vi "justin arc - v1.vi"() -> ()   [LabVIEW 2019]
doc: "This is the interface, the one VI which loads all the others. Run this one first.\n\n(the line below ensures settings are saved)\n[Red Tweezers Save Settings]"
uses:
  justin arc - v1 Folder/Matt Fall 2018 files/Matt working/Red Tweezers Image Processing Final 1-19/subvis/line_trapping.ctl
  justin arc - v1 Folder/Matt Fall 2018 files/Matt working/Red Tweezers Image Processing Final 1-19/subvis/spot.ctl
  <vilib>/userDefined/High Color/IMAQdx.ctl
  justin arc - v1 Folder/Matt Fall 2018 files/Matt working/Red Tweezers Image Processing Final 1-19/subvis/selection_element.ctl
  <vilib>/Analysis/Matrix/Datatypes/RealMatrix.ctl
  justin arc - v1 Folder/Matt Fall 2018 files/Matt working/Red Tweezers Image Processing Final 1-19/subvis/mouse_info.ctl
  <vilib>/Analysis/baseanly.llb/Real A x B.vi
  justin arc - v1 Folder/Matt Fall 2018 files/Matt working/Red Tweezers Image Processing Final 1-19/subvis/red_tweezers_globals_INTERNAL_VOLATILE.vi
  justin arc - v1 Folder/Matt Fall 2018 files/Matt working/Red Tweezers Image Processing Final 1-19/subvis/red_tweezers_globals.vi
  <vilib>/Analysis/Matrix/Numeric/Multiply/Multiply - RM,R.vi
  <vilib>/Analysis/Matrix/Numeric/Multiply/Multiply - R,RM.vi
  <vilib>/Analysis/NI_AALBase.lvlib
  <vilib>/vision/driver/NI_Vision_Acquisition_Software.lvlib
  <vilib>/vision/NI_Vision_Development_Module.lvlib
  <vilib>/Analysis/Matrix/NI_Matrix.lvlib
panel:
  out "Specific Point":cluster{i32, i32}
  out "bottomrx 3":dbl
  out "toply 3":dbl
  out "bottomry 3":dbl
  out "toplx 3":dbl
  out "Circles 2":T1(array[cluster]) {"Position"."Y" format="%.2f"; "Position"."X" format="%.2f"}
  out "Spot Storage":T2[](array[typedef]) {"Amplitude Correction" step=0.1; "Line Trapping"."Phase Gradient" step=0.05; "Line Trapping"."Vector"."x" step=1e-06 format="%#_6p"; "Line Trapping"."Vector"."y" step=1e-06 format="%#_6p"; "Line Trapping"."Vector"."z" step=1e-06 format="%#_6p"; "NA Position"."r" step=1e-06; "NA Position"."y" step=1e-06; "NA Position"."x" step=1e-06; "Position"."z" step=1e-06; "Position"."y" step=1e-06; "Position"."x" step=1e-06; "Phase" step=0.7753; "Intensity" step=0.1}
  out "# selected":i16
  out "Last Pattern":T2[](array[typedef]) {"Amplitude Correction" step=0.1; "Line Trapping"."Phase Gradient" step=0.05; "Line Trapping"."Vector"."x" step=1e-06 format="%#_6p"; "Line Trapping"."Vector"."y" step=1e-06 format="%#_6p"; "Line Trapping"."Vector"."z" step=1e-06 format="%#_6p"; "NA Position"."r" step=1e-06; "NA Position"."y" step=1e-06; "NA Position"."x" step=1e-06; "Position"."z" step=1e-06; "Position"."y" step=1e-06; "Position"."x" step=1e-06; "Phase" step=0.7753; "Intensity" step=0.1}
  out "Plugins":T4(array[cluster])=[{"Name"="ASI Stage", "Folder"=path "C:/Users/Richard Bowman/Dropbox/red_tweezers_1_4_rc4/plugins/ASI Stage.llb", "vi reference"=refnum, "Needs to be run"=TRUE, "Error"={"status"=FALSE, "code"=0, "source"=""}}, {"Name"="iTweezers", "Folder"=path "C:/Users/Richard Bowman/Dropbox/red_tweezers_1_4_rc4/plugins/iTweezers.llb", "vi reference"=refnum, "Needs to be run"=TRUE, "Error"={"status"=FALSE, "code"=0, "source"=""}}, {"Name"="MightexLED", "Folder"=path "C:/Users/Richard Bowman/Dropbox/red_tweezers_1_4_rc4/plugins/MightexLED.llb", "vi reference"=refnum, "Needs to be run"=TRUE, "Error"={"status"=FALSE, "code"=0, "source"=""}}]
  in  "Tab":T5(tab)
  out "Play Pressed":bool
  out "Y":dbl
  out "X":dbl
  in  "O Button":bool
  in  "OK Button":bool
  in  "Bubble Size":dbl=50.0002
  out "Hit Indicator":bool
  in  "On":bool
  out "Induce check":bool
  out "Area+ Buffer":dbl
  in  "Area to check":dbl=0.00025
  out "Prev Current Spot":dbl
  out "spots selected 2":i32=4
  out "Spot # Check":dbl
  out "Orig Y SC":dbl
  out "Orig X SC":dbl
  out "ID num check":dbl
  out "Value Check":dbl
  out "ID":dbl[](array[numeric])
  out "Null array":dbl[](array[numeric])
  out "Potential Collisions":dbl
  out "What to Check":dbl[](array[numeric])
  out "Num":dbl
  out "Old Y":dbl
  out "Old X":dbl
  out "init":dbl
  out "Looper":bool
  in  "Output to SLM":bool
  out "Maximum":dbl
  out "Projected Distance":dbl
  out "Previous Distance":dbl
  out "Group ID #":dbl
  in  "Buffer Zone":dbl=7e-05
  out "# of Spots":dbl
  out "Distance":dbl
  out "Hit":bool
  out "Y Displacement":dbl
  out "X Displacement":dbl
  out "Current Spot #":dbl
  out "spots selected":i32=4
  in  "lock aspect ratio":bool=TRUE
  in  "Size":cluster{"x":dbl, "y":dbl, "z":dbl} {"z" step=1e-06 format="%#_4p"; "y" step=1e-06 format="%#_4p"; "x" step=1e-06 format="%#_4p"}
  in  "phase":dbl step=0.7753
  in  "Vortex Charge":i8
  in  "Intensity":dbl=1.0 step=0.1
  in  "add to selection":bool
  in  "random position":bool
  in  "new spot":bool
  in  "delete":bool
  in  "rotate":bool
  in  "Rotation Axis":u16(ring)=2 items=["Z", "X", "Y", "Custom"]
  in  "Angle (degrees)":dbl=2.0
  in  "Custom Axis":cluster{dbl, dbl, dbl}
  in  "Spot Shape":enum32{"Normal", "Line", "NA", "Mixed"}(tab)=enum."Mixed"
  in  "Line Trapping":T3 {"Phase Gradient" step=0.05; "Vector"."x" step=1e-06 format="%#_4p"; "Vector"."y" step=1e-06 format="%#_4p"; "Vector"."z" step=1e-06 format="%#_4p"}
  in  "Scale back aperture":dbl=1.1 step=0.1
  in  "Scale BA":bool
  in  "Position on back aperture":cluster{"x":dbl, "y":dbl}={"x"=-5.84327907697451e-18, "y"=0.0} {"y" step=0.1 format="%#_4p"; "x" step=0.1 format="%#_4p"}
  in  "Radius on back aperture":dbl=1.1 step=0.1
  in  "Generate":bool
  in  "Pattern":T6(tab)
  in  "Spots across centre":i32=5
  in  "Reference Array?":bool
  in  "Fraction of SLM":dbl=1.0
  in  "Spots across centre":i32=5
  in  "N":cluster{i32, i32}
  in  "spacing/m":dbl=2.0
  in  "Iterations":i32=10
  out "non-uniformity":dbl(slide)=0.031119223416512406 scale=0.0..0.2
  out "efficiency":dbl(slide)=0.8985936267644501 scale=0.0..1.0
  in  "Optimise":bool
  in  "Reset Phase/Amplitude":bool
  in  "Fall-off/m":dbl=0.00025 min=0.0 step=1e-06 format="%#_4p"
  in  "Abort Plugin":bool
  in  "Plugin:":u16(ring)=1
  in  "Save Video":bool
  in  "Global ROI (requires restart)":i32[](array[numeric])=[0, 0, 1280, 512]
  in  "Zoom":bool
  in  "Draw ROI":bool
  in  "Zoom to Fit":bool
  out "Image Information":string="640x480 1.93X 8-bit image 255    (0,0)"
  in  "Camera":T7
  in  "Time per Frame (ms)":dbl
  in  "Edit Sequence Mode":bool
  in  "Manual Edit":bool
  in  "Bubble ID to Empty":dbl
  in  "Clearance Button":bool
  in  "Manual Sequence":bool
  in  "Play Sequence":bool
  in  "Reset":bool
  out "Sequence Instances":dbl
  out "Counter":dbl
  in  "Save State":bool
  out "Sequence On?":bool
  in  "Sequence Order":dbl
  out "Selection/Group":T8[](array[typedef])
  in  "Sequence Storer":T2[][](array[typedef]) {"Amplitude Correction" step=0.1; "Line Trapping"."Phase Gradient" step=0.05; "Line Trapping"."Vector"."x" step=1e-06 format="%#_6p"; "Line Trapping"."Vector"."y" step=1e-06 format="%#_6p"; "Line Trapping"."Vector"."z" step=1e-06 format="%#_6p"; "NA Position"."r" step=1e-06; "NA Position"."y" step=1e-06; "NA Position"."x" step=1e-06; "Position"."z" step=1e-06; "Position"."y" step=1e-06; "Position"."x" step=1e-06; "Phase" step=0.7753; "Intensity" step=0.1}
  in  "Object New Y":dbl
  in  "Object New X":dbl
  in  "Input Object Location":bool
  out "Time Elapsed(ms)":i32
  out "Start":i32
  out "Stop":i32
  out "Insert End":bool
  out "NewXYRates":dbl[][](array[numeric])
  out "NewXYArraySize":dbl
  out "NewXYArray":dbl[][](array[numeric])
  in  "Rates":dbl
  out "LCS Y":dbl
  out "LCS X":dbl
  in  "LCS":dbl
  in  "Play":bool
  out "Initiate Creation 2":dbl
  in  "Max Number of Bubbles 2":dbl
  in  "Number of Planned Sequence Frames 2":dbl
  in  "Add Additional Frames":bool
  in  "Frame Location":dbl
  in  "Additional Frames Wanted":dbl
  in  "Tab Control":enum32{"Line", "Arc"}(tab)
  out "X Rate":dbl
  out "Y Rate":dbl
  out "Original Theta":dbl
  out "Original\nRadius":dbl
  out "Original\nD-Y":dbl
  out "Original\nD-X":dbl
  out "Center Y":dbl
  out "Center X":dbl
  out "Center location":dbl[][](array[numeric])
  out "Degree Rate":dbl
  out "ROI-X":dbl
  out "ROI-Y":dbl
  in  "Lock Current Spot":bool
  out "Locked Current Spot":dbl
  out "Numeric":dbl
  out "probe":dbl
  in  "Insert":bool
  in  "Start at Which Frame?":dbl
  out "Original Y":dbl
  out "Original X":dbl
  in  "Mark Original Position":bool
  in  "How Many Frames?":dbl
  out "New Y":dbl
  out "New X":dbl
  out "Spot Storage 2":T2[](array[typedef]) {"Amplitude Correction" step=0.1; "Line Trapping"."Phase Gradient" step=0.05; "Line Trapping"."Vector"."x" step=1e-06 format="%#_6p"; "Line Trapping"."Vector"."y" step=1e-06 format="%#_6p"; "Line Trapping"."Vector"."z" step=1e-06 format="%#_6p"; "NA Position"."r" step=1e-06; "NA Position"."y" step=1e-06; "NA Position"."x" step=1e-06; "Position"."z" step=1e-06; "Position"."y" step=1e-06; "Position"."x" step=1e-06; "Phase" step=0.7753; "Intensity" step=0.1}
  in  "Numeric 2":dbl
  in  "Save":bool
  in  "Load":bool
  out "Current Y":dbl
  out "Current X":dbl
  out "Calc New  Y":dbl
  out "Calc New X":dbl
  out "distance bw y and rad":dbl
  out "distance  bw x and rad":dbl
  out "Object Y":dbl
  out "Object X":dbl
  in  "Camera Capture 2":bool
  out "Object y":dbl
  out "Object x":dbl
  out "Number of Matches Returned 2":dbl
  out "bottomry 2":dbl
  out "toply 2":dbl
  out "bottomrx 2":dbl
  out "toplx 2":dbl
  in  "Send Data":bool
  out "Camera 3":T9(plugin-control)
  in  "Circle Descriptor 2":cluster{"Min Radius":dbl, "Max Radius":dbl}={"Min Radius"=3.0, "Max Radius"=500.0}
  out "Video Frame Rate":dbl(knob)=50.00000000000003 scale=0.0..100.0 scale format="%.1f"
  out "Interface Frame Rate":dbl(knob)=97.23240312927678 scale=0.0..100.0 scale format="%.1f"
  in  "stop":bool=TRUE
  out "Numeric 4":dbl
  in  "Position":cluster{"x":dbl, "y":dbl, "z":dbl}={"x"=1e-06, "y"=-6.3e-06, "z"=0.0} {"z" step=1e-06 format="%#_4p"; "y" step=1e-06 format="%#_4p"; "x" step=1e-06 format="%#_4p"}
  out "Numeric 3":dbl
  out "ROI 1":T10
  out "ROI 0":T10
  out "MOP pressed":bool
  out "MOP pressed After":bool
  out "X Pos every 10 sec":dbl
  out "Elapsed Time":dbl
  out "Position Indicator":string
  out "Spot Checker":T2[](array[typedef]) {"Amplitude Correction" step=0.1; "Line Trapping"."Phase Gradient" step=0.05; "Line Trapping"."Vector"."x" step=1e-06 format="%#_6p"; "Line Trapping"."Vector"."y" step=1e-06 format="%#_6p"; "Line Trapping"."Vector"."z" step=1e-06 format="%#_6p"; "NA Position"."r" step=1e-06; "NA Position"."y" step=1e-06; "NA Position"."x" step=1e-06; "Position"."z" step=1e-06; "Position"."y" step=1e-06; "Position"."x" step=1e-06; "Phase" step=0.7753; "Intensity" step=0.1}
  out "Image":T9(plugin-control)
  # "Notes:\n\nIf you are doing non-sequence controls,\nthe delete function can be used as intended.\nHowever, do not use the delete function after\nrunning a sequence! Using it will prevent\nthe bubbles from appearing as the\nnumber of spots will change, which is\nessential for the sequence to work (it would\nbe displaying the maximum number of\nbubbles). \n\nIf you happen to delete a bubble, it can be \nrestored by inserting a new spot. Once enough\nspots have been restored, click on manual edit\nto correct the # of spots tracker. It should \nbe restored to where it originally was."
  # "The SLM can be used to shape spots; here you can restrict the NA of a spot (so it comes only from part of the back aperture), or create a line-trap"
  # "The traps do not have any spot-shaping applied (so they should just be diffraction-limited focal spots)."
  # "This shapes the amplitude (and phase) of the beam to create extended line traps.  The \"Phase Gradient\" control allows the Poynting vector to push things along the line.  Unfortunately, some work is needed on the scaling factors so the phase gradient control will need tweaking if the line trap has a nonzero z component."
  # "By default,each spot comes from the whole back aperture.  Here, you can limit a spot to come from a specific part of the back aperture."
  # "The control below allows you to scale the whole back aperture (i.e. the position and size of all the apertures).  It's a one-time operation, i.e. only changes things when you push \"ok\"."
  # "A Combination of line-trapping and NA restriction has been applied to these traps.  You can get at the line trap or NA parameters on the other tabs, switching to the NA tab does not delete the line-trap settings."
  # "This tab generates Shack-Hartmann type holograms, which are often useful when aligning the system, and arrays of spots."
  # "The controls above only work when using the \"IMAQdx with ROI Buttons\" case in the bottom loop.  You can save video regardless of camera code though."
  # "Manual Edit allows a user to\ngo to a specific sequence frame."
  # "To clear the sequence, you must\nclear the array. Right click on sequence\nstorer to do this."
  # "Use this to \"clear\" a \nspecific bubble. If\nworking on a sequence,\nuse this as your delete\nbutton! You can update\nthe view by using manual edit."
  # "Use the reset button\nto clear counter.\nIt becomes necessary\nwhen you clear the array,\nespecially in manual mode."
  # "Use the sequence creator tab to specify the\nnumber of bubbles you want along with\nthe number of frames.\n\nTo save at a specific interval, the sequence\norder can be used to place the state. If used\nto correct something, it will replace the\nentire sequence frame.\n\n\"Sequence On?\" is only used in auto mode."
  # "Multiple bubbles can  be done with the\nline function. One bubble at a time for the arc\nfunction."
  # "Using the Load/Save function:\n\nRed Tweezers itself is unable to save long \nsequences, but a separate program is able to\naccomplish this. To do this, follow these\nsteps:\n\n1. After creating your sequence, press the save\nbutton below.\n\n2. Then, go to the subvi folder and find\nSequenceSaver.vi.\n\n3. At the control \"Sequence Storer,\" right-click\nthe dimensions part of the array and go to\ndata operations.\n\n4. Press \"Make Current Values Default\" and save\nthe sequence.\n\n5. The next time you load the program, simply\npress load to re-acquire the sequence. You\nwill need to insert the bubbles again, but after\nthe first frame can be recovered by using\nSequenceControl.vi."
types:
  T1 = cluster{"Position":cluster{"X":sgl, "Y":sgl}, "Radius":dbl, "Score":dbl}[]
  T2 = typedef "spot.ctl" = cluster{"Position":cluster{"x":dbl, "y":dbl, "z":dbl}, "Intensity":dbl, "Vortex Charge":i8, "Phase":dbl, "NA Position":cluster{"x":dbl, "y":dbl, "r":dbl}, "Line Trapping":T3, "Amplitude Correction":dbl}
  T3 = typedef "line_trapping.ctl" = cluster{"Vector":cluster{"x":dbl, "y":dbl, "z":dbl}, "Phase Gradient":dbl}
  T4 = cluster{"Name":string, "Folder":path, "vi reference":refnum<vi>, "Needs to be run":bool, "Error":errorcluster}[]
  T5 = enum32{"Current Spot", "Rotate", "Spot Shape", "Patterns", "Plugins", "Video", "Sequence", "Sequence Creator", "Spot Control", "Load/Save", "Image Process"}
  T6 = enum32{"HCP Shack-Hartmann", "Square Shack-Hartmann", "Rectangular Grid"}
  T7 = typedef "IMAQdx.ctl" = refnum<k21>
  T8 = typedef "selection_element.ctl" = cluster{"Group ID":i32, "Selected":bool}
  T9 = typedef "IMAQ Image.ctl" = refnum<image>
  T10 = typedef "NI_Matrix.lvlib/RealMatrix.ctl" = dbl[][]
  T11 = typedef "mouse_info.ctl" = cluster{"Button Down":bool, "Dragging":bool, "Position (Image Pixels)":cluster{"X":dbl, "Y":dbl}, "Previous Position (Image Pixels)":cluster{"X":dbl, "Y":dbl}, "Button":u16, "Mods":cluster{"Double Click":bool, "Menu Key":bool}, "PlatMods":cluster{"Shift":bool, "Ctrl":bool, "Alt":bool, "Cmd":bool, "Opt":bool}}
  T12 = cluster{"Desired Font (Application)":enum16{"User-specified Font", "Application Font", "System Font", "Dialog Font"}, "[User-specified Font]":cluster{"Font Name":string, "Size":i16, "Strikeout?":bool, "Italic?":bool, "Underline?":bool, "Outline?":bool, "Shadow?":bool, "Bold?":bool, "Rotation Angle":dbl}, "Horizontal Alignment":i16, "Vertical Alignment":i16}
  T13 = cluster{"Position":cluster{"x":dbl, "y":dbl, "z":dbl}, "Intensity":dbl, "Vortex Charge":i8, "Phase":dbl, "NA Position":cluster{"x":dbl, "y":dbl, "r":dbl}, "Line Trapping":T3, "Amplitude Correction":dbl}
  T14 = enum16{"Set guide visibility", "Set grid visibility", "Show front panel", "Render on image"}
  T15 = enum32{"Current Spot", "Rotate", "Spot Shape", "Patterns", "Plugins", "Video"}
  T16 = enum16{"Left Button", "Center Button", "Right Button", "Window Close"}
  T17 = typedef "Image Type" = u32
  T18 = cluster{"number: 0 to 1":dbl, "number: 0 to 1":dbl}
  T19 = typedef "overlay_element.ctl" = cluster{"Tool":enum16{"Lines", "Oval", "Rectangle", "Text"}, "Points":cluster{"X":dbl, "Y":dbl}[], "Drawing Mode":u32, "Color":u32, "String":string}
  T20 = enum32{"Current Spot", "Rotate", "Spot Shape", "Patterns", "Plugins", "Video", "Particle Tracking", "Clamping", "Blank"}[]
  T21 = typedef "LVMenuShortCut.ctl" = cluster{"include Shift key?":bool, "include Ctrl key?":bool, "shortcut key":string}
  T22 = typedef "LVPoint32TypeDef.ctl" = cluster{"Horizontal":i32, "Vertical":i32}
  T23 = cluster{"Shift":bool, "Ctrl":bool, "Alt":bool, "Cmd":bool, "Opt":bool}
  T24 = cluster{"Button Down":bool, "Dragging":bool, "Mouse Coords (image pixels)":cluster{dbl, dbl}, "Mouse Coords (image pixels)":cluster{dbl, dbl}, "Button":u16, "Mods":cluster{"Double Click":bool, "Menu Key":bool}, "PlatMods":cluster{"Shift":bool, "Ctrl":bool, "Alt":bool, "Cmd":bool, "Opt":bool}}
  T25 = cluster{"Position":cluster{"X":sgl, "Y":sgl}, "Radius":dbl, "Score":dbl}
  T26 = cluster{"Global Rectangle":i32[], "Contours":cluster{"Contour Type":u32, "ROI Type":u32, "Points":i32[]}[]}
  T27 = cluster{"Contour Type":u32, "ROI Type":u32, "Points":i32[]}[]
  T28 = cluster{"Contour Type":u32, "ROI Type":u32, "Points":i32[]}
  T29 = cluster{"[0]":dbl, "[1]":dbl, "[2]":dbl, "[3]":dbl}
  T30 = cluster{"NewXYArray[0]":dbl, "NewXYArray[1]":dbl, "NewXYArray[2]":dbl, "NewXYArray[3]":dbl, "NewXYArray[4]":dbl, "NewXYArray[5]":dbl, "NewXYArray[6]":dbl, "NewXYArray[7]":dbl, "NewXYArray[8]":dbl}
  T31 = cluster{"Average Frame Time":dbl, "millisecond timer value":u32}
  T32 = cluster{"Position":cluster{"x":dbl, "y":dbl, "z":dbl}, "Intensity":dbl, "Vortex Charge":i8, "Phase":dbl, "NA Position":cluster{"x":dbl, "y":dbl, "r":dbl}, "Line Trapping":T3, "Amplitude Correction":dbl}[]
  T33 = enum32{"Bad", "Idle", "Run top level", "Running"}
  T34 = typedef "AviRefnum.ctl" = refnum<k1>
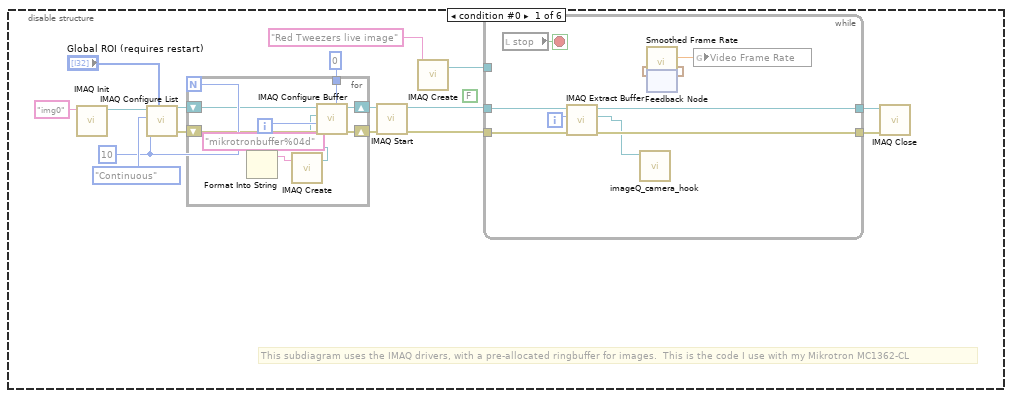
[diagram p3: hidden frame]
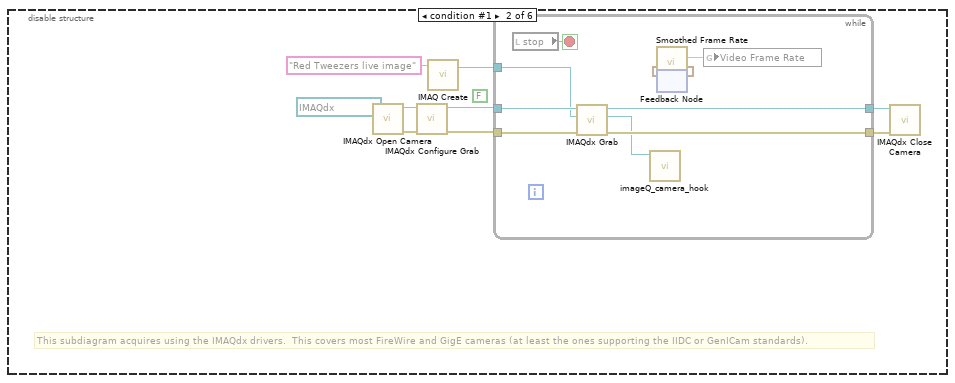
[diagram p4: hidden frame]
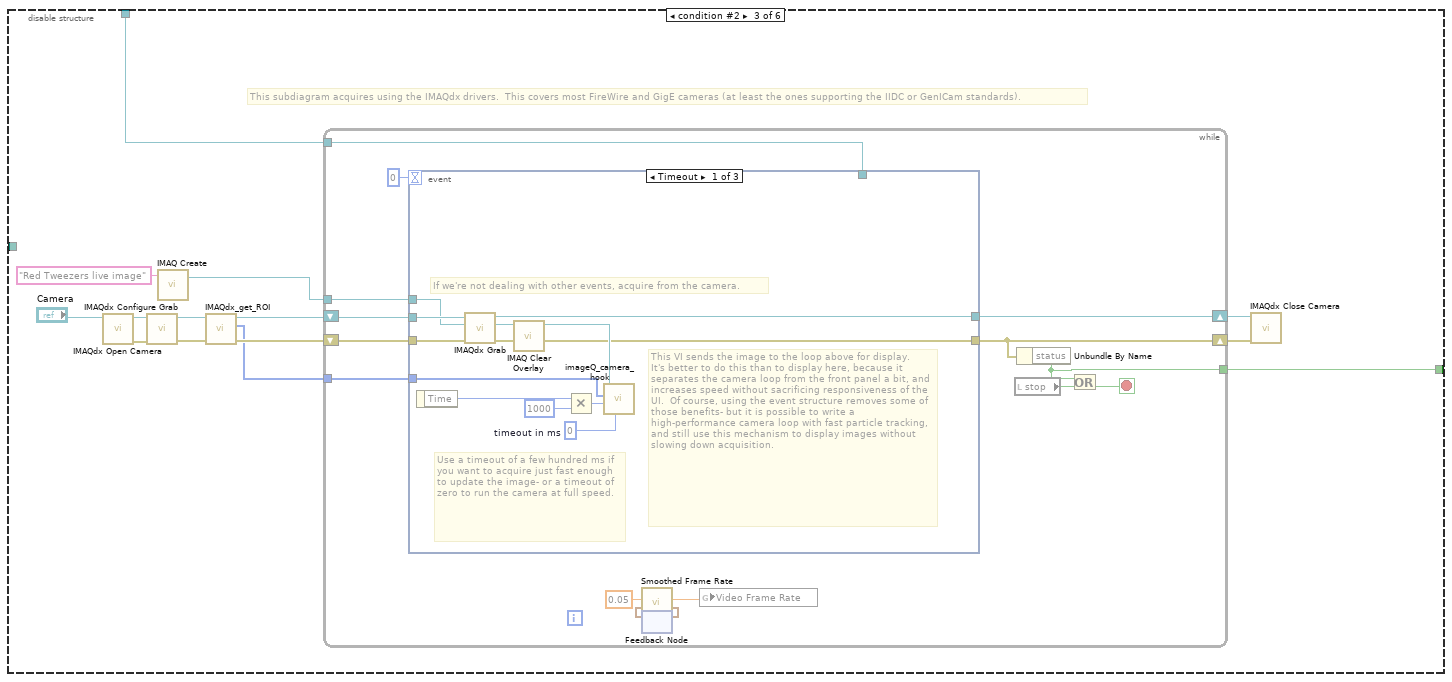
[diagram p5: hidden frame]
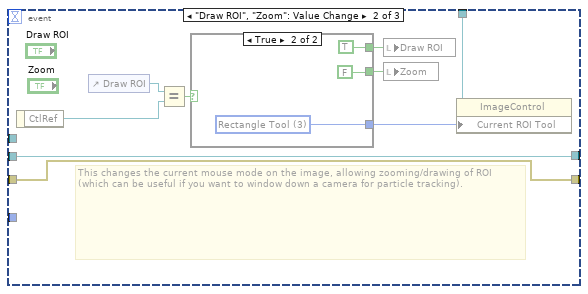
[diagram p6: hidden frame]
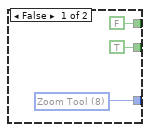
[diagram p7: hidden frame]
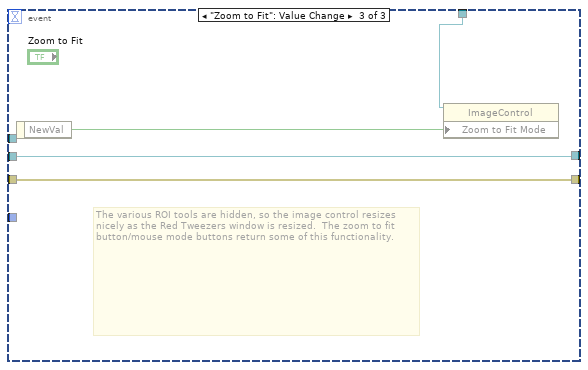
[diagram p8: hidden frame]
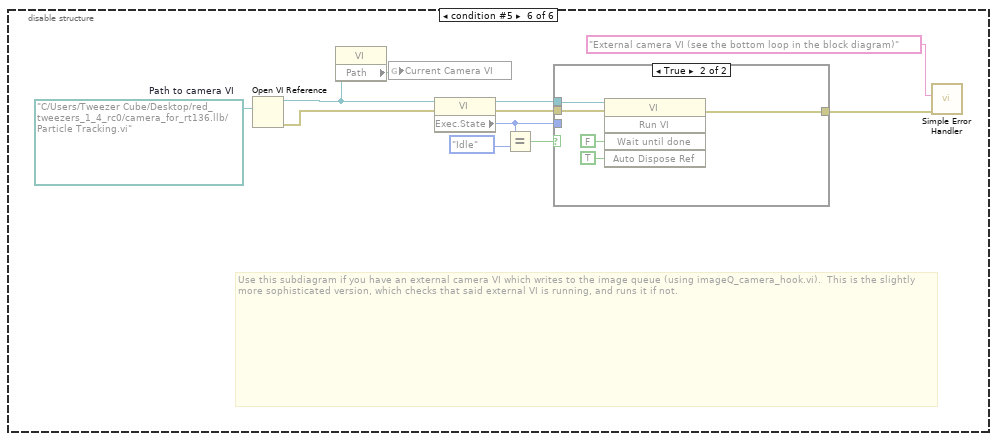
[diagram p10: hidden frame]
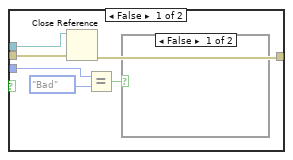
[diagram p11: hidden frame]
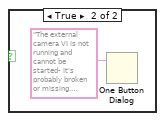
[diagram p12: hidden frame]
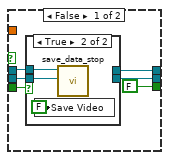
[diagram p13: hidden frame]
diagram:
  w11 = "red_tweezers_display_imageQ" ("Queue Name")
  w23 = T11 {"Button Down"=FALSE, "Dragging"=FALSE, "Position (Image Pixels)"={"X"=0.0, "Y"=0.0}, "Previous Position (Image Pixels)"={"X"=0.0, "Y"=0.0}, "Button"=0, "Mods"={"Double Click"=FALSE, "Menu Key"=FALSE}, "PlatMods"={"Shift"=FALSE, "Ctrl"=FALSE, "Alt"=FALSE, "Cmd"=FALSE, "Opt"=FALSE}}  # Mouse Information
  w24 = refnum<vi> refnum  # Image
  # "The funny looking feedback-node structure is deliberate (if odd).  We want to reload settings from the last used file (stored in the registry) only if this program has not been run since it was last loaded from file/recompiled.  That's why I use an uninitialised shift register: every time the program runs, it increments.  So, if it is zero, this is our first run (or we've been recently recompiled)."
  # "This loop handles the video that is displayed on-screen and saved to file."
  # "Initially, we only register to be told when the user clicks the image"
  # "This is the actual image control"
  # "This is a generic reference.\nIt is just a placeholder, so we can register for events later."
  # "This version of red tweezers uses two coordinate systems: \n1. Real Coordinates - corresponding to physical distances in 3D in microns\n2. Image Coordinates - position on the camera image, relative to the top left of the CURRENT ROI, measured in pixels. If the ROI changes, the relationship between \"real units\" and \"image pixels\" may change, so all values should be stored and presented to the user in REAL units unless there is a good reason to do otherwise."
  n1 = control-ref of="Plugin Pnl"() -> (w20:refnum<vi>)
  n2 = flat-sequence {
    tunnel: [w27] -> w6
    tunnel: w4 -> [_]
    frame #0 {
      n3 = vi-ref "red_tweezers_globals_INTERNAL.vi"() -> (w28:refnum<vi>)
      n4 = property class="VI"(reference=w28) -> ("Path"=w27:path)  [unwired: 1 in, 2 out]
      n5 = global write "red_tweezers_globals_INTERNAL_VOLATILE.vi" "Current Camera VI"(w27) -> ()
    }
  }
  n6 = control-ref of="Plugin:"() -> (w21:refnum<vi>)
  n7 = feedback #1() -> (w14:dbl)  [unwired: 1 in]
  n8 = Equal To 0?(x=w14) -> (x = 0?=w13:bool)
  n9 = Increment(x=w14) -> (x+1=w12:dbl)
  n10 = feedback-in #1(w12) -> ()
  n11 = call "plugins_load.vi"("Sub Panel"=w20, "Plugin Chooser"=w21) -> ("error out"=w15:errorcluster, "Plugins"=w17:T4)  [unwired: 2 in, 2 out]
  "Plugins" <- w17
  n12 = control-ref of="Image"() -> (w5:refnum<vi>)
  n13 = case shown="True" w13 {
    tunnel: w15 -> [_ w29]
    tunnel: [_ w29] -> w4
    frame False {
    }
    frame True {
      n14 = call "settings_load_default_file.vi"("error out"=w29) -> ()
    }
  }
  n15 = flat-sequence {
    tunnel: w4 -> [_]
    tunnel: w2 -> [w31]
    frame #0 {
      # "ensure we don't accidentally start saving video, and run UDP Sender to set up the hologram window."
      n16 = local write "Save Video"(FALSE ("background subtraction")) -> ()
      n17 = call "UDP Sender generic_2.vi"("Spots"=w31) -> ()  [unwired: 2 in, 1 out]
    }
  }
  n18 = global read "red_tweezers_globals.vi" "Selection/Group"() -> (w22:T8[])
  n19 = register-events(w5, w24, w24, w24) -> (reference out=w25:refnum<event-registration>)  [unwired: 2 in, 1 out]
  n20 = global read "red_tweezers_globals.vi" "Spots"() -> (w2:T2[])
  n21 = local write "stop"(FALSE ("STOP")) -> ()
  n22 = call "ensure_selection_matches_spots.vi"("Selection and Groups in"=w22, "Spots"=w2) -> ("Selection and Groups out"=w26:T8[], "Spots (duplicate)"=w1:T2[])  [unwired: 4 in]
  n23 = call "IMAQ Create"("Image Name"=w11) -> ("New Image"=w9:T9)  [unwired: 4 in, 1 out]
  n24 = call "imageQ_create_return_queue.vi"("Queue Name"=w11) -> ("queue out"=w10:refnum<queue>)
  n25 = while {
    shift-right: [w141] -> _
    shift-left: w1 -> [w161]
    shift-right: [w160] -> _
    shift-left: w26 -> [w159]
    shift-right: [w163] -> _
    shift-left: _ -> [w154]
    shift-right: [w162] -> _
    shift-left: _ -> [w153]
    tunnel: w5 -> [w158]
    shift-right: [w152] -> _
    shift-left: w23 -> [w151]
    shift-right: [w155] -> _
    shift-left: w25 -> [w156]
    border: errorcluster {"status"=FALSE, "code"=0, "source"=""} ("error out") -> [_]
    tunnel: [errorcluster {"status"=FALSE, "code"=0, "source"=""} ("error in (no error)")] -> w18
    border: w17 -> [_]
    tunnel: w1 -> [w142]
    stop <- w143 stop-if-true
    w59 = 7 items=["Red", "Green", "Blue", "Hue", "Saturation", "Luminance", "Value", "Intensity"] ("Color Plane")
    w61 = T17 0 items=["Grayscale (U8)", "Grayscale (I16)", "Grayscale (SGL)", "Complex (CSG)", "RGB (U32)", "HSL (U32)", "RGB (U64)", "Grayscale (U16)"] ("Image Type")
    # "ARRAY INICATORS ARE HIDDEN ON THE FRON PANNEL"
    # "CYCLE THROUGH THE NUMBERS ie. 0-6 \nFOR THE CASE OF 6 COORDINATES\nCURRENT CASE HAS 2 SETS OF COORDINATES"
    # "CASE STRUCTURE TO PLACE CODE INTO THE ARRAY"
    # "This is the calculation for the center of the detected circle, not sure where to put for now"
    # "This Play Function inserts bubbles from a given .mat file into the sequence storer"
    # "The function inserts the newly generated sequence for the automatic sequence generator. It also contains the code\nthe code necessary to check whether the bubbles will intersect with each other in the sequence."
    # "This calculates the size of the area including the buffer zone length.\nThe bubble diameter will also be included in the near future."
    # "The statement to the right controls the area that are being chcecked and checks\nwhich bubbles need to be checked.  There are two instances where this activates\nin this case:\n\nWhen a new bubble is selected\nWhen a bubble is deselected, reverting to the last current spot #\n\nThe other case, when the bubble moves out of the area specified, is located\ninside the while loop controlling the bubble movement with a mouse."
    # "Timer function example"
    # "These functions help with the calculations for the sequence generator."
    # "This loads the sequence from the \"saver\" VI. The save function below \"saves\" the sequence into the saver VI."
    # "The VI above is SequenceSaver.vi which contains the\ncode necessary to create a sequence."
    # "This case structure is the Save State structure. This stores\nthe current state of the bubbles (ie position)."
    # "Reset sets the counter back to zero. This is particularly useful \nwhen using the manual sequence."
    # "This case structure helps to continue the sequence.\nThis takes the true case of the Sequence On? function\nor the true case for the Manual Sequence function\nin order to go to the next sequence frame."
    # "This case structure allows for the playing of the sequence.\nThe amount of time it takes to go through the sequence\ncan be edited on the current spot menu."
    # "We only write to the image overlay when we are in one of the tabs, to prevent it disappearing when we are (for example) using the mouse."
    # "These wires control saving undo info. See the VI below's tip strips for details."
    # "Setting these wires to false means:\n(1) dragging moves the selection\n(2) clicking spots changes selection\nset them to true to stop the default mouse behaviour, don't wire them straight through!"
    n26 = event shown="[0] Timeout" {
      selector: w156 -> [w633 w1304 w1309 w1531 w1559 w1576 w1673 _]
      dyn-events: [w633 w1303 w1309 w1529 w1556 w1577 w1673 _] -> w155
      timeout: 0 -> [_ _ _ _ _ _ _ _]
      tunnel: [w641 _ w1311 w1526 w1561 w1568 w1660 _] -> w163
      tunnel: [w640 _ w1310 w1525 w1560 w1567 w1664 _] -> w162
      tunnel: [w639 _ _ _ _ _ _ _] -> w114
      tunnel: w161 -> [w638 w1299 w1316 w1521 w1554 w1573 w1668 w1991]
      tunnel: [w637 w1299 w1314 w1521 w1554 w1564 w1666 w1991] -> w149
      tunnel: [w636 w1298 w1313 w1510 w1553 w1574 w1656 w1990] -> w148
      tunnel: w159 -> [w635 w1298 w1315 w1510 w1553 w1572 w1667 w1990]
      tunnel: w158 -> [w634 w1300 w1306 w1520 w1557 w1575 w1669 _]
      tunnel: [w632 _ w1308 w1530 T11 {"Button Down"=FALSE, "Dragging"=FALSE, "Position (Image Pixels)"={"X"=0.0, "Y"=0.0}, "Previous Position (Image Pixels)"={"X"=0.0, "Y"=0.0}, "Button"=0, "Mods"={"Double Click"=FALSE, "Menu Key"=FALSE}, "PlatMods"={"Shift"=FALSE, "Ctrl"=FALSE, "Alt"=FALSE, "Cmd"=FALSE, "Opt"=FALSE}} T11 {"Button Down"=FALSE, "Dragging"=FALSE, "Position (Image Pixels)"={"X"=0.0, "Y"=0.0}, "Previous Position (Image Pixels)"={"X"=0.0, "Y"=0.0}, "Button"=0, "Mods"={"Double Click"=FALSE, "Menu Key"=FALSE}, "PlatMods"={"Shift"=FALSE, "Ctrl"=FALSE, "Alt"=FALSE, "Cmd"=FALSE, "Opt"=FALSE}} w1672 _] -> w152
      tunnel: w151 -> [w632 _ w1308 _ _ w1571 w1663 _]
      tunnel: w154 -> [_ _ w1311 w1526 w1561 w1568 w1660 _]
      tunnel: w153 -> [_ _ w1310 w1525 w1560 w1567 w1664 _]
      tunnel: [w631 _ _ _ _ _ _ _] -> w150
      tunnel: [_ _ w1307 _ _ _ TRUE _] -> w147
      tunnel: [_ _ _ TRUE TRUE TRUE FALSE _] -> w146
      tunnel: [TRUE _ _ _ _ _ _ _] -> w144
      tunnel: [_ _ _ _ _ _ _ "stop"] -> w143
      tunnel: w142 -> [_ _ _ _ _ _ w1657 _]
      event Timeout {
        n27 = event-data() -> ()  [unwired: 1 in, 1 out]
        n28 = case shown="\"Current Spot\", Default" "Tab" {
          tunnel: [w656 w924 w1071 w1173 w1254 w1292] -> w637
          tunnel: w638 -> [w653 w926 w1072 w1175 w1254 w1292]
          tunnel: w635 -> [w642 w925 w1069 w1174 w1253 w1291]
          tunnel: [w655 w923 w1070 w1172 w1253 w1291] -> w636
          tunnel: [w643 _ TRUE _ _ _] -> w641
          tunnel: [w643 _ _ _ _ _] -> w640
          tunnel: [_ _ _ FALSE _ _] -> w639
          tunnel: w634 -> [_ _ _ _ _ w1288]
          tunnel: w632 -> [_ _ w1051 _ _ _]
          tunnel: [_ _ w1053 _ _ _] -> w631
          frame "Current Spot", Default {
            w643 = FALSE
            # "The function below contains the code necessary to use the automatic sequence generator to create specific movements. It also helps translate cases where the point is entered in not dragged.\nThis prevents bubbles from intersecting if the bubble is told not to intersect."
            # "If it's out of date, update front panel"
            n29 = call "find_centroid.vi"("Selection and Groups"=w642, "Spots"=w653) -> ("Mean Values"=w651:T2, "size"=w645:cluster{"x":dbl, "y":dbl, "z":dbl}, "centroid"=w646:cluster{"x":dbl, "y":dbl, "z":dbl}, "# selected"=w644:i16)  [unwired: 2 in, 1 out]
            n30 = stacked-sequence {
              tunnel: w644 -> [_ w658]
              frame #0 {
                n31 = local read "spots selected"() -> (→"spots selected 2":i32)
              }
              frame #1 {
                "spots selected" <- w658
              }
            }
            n32 = feedback-in #2(w651) -> ()
            n33 = feedback #2() -> (w652:T2)  [unwired: 1 in]
            n34 = feedback #3() -> (w650:cluster{"x":dbl, "y":dbl, "z":dbl})  [unwired: 1 in]
            n35 = feedback-in #3(w645) -> ()
            n36 = Not Equal?(x=w652, y=w651) -> (x != y?=w649:bool)
            n37 = Not Equal?(x=w650, y=w645) -> (x != y?=w648:bool)
            n38 = Or(x=w649, y=w648) -> (x .or. y?=w647:bool)
            n39 = case shown="True" w647 {
              tunnel: w651 -> [_ w664]
              tunnel: w645 -> [_ w660]
              frame False {
              }
              frame True {
                n40 = Unbundle By Name(w664) -> ("Position"=w659:cluster{"x":dbl, "y":dbl, "z":dbl}, "Intensity"=w662:dbl, "Vortex Charge"=w661:i8, "Phase"=w663:dbl)
                n41 = local write "Size"(w660) -> ()
                n42 = local write "Vortex Charge"(w661) -> ()
                n43 = local write "Intensity"(w662) -> ()
                n44 = local write "Position"(w659) -> ()
                n45 = local write "phase"(w663) -> ()
                n46 = Unbundle By Name(w659) -> ()  [unwired: 2 out]
              }
            }
            n47 = local write "Selection/Group"(w642) -> ()
            n48 = event shown="[0] Timeout" {
              selector: _ -> [_ _ _ _ _ _ _ _]
              dyn-events: _ -> [_ _ _ _ _ _ _ _]
              timeout: 10 -> [_ _ _ _ _ _ _ _]
              tunnel: w653 -> [w666 w670 w684 w707 w811 w856 w882 w905]
              tunnel: w642 -> [w665 w669 w687 w714 w798 w853 w879 w903]
              tunnel: [w666 w668 w685 w706 w799 w854 w880 w904] -> w656
              tunnel: [w665 w667 w686 w714 w798 w853 w879 w903] -> w655
              tunnel: w646 -> [_ _ _ _ w810 _ _ _]
              event Timeout {
                n49 = event-data() -> ()  [unwired: 3 out]
              }
              event "delete": Value Change {
                n50 = event-data() -> ()  [unwired: 7 out]
                n51 = call "delete_selected_spots.vi"("Selection/Group 3"=w669, "Spots 3"=w670) -> ("Selection/Group 2"=w667:T8[], "Spots 2"=w668:T2[])  [unwired: 4 in]
              }
              event "new spot": Value Change {
                # "If we're not adding it to the selection, de-select all the other spots"
                n52 = event-data() -> ()  [unwired: 7 out]
                n53 = call "coords_ROI_currentimage.vi"() -> ("Mono ROI"=w671:i32[])
                n54 = case shown="False" "add to selection" {
                  tunnel: w687 -> [w700 w705]
                  tunnel: [w699 w705] -> w682
                  frame False {
                    n55 = for {
                      tunnel: w700 -> [w703] mode=indexing
                      tunnel: [w704] -> w699 mode=indexing
                      n56 = Unbundle(w703) -> ("Group ID"=w702:i32)  [unwired: 1 out]
                      n57 = Bundle(cluster=w703, "Group ID"=w702, "Selected"=FALSE ("Label.Visible")) -> (w704:T8)
                    }
                  }
                  frame True {
                  }
                }
                n58 = Index Array(array=w671) -> (element #1=w677:i32, element #2=w678:i32, element #3=w676:i32, element #4=w675:i32)  [unwired: 4 in]
                n59 = Bundle("Numeric"=w677, "Numeric"=w678) -> (w672:cluster{"Numeric":i32, "Numeric":i32})  [unwired: 1 in]
                n60 = Bundle("Numeric"=w676, "Numeric"=w675) -> (w674:cluster{"Numeric":i32, "Numeric":i32})  [unwired: 1 in]
                n61 = Subtract(x=w674, y=w672) -> (x-y=w673:cluster{"Numeric":i32, "Numeric":i32})
                n62 = case shown="True" "random position" {
                  tunnel: [w689 w695] -> w680
                  tunnel: w673 -> [_ w691]
                  tunnel: w672 -> [_ w690]
                  frame False {
                    n63 = call "replace_position.vi"("Position"=cluster{"x":dbl, "y":dbl, "z":dbl} {"x"=0.0, "y"=0.0, "z"=0.0}) -> ("Spot"=w689:T2)  [unwired: 1 in, 2 out]
                  }
                  frame True {
                    n64 = Random Number (0-1)() -> (number: 0 to 1=w697:dbl)
                    n65 = Random Number (0-1)() -> (number: 0 to 1=w698:dbl)
                    n66 = Bundle("number: 0 to 1"=w698, "number: 0 to 1"=w697) -> (w696:T18)  [unwired: 1 out]
                    n67 = Multiply(x=w696, y=w691) -> (x*y=w693:cluster{dbl, dbl})
                    n68 = Add(x=w693, y=w690) -> (x+y=w692:cluster{dbl, dbl})
                    n69 = call "coords_image_to_real_currentimage.vi"("Position (pixels on image)"=w692) -> ("Position (real coords)"=w694:cluster{dbl, dbl, "Z":dbl})  [unwired: 9 in]
                    n70 = call "replace_position.vi"("Position"=w694) -> ("Spot"=w695:T2)  [unwired: 1 in, 2 out]
                  }
                }
                n71 = Build Array (concatenate)(w684, w680) -> (w685:T2[])
                n72 = Build Array (concatenate)(w682, cluster{i32, "Label.Visible":bool} {0, "Label.Visible"=TRUE}) -> (w686:T8[])
              }
              event "Position": Value Change {
                # "If the position has changed, translate the spots"
                n73 = event-data() -> ("OldVal"=w712:cluster{"x":dbl, "y":dbl, "z":dbl}, "NewVal"=w713:cluster{"x":dbl, "y":dbl, "z":dbl})  [unwired: 5 out]
                n74 = flat-sequence {
                  tunnel: w714 -> [w718]
                  tunnel: w711 -> [w717]
                  tunnel: w707 -> [w716]
                  tunnel: [w715] -> w708
                  frame #0 {
                    n75 = for {
                      tunnel: w716 -> [w723] mode=indexing
                      tunnel: w718 -> [w720] mode=indexing
                      tunnel: [w722] -> w715 mode=indexing
                      tunnel: w717 -> [w721]
                      n76 = Unbundle(w720) -> ("Selected"=w719:bool)  [unwired: 1 out]
                      n77 = case shown="True" w719 {
                        tunnel: w723 -> [w724 w729]
                        tunnel: [w724 w728] -> w722
                        tunnel: w721 -> [_ w725]
                        frame False {
                        }
                        frame True {
                          n78 = call "extract_position.vi"("Spot"=w729) -> ("Position"=w726:cluster{"x":dbl, "y":dbl, "z":dbl})
                          n79 = Add(x=w726, y=w725) -> (x+y=w727:cluster{"x":dbl, "y":dbl, "z":dbl})
                          n80 = call "replace_position.vi"("Position"=w727, "Spot in"=w729) -> ("Spot"=w728:T2)  [unwired: 2 out]
                        }
                      }
                    }
                  }
                }
                n81 = Subtract(x=w713, y=w712) -> (x-y=w711:cluster{"x":dbl, "y":dbl, "z":dbl})
                n82 = local read "# of Spots"() -> (w710:dbl)
                n83 = stacked-sequence {
                  tunnel: w707 -> [_ w734 _]
                  tunnel: w708 -> [_ w733 _]
                  tunnel: w710 -> [_ w732 _]
                  tunnel: [_ _ w781] -> w709
                  tunnel: w708 -> [_ _ w780]
                  tunnel: w707 -> [_ _ w779]
                  tunnel: [_ _ w778] -> w706
                  frame #0 {
                    n84 = local write "Looper"(FALSE) -> ()
                    "init" <- 0
                  }
                  frame #1 {
                    n85 = for {
                      N: w732 -> [_]
                      tunnel: w734 -> [w739]
                      tunnel: w733 -> [w744]
                      stop <- w745 stop-if-true
                      n86 = local read "init"() -> (w738:dbl)
                      n87 = Index Array(array=w744, index=w738) -> (element=w743:T2)
                      n88 = Index Array(array=w739, index=w738) -> (element=w737:T2)
                      n89 = Unbundle By Name(w743) -> ("Position.x"=w742:dbl, "Position.y"=w741:dbl)
                      n90 = local read "# of Spots"() -> (w740:dbl)
                      n91 = Unbundle By Name(w737) -> ("Position.x"=→"Old X":dbl, "Position.y"=→"Old Y":dbl)
                      n92 = local write "New X"(w742) -> ()
                      n93 = local write "New Y"(w741) -> ()
                      n94 = stacked-sequence {
                        tunnel: w739 -> [w750 _]
                        tunnel: w742 -> [w749 _]
                        tunnel: w741 -> [w748 _]
                        tunnel: w740 -> [w747 _]
                        tunnel: w738 -> [w746 _]
                        frame #0 {
                          n95 = for {
                            N: w747 -> [_]
                            tunnel: w750 -> [w772]
                            tunnel: w749 -> [w771]
                            tunnel: w748 -> [w769]
                            tunnel: w746 -> [w754]
                            i -> [w756]
                            stop <- w755 stop-if-true
                            n96 = Index Array(array=w772, index=w756) -> (element=w773:T2)
                            n97 = Unbundle By Name(w773) -> ("Position.x"=w770:dbl, "Position.y"=w768:dbl)
                            n98 = Subtract(x=w771, y=w770) -> (x-y=w767:dbl)
                            n99 = Subtract(x=w769, y=w768) -> (x-y=w766:dbl)
                            n100 = Square(x=w767) -> (x^2=w765:dbl)
                            n101 = Square(x=w766) -> (x^2=w764:dbl)
                            n102 = local read "# of Spots"() -> (w758:dbl)
                            n103 = Add(x=w765, y=w764) -> (x+y=w763:dbl)
                            n104 = local read "Buffer Zone"() -> (w753:dbl)
                            n105 = Square Root(x=w763) -> (sqrt(x)=w762:dbl)
                            n106 = Multiply(x=2, y=w753) -> (x*y=w751:dbl)
                            n107 = Less?(x=w762, y=w751) -> (x < y?=w760:bool)
                            n108 = Not Equal?(x=w754, y=w756) -> (x != y?=w759:bool)
                            n109 = Equal?(x=w758, y=w756) -> (x = y?=w761:bool)
                            n110 = And(x=w759, y=w760) -> (x .and. y?=w757:bool)
                            "Looper" <- w757
                            n111 = Or(x=w757, y=w761) -> (x .or. y?=w755:bool)
                          }
                        }
                        frame #1 {
                          n112 = local read "Looper"() -> (w774:bool)
                          n113 = case shown="False" w774 {
                            frame False {
                              n114 = local read "init"() -> (w775:dbl)
                              n115 = Add(x=w775, y=1) -> (x+y=w777:dbl)
                              n116 = local write "init"(w777) -> ()
                            }
                            frame True {
                            }
                          }
                        }
                      }
                      n117 = local read "Looper"() -> (w745:bool)
                    }
                  }
                  frame #2 {
                    n118 = local read "Looper"() -> (w782:bool)
                    n119 = case shown="True" w782 {
                      tunnel: w780 -> [w786 _]
                      tunnel: w779 -> [_ w794]
                      tunnel: ["This is an acceptable entry." "ERROR: A bubble will intersect the buffer zone."] -> w781
                      tunnel: [w786 w794] -> w778
                      frame False {
                        n120 = local write "Looper"(FALSE) -> ()
                        n121 = local read "Current Spot #"() -> (w787:dbl)
                        n122 = Index Array(array=w786, index=w787) -> (element=w785:T2)
                        n123 = Unbundle By Name(w785) -> ("Position.x"=w784:dbl, "Position.y"=w783:dbl)
                        n124 = local write "New Y"(w783) -> ()
                        n125 = local write "New X"(w784) -> ()
                      }
                      frame True {
                        # "Restore original position"
                        n126 = local write "Looper"(FALSE) -> ()
                        n127 = local read "Old Y"() -> (w791:dbl)
                        n128 = local read "Old X"() -> (w792:dbl)
                        n129 = local read "Position"() -> (w790:cluster{"x":dbl, "y":dbl, "z":dbl})
                        n130 = Bundle By Name(cluster=w790, "x"=w792, "y"=w791) -> (w793:cluster{"x":dbl, "y":dbl, "z":dbl})
                        n131 = local write "Position"(w793) -> ()
                      }
                    }
                  }
                }
                "Position Indicator" <- w709
              }
              event "Size": Value Change {
                # "If we were constraining the aspect ratio, or preventing a divide by zero, the size control on the FP may be incorrect.  We refresh it in here to stop it displaying a wrong value."
                # "If the size has changed, scale the spots"
                n132 = event-data() -> ("OldVal"=w803:cluster{"x":dbl, "y":dbl, "z":dbl}, "NewVal"=w809:cluster{"x":dbl, "y":dbl, "z":dbl})  [unwired: 5 out]
                n133 = Not Equal?(x=w803, y=w809) -> (x != y?=w802:cluster{"x":bool, "y":bool, "z":bool})
                n134 = Divide(x=w809, y=w803) -> (x/y=w808:cluster{"x":dbl, "y":dbl, "z":dbl})
                n135 = Not Equal To 0?(x=w803) -> (x != 0?=w801:cluster{"x":bool, "y":bool, "z":bool})
                n136 = And(x=w802, y=w801) -> (x .and. y?=w800:cluster{"x":bool, "y":bool, "z":bool})
                n137 = Cluster To Array(cluster=w800) -> (array=w807:bool[])
                n138 = Cluster To Array(cluster=w808) -> (array=w806:dbl[])
                n139 = case shown="True" "lock aspect ratio" {
                  tunnel: w807 -> [w815 w832]
                  tunnel: w806 -> [w814 w830]
                  tunnel: [w812 w822] -> w805
                  frame False {
                    # "We are not constraining the aspect ratio here, so just check we're not introducing NAs"
                    n140 = for {
                      tunnel: w815 -> [w821] mode=indexing
                      tunnel: w814 -> [w817] mode=indexing
                      tunnel: [w819] -> w813 mode=indexing
                      n141 = Not A Number/Path/Refnum?(number/path/refnum=w817) -> (NaN/Path/Refnum?=w818:bool)
                      n142 = Compound Arithmetic op=AND(w821, invert w818) -> (w820:bool)
                      n143 = Select(t=w817, s=w820, f=1.0) -> (s? t:f=w819:dbl)
                    }
                    n144 = Array To Cluster(array=w813) -> (cluster=w812:cluster{"[0]":dbl, "[1]":dbl, "[2]":dbl})
                  }
                  frame True {
                    # "Pick the first element that changed and use it.  Also need to make sure (1) an element did change and (2) everything's valid (no divide by zeros)"
                    n145 = Search 1D Array(1D array=w832, element=TRUE) -> (index of element=w829:i32)  [unwired: 1 in]
                    n146 = Index Array(array=w830, index=w829) -> (element=w825:dbl)
                    n147 = Not A Number/Path/Refnum?(number/path/refnum=w825) -> (NaN/Path/Refnum?=w828:bool)
                    n148 = Less Than 0?(x=w829) -> (x < 0?=w827:bool)
                    n149 = Or(x=w828, y=w827) -> (x .or. y?=w826:bool)
                    n150 = Select(t=1.0, s=w826, f=w825) -> (s? t:f=w823:dbl)
                    n151 = Bundle("x"=w823, "x"=w823, "x"=w823) -> (w822:cluster{"x":dbl, "x":dbl, "x":dbl})  [unwired: 1 in]
                  }
                }
                n152 = for {
                  tunnel: w811 -> [w838] mode=indexing
                  tunnel: w798 -> [w835] mode=indexing
                  tunnel: [w837] -> w799 mode=indexing
                  tunnel: w805 -> [w836]
                  tunnel: w810 -> [w833]
                  n153 = Unbundle(w835) -> ("Selected"=w834:bool)  [unwired: 1 out]
                  n154 = case shown="True" w834 {
                    tunnel: w838 -> [w839 w847]
                    tunnel: [w839 w846] -> w837
                    tunnel: w836 -> [_ w845]
                    tunnel: w833 -> [_ w841]
                    frame False {
                    }
                    frame True {
                      n155 = call "extract_position.vi"("Spot"=w847) -> ("Position"=w843:cluster{"x":dbl, "y":dbl, "z":dbl})
                      n156 = Subtract(x=w843, y=w841) -> (x-y=w844:cluster{"x":dbl, "y":dbl, "z":dbl})
                      n157 = Multiply(x=w844, y=w845) -> (x*y=w842:cluster{"x":dbl, dbl, dbl})
                      n158 = Add(x=w841, y=w842) -> (x+y=w840:cluster{"x":dbl, dbl, dbl})
                      n159 = call "replace_position.vi"("Position"=w840, "Spot in"=w847) -> ("Spot"=w846:T2)  [unwired: 2 out]
                    }
                  }
                }
                n160 = call "find_centroid.vi"("Selection and Groups"=w798, "Spots"=w799) -> ("size"=w797:cluster{"x":dbl, "y":dbl, "z":dbl})  [unwired: 2 in, 4 out]
                n161 = local write "Size"(w797) -> ()
              }
              event "Intensity": Value Change {
                # "When  the user changes intensity, scale all the spots selected so the new mean is correct but keep the ratio between the selected spots.\n\nThe exception to this is when the mean intensity is zero, in which case multiplying makes no sense- in that case we just replace with the new value."
                n162 = event-data() -> ("NewVal"=w848:dbl, "OldVal"=w855:dbl)  [unwired: 5 out]
                n163 = Equal To 0?(x=w855) -> (x = 0?=w851:bool)
                n164 = Not A Number/Path/Refnum?(number/path/refnum=w855) -> (NaN/Path/Refnum?=w850:bool)
                n165 = Or(x=w851, y=w850) -> (x .or. y?=w849:bool)
                n166 = Divide(x=w848, y=w855) -> (x/y=w852:dbl)
                n167 = for {
                  tunnel: w856 -> [w861] mode=indexing
                  tunnel: w853 -> [w863] mode=indexing
                  tunnel: [w860] -> w854 mode=indexing
                  tunnel: w852 -> [w859]
                  tunnel: w849 -> [w858]
                  tunnel: w848 -> [w857]
                  n168 = Unbundle(w863) -> ("Selected"=w862:bool)  [unwired: 1 out]
                  n169 = case shown="True" w862 {
                    tunnel: w861 -> [w864 w871]
                    tunnel: [w864 w868] -> w860
                    tunnel: w859 -> [_ w867]
                    tunnel: w858 -> [_ w866]
                    tunnel: w857 -> [_ w865]
                    frame False {
                    }
                    frame True {
                      n170 = Unbundle By Name(w871) -> ("Intensity"=w869:dbl)
                      n171 = case shown="True" w866 {
                        tunnel: [w874 w875] -> w870
                        tunnel: w869 -> [w873 _]
                        tunnel: w867 -> [w872 _]
                        tunnel: w865 -> [_ w875]
                        frame False {
                          n172 = Multiply(x=w873, y=w872) -> (x*y=w874:dbl)
                        }
                        frame True {
                        }
                      }
                      n173 = Bundle By Name(cluster=w871, "Intensity"=w870) -> (w868:T2)
                    }
                  }
                }
              }
              event "phase": Value Change {
                # "When  the user changes phase, translate the phase of all spots selectedd"
                n174 = event-data() -> ("NewVal"=w877:dbl, "OldVal"=w881:dbl)  [unwired: 5 out]
                n175 = Not A Number/Path/Refnum?(number/path/refnum=w881) -> (NaN/Path/Refnum?=w876:bool)
                n176 = Subtract(x=w877, y=w881) -> (x-y=w878:dbl)
                n177 = for {
                  tunnel: w882 -> [w887] mode=indexing
                  tunnel: w879 -> [w889] mode=indexing
                  tunnel: [w886] -> w880 mode=indexing
                  tunnel: w878 -> [w885]
                  tunnel: w876 -> [w884]
                  tunnel: w877 -> [w883]
                  n178 = Unbundle(w889) -> ("Selected"=w888:bool)  [unwired: 1 out]
                  n179 = case shown="False" w888 {
                    tunnel: w887 -> [w890 w897]
                    tunnel: [w890 w894] -> w886
                    tunnel: w885 -> [_ w893]
                    tunnel: w884 -> [_ w892]
                    tunnel: w883 -> [_ w891]
                    frame False {
                    }
                    frame True {
                      n180 = Unbundle By Name(w897) -> ("Phase"=w895:dbl)
                      n181 = case shown="False" w892 {
                        tunnel: [w900 w901] -> w896
                        tunnel: w895 -> [w899 _]
                        tunnel: w893 -> [w898 _]
                        tunnel: w891 -> [_ w901]
                        frame False {
                          n182 = Add(x=w899, y=w898) -> (x+y=w900:dbl)
                        }
                        frame True {
                        }
                      }
                      n183 = Bundle By Name(cluster=w897, "Phase"=w896) -> (w894:T2)
                    }
                  }
                }
              }
              event "Vortex Charge": Value Change {
                # "When  the user changes l, just set all selected spots to have that value of l."
                n184 = event-data() -> ("NewVal"=w902:i8)  [unwired: 6 out]
                n185 = for {
                  tunnel: w905 -> [w908] mode=indexing
                  tunnel: w903 -> [w910] mode=indexing
                  tunnel: [w907] -> w904 mode=indexing
                  tunnel: w902 -> [w906]
                  n186 = Unbundle(w910) -> ("Selected"=w909:bool)  [unwired: 1 out]
                  n187 = case shown="True" w909 {
                    tunnel: w908 -> [w911 w914]
                    tunnel: [w911 w913] -> w907
                    tunnel: w906 -> [_ w912]
                    frame False {
                    }
                    frame True {
                      n188 = Bundle By Name(cluster=w914, "Vortex Charge"=w912) -> (w913:T2)
                    }
                  }
                }
              }
            }
          }
          frame "Spot Shape" {
            # "We update the spot shape tab only when spots have changed OUTSIDE this tab.  This avoids unnecessary jumping about of the tab control."
            n189 = call "find_centroid.vi"("Selection and Groups"=w925, "Spots"=w926) -> ("Mean Values"=w921:T2)  [unwired: 2 in, 4 out]
            n190 = Wait (ms)(milliseconds to wait=u32 10) -> ()  [unwired: 1 out]
            n191 = call "spots_shape.vi"("Selection and Groups"=w925, "Spots"=w926) -> ("Spot Shape"=w928:enum32{"Normal", "Line", "NA", "Mixed"})  [unwired: 7 in]
            n192 = feedback-in #4(w921) -> ()
            n193 = feedback #4() -> (w922:T2)  [unwired: 1 in]
            n194 = Not Equal?(x=w922, y=w921) -> (x != y?=w927:bool)
            n195 = feedback #5() -> (w917:enum32{"Normal", "Line", "NA", "Mixed"})  [unwired: 1 in]
            n196 = feedback #6() -> (w919:T2)  [unwired: 1 in]
            n197 = Not Equal?(x=w919, y=w921) -> (x != y?=w918:bool)
            n198 = case shown="False" w918 {
              tunnel: w928 -> [_ w1047]
              tunnel: ["Spot Shape" w1047] -> w916
              frame False {
              }
              frame True {
                n199 = local write "Spot Shape"(w1047) -> ()
              }
            }
            n200 = feedback-in #5(w916) -> ()
            n201 = Not Equal?(x=w916, y=w917) -> (x != y?=w915:bool)
            n202 = case shown="\"Normal\", Default" w916 {
              tunnel: w926 -> [w932 w949 w975 w1045]
              tunnel: w925 -> [w931 w948 w974 w1044]
              tunnel: [w931 w947 w972 w1044] -> w923
              tunnel: [w930 w946 w973 w1045] -> w924
              tunnel: w921 -> [_ w945 w971 _]
              tunnel: w927 -> [_ w944 w970 _]
              tunnel: w915 -> [_ w942 w968 _]
              frame "Normal", Default {
                # "If \"normal\" is selected, don't allow any NA or line-trapping stuff"
                n203 = for {
                  tunnel: w932 -> [w935] mode=indexing
                  tunnel: w931 -> [w934] mode=indexing
                  tunnel: [w936] -> w930 mode=indexing
                  n204 = Unbundle(w934) -> ("Selected"=w933:bool)  [unwired: 1 out]
                  n205 = case shown="True" w933 {
                    tunnel: [w937 w941] -> w936
                    tunnel: w935 -> [w937 w940]
                    frame False {
                    }
                    frame True {
                      n206 = Bundle By Name(cluster=w940, "NA Position"=cluster{"x":dbl, "y":dbl, "r":dbl} {"x"=0.0, "y"=0.0, "r"=1.0} ("x"), "Line Trapping"=T3 {"Vector"={"x"=0.0, "y"=0.0, "z"=0.0}, "Phase Gradient"=0.0}) -> (w941:T2)
                    }
                  }
                }
              }
              frame "Line" {
                # "If it's out of date, update front panel"
                n207 = Or(x=w944, y=w942) -> (x .or. y?=w943:bool)
                n208 = case shown="True" w943 {
                  tunnel: w945 -> [_ w952]
                  frame False {
                  }
                  frame True {
                    n209 = Unbundle By Name(w952) -> ("Line Trapping"=w951:T3)
                    n210 = local write "Line Trapping"(w951) -> ()
                  }
                }
                n211 = event shown="[1] \"Line Trapping\": Value Change" {
                  selector: _ -> [_ _]
                  dyn-events: _ -> [_ _]
                  timeout: 10 -> [_ _]
                  tunnel: w949 -> [w954 w958]
                  tunnel: w948 -> [w953 w956]
                  tunnel: [w954 w957] -> w946
                  tunnel: [w953 w956] -> w947
                  event Timeout {
                    n212 = event-data() -> ()  [unwired: 3 out]
                  }
                  event Value Change {
                    # "If the line vector has changed, update it"
                    n213 = event-data() -> ("NewVal"=w955:T3)  [unwired: 6 out]
                    n214 = for {
                      tunnel: w958 -> [w963] mode=indexing
                      tunnel: w956 -> [w960] mode=indexing
                      tunnel: [w962] -> w957 mode=indexing
                      tunnel: w955 -> [w961]
                      n215 = Unbundle(w960) -> ("Selected"=w959:bool)  [unwired: 1 out]
                      n216 = case shown="True" w959 {
                        tunnel: w963 -> [w964 w966]
                        tunnel: [w964 w967] -> w962
                        tunnel: w961 -> [_ w965]
                        frame False {
                        }
                        frame True {
                          n217 = Bundle By Name(cluster=w966, "Line Trapping"=w965) -> (w967:T2)
                        }
                      }
                    }
                  }
                }
              }
              frame "NA" {
                n218 = Or(x=w968, y=w970) -> (x .or. y?=w969:bool)
                n219 = case shown="True" w969 {
                  tunnel: w971 -> [_ w980]
                  frame False {
                  }
                  frame True {
                    n220 = Unbundle By Name(w980) -> ("NA Position"=w979:cluster{"x":dbl, "y":dbl, "r":dbl})
                    n221 = call "xyz_to_xy.vi"("Position"=w979) -> ("Position (2D)"=w978:cluster{"x":dbl, "y":dbl}, "z"=w977:dbl)  [unwired: 6 out]
                    n222 = local write "Position on back aperture"(w978) -> ()
                    n223 = local write "Radius on back aperture"(w977) -> ()
                  }
                }
                n224 = event shown="[3] \"Scale BA\": Value Change" {
                  selector: _ -> [_ _ _ _]
                  dyn-events: _ -> [_ _ _ _]
                  timeout: 10 -> [_ _ _ _]
                  tunnel: w975 -> [w982 w988 w1009 w1031]
                  tunnel: w974 -> [w981 w986 w1006 w1032]
                  tunnel: [w982 w987 w1007 w1029] -> w973
                  tunnel: [w981 w986 w1006 w1032] -> w972
                  event Timeout {
                    n225 = event-data() -> ()  [unwired: 3 out]
                  }
                  event "Position on back aperture": Value Change {
                    # "If the position has changed, translate the spots"
                    n226 = event-data() -> ("OldVal"=w984:cluster{"x":dbl, "y":dbl}, "NewVal"=w985:cluster{"x":dbl, "y":dbl})  [unwired: 5 out]
                    n227 = Subtract(x=w985, y=w984) -> (x-y=w983:cluster{"x":dbl, "y":dbl})
                    n228 = for {
                      tunnel: w988 -> [w993] mode=indexing
                      tunnel: w986 -> [w990] mode=indexing
                      tunnel: [w992] -> w987 mode=indexing
                      tunnel: w983 -> [w991]
                      n229 = Unbundle(w990) -> ("Selected"=w989:bool)  [unwired: 1 out]
                      n230 = case shown="True" w989 {
                        tunnel: w993 -> [w994 w996]
                        tunnel: [w994 w997] -> w992
                        tunnel: w991 -> [_ w998]
                        frame False {
                        }
                        frame True {
                          n231 = Unbundle By Name(w996) -> ("NA Position"=w1000:cluster{"x":dbl, "y":dbl, "r":dbl})
                          n232 = call "xy_to_xyz.vi"("Position (2D)"=w998) -> ("Position (3D)"=w999:cluster{dbl, dbl, dbl})  [unwired: 1 in, 2 out]
                          n233 = Add(x=w1000, y=w999) -> (x+y=w995:cluster{dbl, dbl, dbl})
                          n234 = Bundle By Name(cluster=w996, "NA Position"=w995) -> (w997:T2)
                        }
                      }
                    }
                  }
                  event "Radius on back aperture": Value Change {
                    # "When  the user changes intensity, scale all the spots selected so the new mean is correct but keep the ratio between the selected spots.\n\nThe exception to this is when the mean intensity is zero, in which case multiplying makes no sense- in that case we just replace with the new value."
                    n235 = event-data() -> ("NewVal"=w1001:dbl, "OldVal"=w1008:dbl)  [unwired: 5 out]
                    n236 = Equal To 0?(x=w1008) -> (x = 0?=w1004:bool)
                    n237 = Not A Number/Path/Refnum?(number/path/refnum=w1008) -> (NaN/Path/Refnum?=w1003:bool)
                    n238 = Or(x=w1004, y=w1003) -> (x .or. y?=w1002:bool)
                    n239 = Divide(x=w1001, y=w1008) -> (x/y=w1005:dbl)
                    n240 = for {
                      tunnel: w1009 -> [w1014] mode=indexing
                      tunnel: w1006 -> [w1016] mode=indexing
                      tunnel: [w1013] -> w1007 mode=indexing
                      tunnel: w1005 -> [w1012]
                      tunnel: w1002 -> [w1011]
                      tunnel: w1001 -> [w1010]
                      n241 = Unbundle(w1016) -> ("Selected"=w1015:bool)  [unwired: 1 out]
                      n242 = case shown="True" w1015 {
                        tunnel: w1014 -> [w1017 w1024]
                        tunnel: [w1017 w1021] -> w1013
                        tunnel: w1012 -> [_ w1020]
                        tunnel: w1011 -> [_ w1019]
                        tunnel: w1010 -> [_ w1018]
                        frame False {
                        }
                        frame True {
                          n243 = Unbundle By Name(w1024) -> ("NA Position.r"=w1022:dbl)
                          n244 = case shown="False" w1019 {
                            tunnel: [w1027 w1028] -> w1023
                            tunnel: w1022 -> [w1026 _]
                            tunnel: w1020 -> [w1025 _]
                            tunnel: w1018 -> [_ w1028]
                            frame False {
                              n245 = Multiply(x=w1026, y=w1025) -> (x*y=w1027:dbl)
                            }
                            frame True {
                            }
                          }
                          n246 = Bundle By Name(cluster=w1024, "NA Position.r"=w1023) -> (w1021:T2)
                        }
                      }
                    }
                  }
                  event "Scale BA": Value Change {
                    n247 = event-data() -> ()  [unwired: 7 out]
                    n248 = for {
                      tunnel: w1032 -> [w1037] mode=indexing
                      tunnel: w1031 -> [w1035] mode=indexing
                      tunnel: "Scale back aperture" -> [w1034]
                      tunnel: [w1033] -> w1029 mode=indexing
                      n249 = Unbundle(w1037) -> ("Selected"=w1036:bool)  [unwired: 1 out]
                      n250 = case shown="True" w1036 {
                        tunnel: w1035 -> [w1038 w1039]
                        tunnel: w1034 -> [_ w1042]
                        tunnel: [w1038 w1040] -> w1033
                        frame False {
                        }
                        frame True {
                          n251 = Unbundle By Name(w1039) -> ("NA Position"=w1043:cluster{"x":dbl, "y":dbl, "r":dbl})
                          n252 = Multiply(x=w1042, y=w1043) -> (x*y=w1041:cluster{"x":dbl, "y":dbl, "r":dbl})
                          n253 = Bundle By Name(cluster=w1039, "NA Position"=w1041) -> (w1040:T2)
                        }
                      }
                    }
                  }
                }
              }
              frame "Mixed" {
              }
            }
            n254 = call "find_centroid.vi"("Selection and Groups"=w923, "Spots"=w924) -> ("Mean Values"=w920:T2)  [unwired: 2 in, 4 out]
            n255 = feedback-in #6(w920) -> ()
          }
          frame "Rotate" {
            w1058 = u32 0 items=["Frame", "Fill", "Highlight"] ("Drawing Mode")
            w1057 = u32 0 ("Color")
            w1054 = i16 100 ("radius")
            # "It's necessary to check this has changed to stop us unintentionally \"spinning\" the spots..."
            # "Draw the centroid as a spot, then a large circle+cross"
            # "It's important that this loop doesn't go too fast- it hogs the CPU.  However, each tab can have a different loop speed."
            n256 = Unbundle By Name(w1051) -> ("Position (Image Pixels)"=w1067:cluster{"X":dbl, "Y":dbl}, "Previous Position (Image Pixels)"=w1066:cluster{"X":dbl, "Y":dbl}, "Dragging"=w1068:bool)
            n257 = feedback-in #7(w1051) -> ()
            n258 = feedback #7() -> (w1052:T11)  [unwired: 1 in]
            n259 = call "find_centroid.vi"("Selection and Groups"=w1069, "Spots"=w1072) -> ("centroid"=w1065:cluster{"x":dbl, "y":dbl, "z":dbl})  [unwired: 2 in, 4 out]
            n260 = Not Equal?(x=w1051, y=w1052) -> (x != y?=w1049:bool)
            n261 = Wait (ms)(milliseconds to wait=u32 10) -> ()  [unwired: 1 out]
            n262 = And(x=w1049, y=w1068) -> (x .and. y?=w1050:bool)
            n263 = call "coords_real_to_image_currentview.vi"("Position (real coords)"=w1065) -> ("Position (pixels, relative to the top left of the image)"=w1048:cluster{dbl, dbl})  [unwired: 7 in, 1 out]
            n264 = case shown="True" w1050 {
              tunnel: w1072 -> [w1081 w1125]
              tunnel: [w1083 w1124] -> w1071
              tunnel: w1069 -> [w1082 w1126]
              tunnel: [w1082 w1126] -> w1070
              tunnel: w1065 -> [w1080 w1117]
              tunnel: w1067 -> [_ w1116]
              tunnel: w1066 -> [_ w1115]
              tunnel: w1048 -> [_ w1114]
              frame False {
                n265 = event shown="[1] Timeout" {
                  selector: _ -> [_ _]
                  dyn-events: _ -> [_ _]
                  timeout: 10 -> [_ _]
                  tunnel: [w1096 w1113] -> w1083
                  tunnel: w1082 -> [w1095 _]
                  tunnel: w1081 -> [w1094 w1113]
                  tunnel: w1080 -> [w1090 _]
                  event "rotate": Value Change {
                    n266 = event-data() -> ()  [unwired: 6 out]
                    n267 = case shown="3" "Rotation Axis" {
                      tunnel: [cluster{dbl, dbl, dbl} {0.0, 0.0, 1.0} ("Custom Axis") cluster{dbl, dbl, dbl} {1.0, 0.0, 0.0} ("Custom Axis") cluster{dbl, dbl, dbl} {0.0, 1.0, 0.0} ("Custom Axis") "Custom Axis"] -> w1091
                      frame 0, Default {
                        # "Z"
                      }
                      frame 1 {
                        # "X"
                      }
                      frame 2 {
                        # "Y"
                      }
                      frame 3 {
                      }
                    }
                    n268 = call "normalise_3d_vector.vi"("Vector"=w1091) -> ("Unit Vector"=w1093:cluster{dbl, dbl, dbl})  [unwired: 3 out]
                    n269 = Divide(x=6.283185307179586, y=360.0) -> (x/y=w1088:dbl)
                    n270 = Multiply(x="Angle (degrees)", y=w1088) -> (x*y=w1085:dbl)
                    n271 = call "arb_rotation_matrix.vi"("Unit Vector"=w1093, "theta"=w1085) -> ("Real Matrix"=w1097:T10)
                    n272 = for {
                      tunnel: w1095 -> [w1107] mode=indexing
                      tunnel: w1094 -> [w1102] mode=indexing
                      tunnel: [w1103] -> w1096 mode=indexing
                      tunnel: w1090 -> [w1105]
                      tunnel: w1097 -> [w1104]
                      n273 = Unbundle(w1107) -> ("Selected"=w1106:bool)  [unwired: 1 out]
                      n274 = case shown="True" w1106 {
                        tunnel: w1105 -> [_ w1112]
                        tunnel: [w1108 w1111] -> w1103
                        tunnel: w1102 -> [w1108 w1110]
                        tunnel: w1104 -> [_ w1109]
                        frame False {
                        }
                        frame True {
                          n275 = call "apply_matrix_transformation_to_spots.vi"("Transform centre (i.e. transform about this point)"=w1112, "Transformation Matrix (3x3)"=w1109, "Spot In"=w1110) -> ("Spot Out"=w1111:T2)  [unwired: 5 out]
                        }
                      }
                    }
                  }
                  event Timeout {
                    n276 = event-data() -> ()  [unwired: 4 out]
                  }
                }
              }
              frame True {
                # "if the mouse has not moved, stuff will be NaN, so let's make like a leopard and not change our spots"
                # "the magnitude of the change in our direction vector gives the rotation angle in radians"
                # "If it's within 100px of the centroid, pretend the mouse is on the surface of a sphere, and synthesize Z accordingly (z^2=100^2-x^2-y^2).  This allows rotation in 3d :)  The output should always be a unit vector."
                n277 = Build Array(w1116, w1115) -> (w1131:cluster{"X":dbl, "Y":dbl}[])
                n278 = for {
                  tunnel: w1114 -> [w1164]
                  tunnel: w1131 -> [w1160] mode=indexing
                  tunnel: [w1150] -> w1130 mode=indexing
                  n279 = Subtract(x=w1160, y=w1164) -> (x-y=w1155:cluster{dbl, dbl})
                  n280 = Divide(x=w1155, y=100.0 ("x")) -> (x/y=w1156:cluster{dbl, dbl})
                  n281 = Square(x=w1156) -> (x^2=w1163:cluster{dbl, dbl})
                  n282 = Unbundle(w1163) -> (w1161:dbl, w1162:dbl)
                  n283 = Add(x=w1161, y=w1162) -> (x+y=w1152:dbl)
                  n284 = Subtract(x=1.0, y=w1152) -> (x-y=w1158:dbl)
                  n285 = Square Root(x=w1152) -> (sqrt(x)=w1153:dbl)
                  n286 = Greater Than 0?(x=w1158) -> (x > 0?=w1159:bool)
                  n287 = case shown="False" w1159 {
                    tunnel: w1158 -> [_ w1171]
                    tunnel: [0.0 w1170] -> w1149
                    tunnel: w1156 -> [w1168 w1169]
                    tunnel: w1153 -> [w1167 _]
                    tunnel: [w1166 w1169] -> w1151
                    frame False {
                      n288 = Divide(x=w1168, y=w1167) -> (x/y=w1166:cluster{dbl, dbl})
                    }
                    frame True {
                      n289 = Square Root(x=w1171) -> (sqrt(x)=w1170:dbl)
                    }
                  }
                  n290 = call "xy_to_xyz.vi"("z"=w1149, "Position (2D)"=w1151) -> ("Position (3D)"=w1150:cluster{dbl, dbl, dbl})  [unwired: 2 out]
                }
                n291 = Index Array(array=w1130) -> (element #1=w1129:cluster{dbl, dbl, dbl}, element #2=w1120:cluster{dbl, dbl, dbl})  [unwired: 2 in]
                n292 = Add(x=w1129, y=w1120) -> (x+y=w1119:cluster{dbl, dbl, dbl})
                n293 = Subtract(x=w1129, y=w1120) -> (x-y=w1118:cluster{dbl, dbl, dbl})
                n294 = call "cross_product.vi"("b"=w1119, "a"=w1118) -> ("a cross b"=w1128:cluster{dbl, dbl, dbl})
                n295 = call "normalise_3d_vector.vi"("Vector"=w1128) -> ("Unit Vector"=w1127:cluster{dbl, dbl, dbl})  [unwired: 3 out]
                n296 = call "normalise_3d_vector.vi"("Vector"=w1118) -> ("magnitude"=w1122:dbl)  [unwired: 3 out]
                n297 = Not Equal To 0?(x=w1122) -> (x != 0?=w1121:bool)
                n298 = call "arb_rotation_matrix.vi"("Unit Vector"=w1127, "theta"=w1122) -> ("Real Matrix"=w1123:T10)
                n299 = case shown="True" w1121 {
                  tunnel: w1126 -> [_ w1137]
                  tunnel: w1125 -> [w1132 w1136]
                  tunnel: [w1132 w1135] -> w1124
                  tunnel: w1123 -> [_ w1134]
                  tunnel: w1117 -> [_ w1133]
                  frame False {
                  }
                  frame True {
                    n300 = for {
                      tunnel: w1137 -> [w1143] mode=indexing
                      tunnel: w1136 -> [w1140] mode=indexing
                      tunnel: [w1139] -> w1135 mode=indexing
                      tunnel: w1134 -> [w1141]
                      tunnel: w1133 -> [w1138]
                      n301 = Unbundle(w1143) -> ("Selected"=w1142:bool)  [unwired: 1 out]
                      n302 = case shown="True" w1142 {
                        tunnel: [w1144 w1147] -> w1139
                        tunnel: w1140 -> [w1144 w1148]
                        tunnel: w1141 -> [_ w1145]
                        tunnel: w1138 -> [_ w1146]
                        frame False {
                        }
                        frame True {
                          n303 = call "apply_matrix_transformation_to_spots.vi"("Transform centre (i.e. transform about this point)"=w1146, "Transformation Matrix (3x3)"=w1145, "Spot In"=w1148) -> ("Spot Out"=w1147:T2)  [unwired: 5 out]
                        }
                      }
                    }
                  }
                }
              }
            }
            n304 = call "coords_real_to_image_currentview.vi"("Position (real coords)"=w1065) -> ("Position (pixels, relative to the top left of the image)"=w1060:cluster{dbl, dbl}, "z (real coords)"=w1064:dbl)  [unwired: 7 in]
            n305 = expression code="z*1e7+20"(w1064) -> (w1076:dbl)
            n306 = In Range and Coerce(upper limit=100.0, x=w1076, lower limit=2.0) -> (coerced(x)=w1063:dbl)  [unwired: 1 out]
            n307 = Bundle("upper limit"=w1063, "upper limit"=w1063) -> (w1056:cluster{"upper limit":dbl, "upper limit":dbl})  [unwired: 1 in]
            n308 = call "myoverlay_oval.vi"("Color"=w1057, "Drawing Mode"=w1058, "Size"=w1056, "Centre Position (pixels on image)"=w1060) -> ("Overlay Elements Out"=w1062:T19[])  [unwired: 5 in]
            n309 = Bundle("radius"=w1054, "radius"=w1054) -> (w1055:cluster{"radius":i16, "radius":i16})  [unwired: 1 in]
            n310 = call "myoverlay_oval.vi"("Color"=w1057, "Drawing Mode"=w1058, "Size"=w1055, "Centre Position (pixels on image)"=w1060, "Overlay Elements In"=w1062) -> ("Overlay Elements Out"=w1061:T19[])  [unwired: 4 in]
            n311 = Multiply(x=w1054, y=cluster{dbl, dbl}[] [{0.0, 0.0}, {1.0, 0.0}, {0.0, 0.0}, {0.0, 1.0}, {0.0, 0.0}, {-1.0, 0.0}, {0.0, 0.0}, {0.0, -1.0}, {0.0, 0.0}]) -> (x*y=w1073:cluster{dbl, dbl}[])
            n312 = Add(x=w1060, y=w1073) -> (x+y=w1059:cluster{dbl, dbl}[])
            n313 = call "myoverlay_lines.vi"("Color"=w1057, "Drawing Mode"=w1058, "Line Endpoints"=w1059, "Overlay Elements In"=w1061) -> ("Overlay Elements Out"=w1053:T19[])  [unwired: 5 in]
          }
          frame "Patterns" {
            n314 = event shown="[3] \"Optimise\": Value Change" {
              selector: _ -> [_ _ _ _ _]
              dyn-events: _ -> [_ _ _ _ _]
              timeout: u32 10 ("milliseconds to wait") -> [_ _ _ _ _]
              tunnel: [w1190 w1220 w1224 w1227 w1238] -> w1173
              tunnel: [w1189 w1221 w1223 w1230 w1239] -> w1172
              tunnel: w1175 -> [w1188 w1220 w1224 w1228 w1237]
              tunnel: w1174 -> [w1187 w1221 w1223 w1230 w1239]
              event "Generate": Value Change {
                # "If there were previous spots, centre the pattern on the spots"
                n315 = event-data() -> ()  [unwired: 1 in, 1 out]
                n316 = call "find_centroid.vi"("Selection and Groups"=w1187, "Spots"=w1188) -> ("size"=w1183:cluster{"x":dbl, "y":dbl, "z":dbl}, "centroid"=w1179:cluster{"x":dbl, "y":dbl, "z":dbl}, "# selected"=w1185:i16)  [unwired: 2 in, 2 out]
                n317 = Greater?(x=w1185, y=i16 1) -> (0:w1180:bool)
                n318 = case shown="False" w1180 {
                  tunnel: w1183 -> [_ w1206]
                  tunnel: [cluster{"x":dbl, "y":dbl, "z":dbl} {"x"=2e-05, "y"=2e-05, "z"=2e-05} ("size") w1206] -> w1182
                  frame False {
                  }
                  frame True {
                  }
                }
                n319 = case shown="\"HCP Shack-Hartmann\"" "Pattern" {
                  tunnel: [w1208 w1211 w1217] -> w1181
                  tunnel: w1182 -> [_ w1210 _]
                  frame "Square Shack-Hartmann" {
                    n320 = call "patterns_square_shack_hartmann.vi"("N"="Spots across centre") -> ("Spots"=w1208:T2[])
                  }
                  frame "HCP Shack-Hartmann" {
                    n321 = Unbundle By Name(w1210) -> ("x"=w1209:dbl)
                    n322 = call "pattern_hcp_shack_hartmann.vi"("Width"=w1209, "Reference Array?"="Reference Array?", "Fraction of SLM"="Fraction of SLM", "N"="Spots across centre") -> ("Shack-Hartmann Spots"=w1211:T2[])  [unwired: 7 in]
                  }
                  frame "Rectangular Grid" {
                    n323 = call "patterns_rectangular_grid.vi"("spacing/m"="spacing/m", "N"="N") -> ("Spots"=w1217:T2[])
                  }
                }
                n324 = local write "Generate"(FALSE ("Generate")) -> ()
                n325 = case shown="True" w1180 {
                  tunnel: w1181 -> [w1193 w1197]
                  tunnel: w1179 -> [_ w1199]
                  tunnel: [w1193 w1195] -> w1191
                  frame False {
                  }
                  frame True {
                    n326 = call "find_centroid.vi"("Spots"=w1197) -> ("centroid"=w1198:cluster{"x":dbl, "y":dbl, "z":dbl}, "# selected"=→"# selected":i16)  [unwired: 3 in, 3 out]
                    n327 = Subtract(x=w1199, y=w1198) -> (x-y=w1196:cluster{"x":dbl, "y":dbl, "z":dbl})
                    n328 = for {
                      tunnel: w1197 -> [w1202] mode=indexing
                      tunnel: w1196 -> [w1201]
                      tunnel: [w1200] -> w1195 mode=indexing
                      n329 = call "extract_position.vi"("Spot"=w1202) -> ("Position"=w1203:cluster{"x":dbl, "y":dbl, "z":dbl})
                      n330 = Add(x=w1203, y=w1201) -> (x+y=w1204:cluster{"x":dbl, "y":dbl, "z":dbl})
                      n331 = call "replace_position.vi"("Position"=w1204, "Spot in"=w1202) -> ("Spot"=w1200:T2)  [unwired: 2 out]
                    }
                  }
                }
                "Last Pattern" <- w1191
                n332 = call "ensure_selection_matches_spots.vi"("Select All (default: no)"=TRUE ("Select All (default: true)"), "Spots"=w1191) -> ("Selection and Groups out"=w1189:T8[], "Spots (duplicate)"=w1190:T2[])  [unwired: 4 in]
              }
              event "Spots across centre", "Fraction of SLM", "Reference Array?", "N", "spacing/m", "Spots across centre": Value Change {
                n333 = event-data() -> ()  [unwired: 1 in, 1 out]
                n334 = local read "Last Pattern"() -> (w1219:T2[])
                n335 = Equal?(x=w1220, y=w1219) -> (x = y?=w1218:bool)
                n336 = case shown="True" w1218 {
                  selector: w1218 -> [_ w1222]
                  frame False {
                  }
                  frame True {
                    n337 = property on="Generate" class="Bool (strict)"("Val(Sgnl)"=w1222) -> ()  [unwired: 2 in, 2 out]
                  }
                }
              }
              event Timeout {
                n338 = event-data() -> ()  [unwired: 1 in, 1 out]
              }
              event "Optimise": Value Change {
                n339 = event-data() -> ()  [unwired: 1 in, 1 out]
                n340 = for {
                  N: "Iterations" -> [_]
                  tunnel: 203 ("Optimisation Resolution") -> [w1234]
                  shift-right: [w1235] -> w1227
                  shift-left: w1228 -> [w1236]
                  tunnel: "Fall-off/m" -> [w1231]
                  n341 = call "do_gsw_step.vi"("Optimisation Resolution"=w1234, "Sinc Zero"=w1231, "Spots In"=w1236) -> ("non-uniformity"=→"non-uniformity":dbl, "efficiency"=→"efficiency":dbl, "Spots Out"=w1235:T2[])  [unwired: 6 in]
                }
              }
              event "Reset Phase/Amplitude": Value Change {
                n342 = event-data() -> ()  [unwired: 1 in, 1 out]
                n343 = for {
                  tunnel: [w1242] -> w1238 mode=indexing
                  tunnel: w1237 -> [w1243] mode=indexing
                  n344 = Bundle By Name(cluster=w1243, "Phase"=0.0, "Amplitude Correction"=0.0) -> (w1242:T2)
                }
              }
            }
          }
          frame "Plugins" {
            # "The local variable ensures the references are  correct when they make it through to the \"close plugins\" block."
            # "This is the error from loading/unloading VIs on the front panel"
            n345 = control-ref of="Plugin Pnl"() -> (w1247:refnum<vi>)
            n346 = Wait (ms)(milliseconds to wait=u32 10) -> ()  [unwired: 1 out]
            n347 = feedback #8() -> (w1246:T4)
            n348 = feedback #9() -> (w1248:errorcluster)
            n349 = event shown="[1] \"Plugin:\": Value Change" {
              selector: _ -> [_ _ _]
              dyn-events: _ -> [_ _ _]
              timeout: 10 -> [_ _ _]
              tunnel: "Abort Plugin" -> [w1255 _ _]
              tunnel: "Plugin:" -> [w1260 _ w1276]
              tunnel: w1248 -> [w1259 w1274 w1278]
              tunnel: [w1258 w1269 w1277] -> w1249
              tunnel: [w1257 w1270 w1280] -> w1245
              tunnel: w1246 -> [w1261 w1271 w1279]
              tunnel: w1247 -> [_ w1272 _]
              event Timeout {
                n350 = event-data() -> ()  [unwired: 1 in, 2 out]
                n351 = Not(x=w1255) -> (.not. x?=w1256:bool)
                n352 = case shown="True" w1256 {
                  tunnel: w1261 -> [w1263 w1268]
                  tunnel: w1260 -> [_ w1267]
                  tunnel: w1259 -> [w1262 w1266]
                  tunnel: [w1262 w1265] -> w1258
                  tunnel: [w1263 w1264] -> w1257
                  frame False {
                  }
                  frame True {
                    n353 = call "plugins_run.vi"("Error In"=w1266, "Plugin Index"=w1267, "Plugins In"=w1268) -> ("Error Out"=w1265:errorcluster, "Plugins"=w1264:T4)  [unwired: 7 in]
                  }
                }
              }
              event "Plugin:": Value Change {
                n354 = event-data() -> ("NewVal"=w1273:u16)  [unwired: 1 in]
                n355 = call "plugins_switch.vi"("error in"=w1274, "Plugin Pnl"=w1272, "Plugin Index"=w1273, "Plugins In"=w1271) -> ("error out"=w1269:errorcluster, "Plugins Out"=w1270:T4)  [unwired: 4 in]
              }
              event "Abort Plugin": Value Change {
                n356 = event-data() -> ("NewVal"=w1275:bool)  [unwired: 1 in]
                n357 = case shown="True" w1275 {
                  tunnel: [w1282 w1287] -> w1280
                  tunnel: w1279 -> [w1282 w1286]
                  tunnel: w1278 -> [w1281 w1285]
                  tunnel: [w1281 w1284] -> w1277
                  tunnel: w1276 -> [_ w1283]
                  frame False {
                  }
                  frame True {
                    n358 = call "plugins_abort.vi"("Error In"=w1285, "Plugin Index"=w1283, "Plugins In"=w1286) -> ("Error Out"=w1284:errorcluster, "Plugins Out"=w1287:T4)  [unwired: 7 in]
                  }
                }
              }
            }
            n359 = feedback-in #8(w1245) -> ()
            n360 = feedback-in #9(w1249) -> ()
            n361 = local write "Plugins"(w1245) -> ()
          }
          frame "Video" {
            # "All the controls on this tab are in the bottom (camera) loop."
            n362 = Wait (ms)(milliseconds to wait=u32 10) -> ()  [unwired: 1 out]
            n363 = property on="Property Node" class="ImageControl"(reference=w1288) -> ("Image Information String"=→"Image Information":string)  [unwired: 1 in, 2 out]
          }
        }
      }
      event "Tab": Value Change {
        w1296 = T20 [enum."Video", enum."Particle Tracking"] items=["Current Spot", "Rotate", "Spot Shape", "Patterns", "Plugins", "Video", "Particle Tracking", "Clamping", "Blank"]
        w1301 = refnum<vi> refnum  # Image
        # "This allows us to disable custom mouse-handling for certain tabs.  It can also be done from within the \"mouse down\" event case."
        n364 = event-data() -> ("NewVal"=w1297:T5)  [unwired: 1 in, 3 out]
        n365 = Equal?(x=w1296, y=w1297) -> (x = y?=w1295:bool[])
        n366 = Or Array Elements(Boolean array=w1295) -> (logical OR=w1294:bool)
        n367 = Not(x=w1294) -> (.not. x?=w1293:bool)
        n368 = Select(t=w1300, s=w1293, f=w1301) -> (s? t:f=w1302:refnum<vi>)
        n369 = register-events(reference=w1304, w1302, w1301, w1301, w1301) -> (reference out=w1303:refnum<event-registration>)  [unwired: 1 in, 1 out]
      }
      event Menu Selection (User) {
        n370 = event-data() -> ("ItemTag"=w1312:string, "MenuRef"=w1305:refnum<k9>)  [unwired: 1 in]
        n371 = case shown="\"ToggleSavingData\"" w1312 {
          tunnel: w1316 -> [w1320 w1330 w1339 w1353 w1372 w1376 w1379 w1386 w1393 w1395 w1398 w1427 w1453 w1474 w1485 w1496 w1499 w1501 w1506 w1509]
          tunnel: w1315 -> [w1319 w1329 w1338 w1362 w1371 w1375 w1377 w1384 w1392 w1394 w1397 w1426 w1452 w1473 w1484 w1495 w1498 w1502 w1507 w1508]
          tunnel: [w1320 w1330 w1339 w1353 w1370 w1373 w1379 w1386 w1393 w1395 w1398 w1427 w1453 w1474 w1485 w1496 w1499 w1501 w1506 w1509] -> w1314
          tunnel: [w1319 w1329 w1338 w1362 w1369 w1374 w1378 w1385 w1391 w1396 w1399 w1426 w1452 w1473 w1484 w1495 w1498 w1502 w1507 w1508] -> w1313
          tunnel: [_ _ _ _ TRUE _ _ _ _ _ _ _ _ _ _ _ _ _ _ _] -> w1307
          tunnel: w1306 -> [_ _ _ _ _ _ _ _ _ _ _ w1425 w1451 w1465 _ _ _ _ _ _]
          tunnel: w1305 -> [_ _ _ _ _ _ _ _ _ _ _ w1416 w1445 w1468 w1479 w1490 _ _ _ _]
          frame "ToggleSavingData" {
            # "Data is saved from the middle loop: look there for an explanation."
            n372 = local read "Save Video"() -> (w1318:bool)
            n373 = Not(x=w1318) -> (.not. x?=w1317:bool)
            n374 = local write "Save Video"(w1317) -> ()
          }
          frame "SaveStateToFile" {
            # "Save the current settings (i.e. the values of all the controls in VIs that have [Red Tweezers Save Settings] in their documentation string) to a file."
            n375 = call "File Dialog"("prompt"="Please select a location to save the settings", "button label"="Save", "default name"="red_tweezers_settings.xml", "pattern (all files)"="*.xml" ("pattern label"), "pattern label"="XML Settings Files") -> ("selected path"=w1328:path, "cancelled"=w1321:bool)  [unwired: 7 in, 2 out]
            n376 = Not(x=w1321) -> (.not. x?=w1322:bool)
            n377 = case shown="True" w1322 {
              tunnel: w1328 -> [_ w1332]
              frame False {
              }
              frame True {
                n378 = Path To String(path=w1332) -> (string=w1331:string)
                n379 = call "settings_save_to_file.vi"("XML File Path"=w1332) -> ()  [unwired: 11 in]
                n380 = call "settings_filename_to_registry.vi"("Last Used Settings File"=w1331) -> ()  [unwired: 11 in]
              }
            }
          }
          frame "SaveStateToCurrentFile" {
            # "As SaveStateToFile, but using the current file (i.e. Save not Save As...)."
            n381 = global read "red_tweezers_globals_INTERNAL_VOLATILE.vi" "Current Settings File"() -> (w1337:path)
            n382 = call <vilib>:"Check if File or Folder Exists.vi"("path"=w1337) -> ("file or folder exists?"=w1336:bool, "dup path"=w1335:path)  [unwired: 8 in, 1 out]
            n383 = case shown="True" w1336 {
              selector: w1336 -> [_ w1350]
              tunnel: w1335 -> [_ w1351]
              tunnel: [w1342 w1351] -> w1334
              tunnel: [w1343 w1350] -> w1333
              frame False {
                n384 = call "File Dialog3"("prompt"="Please select a location to save the settings", "button label"="Save", "default name"="red_tweezers_settings.xml", "pattern (all files)"="*.xml" ("pattern label"), "pattern label"="XML Settings Files") -> ("selected path"=w1342:path, "cancelled"=w1349:bool)  [unwired: 7 in, 2 out]
                n385 = Not(x=w1349) -> (.not. x?=w1343:bool)
              }
              frame True {
              }
            }
            n386 = case shown="True" w1333 {
              tunnel: w1334 -> [_ w1341]
              frame False {
              }
              frame True {
                n387 = Path To String(path=w1341) -> (string=w1340:string)
                n388 = call "settings_save_to_file.vi"("XML File Path"=w1341) -> ()  [unwired: 11 in]
                n389 = call "settings_filename_to_registry.vi"("Last Used Settings File"=w1340) -> ()  [unwired: 11 in]
              }
            }
          }
          frame "LoadStateFromFile" {
            # "Load a file, and use it to reset the values of all the front panel controls."
            # "We need to re-run the initialisation stuff in UDP sender after changing settings\n(for example, this synchronises the settings like camera pixel size with the\nrelevant global variable)"
            n390 = call "File Dialog2"("prompt"="Please select a settings file", "button label"="Open", "default name"="red_tweezers_settings.xml", "pattern (all files)"="*.xml" ("pattern label"), "pattern label"="XML Settings Files") -> ("selected path"=w1354:path, "cancelled"=w1361:bool)  [unwired: 7 in, 2 out]
            n391 = Not(x=w1361) -> (.not. x?=w1360:bool)
            n392 = case shown="False" w1360 {
              selector: w1360 -> [w1363 w1364]
              tunnel: w1354 -> [_ w1365]
              tunnel: [w1363 w1364] -> w1352
              frame False {
              }
              frame True {
                n393 = call "settings_load_from_file.vi"("XML File Path"=w1365) -> ()  [unwired: 9 in, 2 out]
                n394 = Path To String(path=w1365) -> (string=w1366:string)
                n395 = call "settings_filename_to_registry.vi"("Last Used Settings File"=w1366) -> ()  [unwired: 11 in]
              }
            }
            n396 = call "UDP Sender generic_2.vi"("re-initialise"=w1352, "Spots"=w1353) -> ()  [unwired: 1 in, 1 out]
          }
          frame "Undo" {
            # "This should get the last undo vector and replace the spots with it :)"
            n397 = call "red_tweezers_UNDO.vi"("Selection/Group"=w1371, "Undo/Store (store, False)"=TRUE, "Spots"=w1372) -> ("Selection/Group Out (Undo only)"=w1369:T8[], "Spots Out (Undo only)"=w1370:T2[])  [unwired: 7 in]
          }
          frame "Delete" {
            n398 = call "delete_selected_spots.vi"("Selection/Group 3"=w1375, "Spots 3"=w1376) -> ("Selection/Group 2"=w1374:T8[], "Spots 2"=w1373:T2[])  [unwired: 4 in]
          }
          frame "SelectAllSpots" {
            n399 = for {
              tunnel: w1377 -> [w1382] mode=indexing
              tunnel: [w1383] -> w1378 mode=indexing
              n400 = Unbundle(w1382) -> ("Group ID"=w1381:i32)  [unwired: 1 out]
              n401 = Bundle(cluster=w1382, "Group ID"=w1381, "Selected"=TRUE ("Label.Visible")) -> (w1383:T8)
            }
          }
          frame "SelectNoSpots" {
            n402 = for {
              tunnel: w1384 -> [w1389] mode=indexing
              tunnel: [w1390] -> w1385 mode=indexing
              n403 = Unbundle(w1389) -> ("Group ID"=w1388:i32)  [unwired: 1 out]
              n404 = Bundle(cluster=w1389, "Group ID"=w1388, "Selected"=FALSE ("Label.Visible")) -> (w1390:T8)
            }
          }
          frame "SelectSpecificSpots" {
            n405 = call "select_by_id.vi"("Selection/Group"=w1392, "Spots"=w1393) -> ("Selection/Group Out"=w1391:T8[])  [unwired: 9 in]
          }
          frame "Group" {
            # "Group the currently selected spots"
            n406 = call "group_selected_spots.vi"("Selection/Group 2"=w1394) -> ("Array"=w1396:T8[])
          }
          frame "Ungroup" {
            # "Ungroup the currently selected spots"
            n407 = for {
              tunnel: [w1403] -> w1399 mode=indexing
              tunnel: w1397 -> [w1402] mode=indexing
              tunnel: 0 -> [w1401]
              n408 = Unbundle(w1402) -> ("Selected"=w1404:bool)  [unwired: 1 out]
              n409 = case shown="False" w1404 {
                tunnel: [w1405 w1408] -> w1403
                tunnel: w1402 -> [w1405 w1407]
                tunnel: w1401 -> [_ w1406]
                frame False {
                }
                frame True {
                  n410 = Unbundle(w1407) -> ("Selected"=w1409:bool)  [unwired: 1 out]
                  n411 = Bundle(cluster=w1407, "Group ID"=w1406, "Selected"=w1409) -> (w1408:T8)
                }
              }
            }
          }
          frame "ZoomIn" {
            w1410 = "ZoomToFit" ("item tag")
            # "turn off \"zoom to fit\""
            n412 = property class="ImageControl"(reference=w1425) -> (reference out=w1419:refnum<vi>, "ZoomSingle"=w1424:cluster{"X":sgl, "Y":sgl}, "Image Center Position"=w1417:cluster{"X":u32, "Y":u32})  [unwired: 1 in, 1 out]
            n413 = Unbundle(w1424) -> ("X"=w1422:sgl)  [unwired: 1 out]
            n414 = Round To Nearest(number=w1422) -> (nearest integer value=w1418:sgl)
            n415 = Greater Than 0?(x=w1418) -> (x > 0?=w1423:bool)
            n416 = case shown="True" w1423 {
              tunnel: w1422 -> [w1432 w1435]
              tunnel: [w1431 w1433] -> w1421
              frame False {
                n417 = Reciprocal(x=w1432) -> (1/x=w1429:sgl)
                n418 = Round Toward +Infinity(x=w1429) -> (ceil(x): smallest int >= x=w1430:sgl)
                n419 = Decrement(x=w1430) -> (x-1=w1428:sgl)
                n420 = Reciprocal(x=w1428) -> (1/x=w1431:sgl)
              }
              frame True {
                n421 = Round Toward -Infinity(1:w1435) -> (0:w1434:sgl)
                n422 = Increment(x=w1434) -> (x+1=w1433:sgl)
              }
            }
            n423 = Bundle(w1421, w1421) -> (w1420:cluster{sgl, sgl})  [unwired: 1 in]
            n424 = property class="ImageControl"(reference=w1419, "ZoomSingle"=w1420, "Image Center Position"=w1417) -> ()  [unwired: 1 in, 2 out]
            n425 = Get Menu Item Info(7:w1410, 11:w1416) -> (1:w1413:bool, 2:w1414:string, 3:w1415:refnum<k9>, 6:w1412:T21)  [unwired: 1 in, 3 out]
            n426 = Set Menu Item Info(4:w1412, 6:FALSE ("checked"), 7:w1410, 9:w1413, 10:w1414, 11:w1415) -> ()  [unwired: 1 in, 2 out]
          }
          frame "ZoomOut" {
            w1439 = "ZoomToFit" ("item tag")
            # "turn off \"zoom to fit\""
            n427 = property class="ImageControl"(reference=w1451) -> (reference out=w1447:refnum<vi>, "ZoomSingle"=w1450:cluster{"X":sgl, "Y":sgl}, "Image Center Position"=w1446:cluster{"X":u32, "Y":u32})  [unwired: 1 in, 1 out]
            n428 = Unbundle(w1450) -> ("X"=w1436:sgl)  [unwired: 1 out]
            n429 = Greater?(x=w1436, y=1.0) -> (0:w1438:bool)
            n430 = case shown="False" w1438 {
              tunnel: w1436 -> [w1460 w1463]
              tunnel: [w1459 w1461] -> w1449
              frame False {
                n431 = Reciprocal(x=w1460) -> (1/x=w1457:sgl)
                n432 = Add(x=w1457, y=sgl 0.01 ("x")) -> (x+y=w1455:sgl)
                n433 = Round Toward -Infinity(1:w1455) -> (0:w1458:sgl)
                n434 = Increment(x=w1458) -> (x+1=w1456:sgl)
                n435 = Reciprocal(x=w1456) -> (1/x=w1459:sgl)
              }
              frame True {
                n436 = Round Toward +Infinity(x=w1463) -> (ceil(x): smallest int >= x=w1462:sgl)
                n437 = Decrement(x=w1462) -> (x-1=w1461:sgl)
              }
            }
            n438 = Bundle(w1449, w1449) -> (w1448:cluster{sgl, sgl})  [unwired: 1 in]
            n439 = property class="ImageControl"(reference=w1447, "ZoomSingle"=w1448, "Image Center Position"=w1446) -> ()  [unwired: 1 in, 2 out]
            n440 = Get Menu Item Info(7:w1439, 11:w1445) -> (1:w1442:bool, 2:w1443:string, 3:w1444:refnum<k9>, 6:w1441:T21)  [unwired: 1 in, 3 out]
            n441 = Set Menu Item Info(4:w1441, 6:FALSE ("checked"), 7:w1439, 9:w1442, 10:w1443, 11:w1444) -> ()  [unwired: 1 in, 2 out]
          }
          frame "ZoomToFit" {
            w1469 = "ZoomToFit" ("item tag")
            # "and make sure the image obeys the result"
            # "Toggle menu checkmark"
            n442 = Get Menu Item Info(7:w1469, 11:w1468) -> (1:w1467:bool, 2:w1471:string, 3:w1472:refnum<k9>, 4:w1466:bool, 6:w1470:T21)  [unwired: 1 in, 2 out]
            n443 = Not(x=w1466) -> (.not. x?=w1464:bool)
            n444 = Set Menu Item Info(4:w1470, 6:w1464, 7:w1469, 9:w1467, 10:w1471, 11:w1472) -> ()  [unwired: 1 in, 2 out]
            n445 = property class="ImageControl"(reference=w1465, "Zoom to Fit Mode"=w1464) -> ()  [unwired: 1 in, 2 out]
          }
          frame "ShowGrid" {
            w1480 = "ShowGrid" ("item tag")
            # "Toggle menu checkmark"
            n446 = Get Menu Item Info(7:w1480, 11:w1479) -> (1:w1478:bool, 2:w1482:string, 3:w1483:refnum<k9>, 4:w1477:bool, 6:w1481:T21)  [unwired: 1 in, 2 out]
            n447 = Not(x=w1477) -> (.not. x?=w1476:bool)
            n448 = Set Menu Item Info(4:w1481, 6:w1476, 7:w1480, 9:w1478, 10:w1482, 11:w1483) -> ()  [unwired: 1 in, 2 out]
            n449 = call "grid_and_guides.vi"("Boolean"=w1476, "Operation"=T14."Set grid visibility") -> ()  [unwired: 9 in, 1 out]
          }
          frame "ShowGuides" {
            w1491 = "ShowGuides" ("item tag")
            # "Toggle menu checkmark"
            n450 = Get Menu Item Info(7:w1491, 11:w1490) -> (1:w1489:bool, 2:w1493:string, 3:w1494:refnum<k9>, 4:w1488:bool, 6:w1492:T21)  [unwired: 1 in, 2 out]
            n451 = Not(x=w1488) -> (.not. x?=w1487:bool)
            n452 = Set Menu Item Info(4:w1492, 6:w1487, 7:w1491, 9:w1489, 10:w1493, 11:w1494) -> ()  [unwired: 1 in, 2 out]
            n453 = call "grid_and_guides.vi"("Boolean"=w1487, "Operation"=T14."Set guide visibility") -> ()  [unwired: 9 in, 1 out]
          }
          frame "ConfigureGridAndGuides" {
            n454 = call "grid_and_guides.vi"("Operation"=T14."Show front panel") -> ()  [unwired: 10 in, 1 out]
          }
          frame "ShowSettings" {
            n455 = call "UDP Sender generic_2.vi"("Show panel"=TRUE, "Spots"=w1501) -> ()  [unwired: 1 in, 1 out]
          }
          frame "CameraSettings" {
            n456 = global read "red_tweezers_globals_INTERNAL_VOLATILE.vi" "Current Camera VI"() -> (w1504:path)
            n457 = Open VI Reference(vi path=w1504) -> (vi reference=w1503:refnum<vi>)  [unwired: 5 in, 1 out]
            n458 = property class="VI"(reference=w1503, "Front Panel.Open"=TRUE ("Front Panel Window:Open")) -> ()  [unwired: 1 in, 2 out]
          }
          frame Default {
          }
        }
      }
      event Mouse Down? {
        # "We don't process clicks when the user is on the video tab, so that we can set ROIs."
        # "When the mouse button goes down over the image, we save where it went down, etc. and wait to see what happens next.  We also register to be told when the mouse leaves the control, goes up, or moves.  \"click\" or \"drag\" are only detected once the mouse moves or goes up."
        n459 = event-data() -> ("Coords"=w1524:T22, "Button"=w1519:u16, "Mods"=w1528:cluster{"Double Click":bool, "Menu Key":bool}, "PlatMods"=w1527:T23)  [unwired: 1 in]
        n460 = call "mouse_to_image_coords.vi"("Mouse Coords (screen/pane units)"=w1524, "Image Control"=w1520) -> ("Cursor is on Display Area"=w1518:bool, "Mouse Coords (image pixels)"=w1523:cluster{dbl, dbl})  [unwired: 4 in]
        n461 = disable-structure shown="Enabled" {
          disable-tunnel: w1519 -> [w1536 _]
          disable-tunnel: w1518 -> [w1534 w1537]
          disable-tunnel: [w1533 w1537] -> w1514
          frame Enabled {
            n462 = Equal?(x=u16 1, y=w1536) -> (x = y?=w1535:bool)
            n463 = And(x=w1534, y=w1535) -> (x .and. y?=w1533:bool)
          }
          frame Disabled {
            # "use other pane to allow right-clicking on image"
          }
        }
        n464 = local read "Tab"() -> (w1515:T5)
        n465 = Not Equal?(x=w1515, y=T15."Video" ("Tab")) -> (x != y?=w1513:bool)
        n466 = And(x=w1514, y=w1513) -> (x .and. y?=w1512:bool)
        n467 = case shown="False" w1512 {
          tunnel: w1531 -> [w1540 w1551]
          tunnel: [T11 {"Button Down"=FALSE, "Dragging"=FALSE, "Position (Image Pixels)"={"X"=0.0, "Y"=0.0}, "Previous Position (Image Pixels)"={"X"=0.0, "Y"=0.0}, "Button"=0, "Mods"={"Double Click"=FALSE, "Menu Key"=FALSE}, "PlatMods"={"Shift"=FALSE, "Ctrl"=FALSE, "Alt"=FALSE, "Cmd"=FALSE, "Opt"=FALSE}} w1550] -> w1530
          tunnel: [w1540 w1547] -> w1529
          tunnel: w1519 -> [_ w1546]
          tunnel: w1528 -> [_ w1545]
          tunnel: w1527 -> [_ w1544]
          tunnel: w1523 -> [_ w1543]
          tunnel: [FALSE TRUE] -> w1522
          tunnel: w1520 -> [_ w1541]
          frame False {
            # "If the user clicked on a scrollbar, ignore it and let LabVIEW handle it. (this keeps the scrollbars working)"
          }
          frame True {
            w1549 = FALSE  # Dragging
            w1548 = TRUE  # Button Down
            n468 = register-events(reference=w1551, w1541, w1541, w1541, w1541) -> (reference out=w1547:refnum<event-registration>)  [unwired: 1 in, 1 out]
            n469 = Bundle("Button Down"=w1548, "Dragging"=w1549, "Mouse Coords (image pixels)"=w1543, "Mouse Coords (image pixels)"=w1543, "Button"=w1546, "Mods"=w1545, "PlatMods"=w1544) -> (w1550:T24)  [unwired: 1 in]
          }
        }
        n470 = Array Size(array=w1510) -> (size(s)=w1511:i32)
        n471 = local write "# of Spots"(w1511) -> ()
        n472 = local write "Selection/Group"(w1510) -> ()
        n473 = event-data("Discard?"=w1522) -> ()  [unwired: 4 in, 1 out]
      }
      event Mouse Leave {
        w1558 = refnum<vi> refnum  # Dummy
        # "When the mouse leaves, we reset things."
        n474 = event-data() -> ()  [unwired: 1 in, 2 out]
        n475 = register-events(reference=w1559, w1557, w1558, w1558, w1558) -> (reference out=w1556:refnum<event-registration>)  [unwired: 1 in, 1 out]
      }
      event Mouse Up {
        w1578 = refnum<vi> refnum  # Dummy
        # "Double clicking adds a spot at the mouse position."
        # "deregister"
        # "If we get here the mouse has gone down and up again.  If we've not moved in between, we have a Click.\nEither way we're no longer interested in mouse leave/move/up events."
        n476 = event-data() -> ("Mods"=w1565:cluster{"Double Click":bool, "Menu Key":bool})  [unwired: 1 in, 5 out]
        n477 = Unbundle By Name(w1571) -> ("Dragging"=w1580:bool)
        n478 = Unbundle By Name(w1565) -> ("Double Click"=w1562:bool)
        n479 = Not(x=w1580) -> (.not. x?=w1579:bool)
        n480 = Not(x=w1567) -> (.not. x?=w1569:bool)
        n481 = And(x=w1579, y=w1569) -> (x .and. y?=w1563:bool)
        n482 = case shown="True" w1563 {
          tunnel: w1571 -> [_ w1586]
          tunnel: w1573 -> [w1581 w1585]
          tunnel: w1572 -> [w1582 w1588]
          tunnel: [w1582 w1587] -> w1574
          tunnel: w1562 -> [_ w1583]
          tunnel: [w1581 w1584] -> w1564
          frame False {
          }
          frame True {
            n483 = case shown="True" w1583 {
              tunnel: w1588 -> [w1595 w1645]
              tunnel: [w1593 w1651] -> w1587
              tunnel: w1585 -> [w1589 w1652]
              tunnel: w1586 -> [w1592 w1647]
              tunnel: [w1589 w1643] -> w1584
              frame False {
                w1599 = 400.0  # 20^2 px
                # "If the user clicked, determine which spots should be selected: if we've clicked a spot/group then select it.  Shift-clicking toggles selection for that spot, and leaves the rest of the selection unchanged."
                # "check we're close enough"
                # "find closest"
                n484 = Unbundle By Name(w1592) -> ("Position (Image Pixels)"=w1591:cluster{"X":dbl, "Y":dbl}, "PlatMods.Shift"=w1590:bool)
                n485 = for {
                  tunnel: [w1635] -> w1597 mode=indexing
                  tunnel: w1591 -> [w1634]
                  tunnel: w1589 -> [w1633] mode=indexing
                  # "calculate distances between mouse position and spot positions"
                  n486 = call "extract_position.vi"("Spot"=w1633) -> ("Position"=w1632:cluster{"x":dbl, "y":dbl, "z":dbl})
                  n487 = call "coords_real_to_image_currentview.vi"("Position (real coords)"=w1632) -> ("Position (pixels, relative to the top left of the image)"=w1631:cluster{dbl, dbl})  [unwired: 7 in, 1 out]
                  n488 = Subtract(x=w1631, y=w1634) -> (x-y=w1638:cluster{dbl, dbl})
                  n489 = Multiply(x=w1638, y=w1638) -> (x*y=w1637:cluster{dbl, dbl})
                  n490 = Cluster To Array(cluster=w1637) -> (array=w1636:dbl[])
                  n491 = Add Array Elements(numeric array=w1636) -> (sum=w1635:dbl)
                }
                n492 = Array Max & Min(array=w1597) -> (min value=w1598:dbl, min index (indices)=w1594:i32)  [unwired: 2 out]
                n493 = Less Or Equal?(x=w1598, y=w1599) -> (x <= y?=w1596:bool)
                n494 = case shown="True" w1596 {
                  tunnel: w1595 -> [w1600 w1607]
                  tunnel: w1594 -> [_ w1601]
                  tunnel: w1590 -> [_ w1603]
                  tunnel: [w1600 w1602] -> w1593
                  frame False {
                    # "If we didn't click a spot, do nothing."
                  }
                  frame True {
                    # "If the spot is in a group, act on all spots in that group, not just the spot we clicked."
                    # "This case statement toggles the selection of the spot/group we clicked, and leaves other spots unchanged if we're holding shift.  Otherwise, we select the spot/group that was clicked and deselect everything else."
                    n495 = stacked-sequence {
                      tunnel: w1601 -> [_ w1609]
                      frame #0 {
                        n496 = local read "Current Spot #"() -> (→"Prev Current Spot":dbl)
                      }
                      frame #1 {
                        "Current Spot #" <- w1609
                      }
                    }
                    n497 = Index Array(array=w1607, index=w1601) -> (element=w1606:T8)
                    n498 = Unbundle(w1606) -> ("Group ID"=w1604:i32)  [unwired: 1 out]
                    n499 = Greater Than 0?(x=w1604) -> (x > 0?=w1605:bool)
                    n500 = for {
                      tunnel: w1607 -> [w1620] mode=indexing
                      tunnel: w1605 -> [w1617]
                      tunnel: w1604 -> [w1616]
                      tunnel: w1601 -> [w1615]
                      tunnel: w1603 -> [w1613]
                      tunnel: [w1611] -> w1602 mode=indexing
                      i -> [w1614]
                      n501 = Unbundle(w1620) -> ("Group ID"=w1610:i32, "Selected"=w1618:bool)
                      n502 = case shown="True" w1617 {
                        tunnel: w1610 -> [_ w1624]
                        tunnel: [w1622 w1626] -> w1612
                        tunnel: w1616 -> [_ w1625]
                        tunnel: w1615 -> [w1623 _]
                        tunnel: w1614 -> [w1621 _]
                        frame False {
                          n503 = Equal?(x=w1621, y=w1623) -> (x = y?=w1622:bool)
                        }
                        frame True {
                          n504 = Equal?(x=w1624, y=w1625) -> (x = y?=w1626:bool)
                        }
                      }
                      n505 = case shown="True" w1613 {
                        tunnel: [w1627 w1628] -> w1619
                        tunnel: w1618 -> [_ w1629]
                        tunnel: w1612 -> [w1627 w1630]
                        frame False {
                        }
                        frame True {
                          n506 = Exclusive Or(1:w1630, 2:w1629) -> (0:w1628:bool)
                        }
                      }
                      n507 = Bundle("Group ID"=w1610, w1619) -> (w1611:cluster{"Group ID":i32, bool})  [unwired: 1 out]
                    }
                  }
                }
              }
              frame True {
                # "convert mouse position to real coords, and add a spot there."
                # "Double-click detected"
                n508 = Unbundle By Name(w1647) -> ("Position (Image Pixels)"=w1646:cluster{"X":dbl, "Y":dbl})
                n509 = for {
                  tunnel: w1645 -> [w1655] mode=indexing
                  tunnel: [w1654] -> w1644 mode=indexing
                  n510 = Bundle(cluster=w1655, "Selected"=FALSE) -> (w1654:T8)  [unwired: 1 in]
                }
                n511 = call "coords_image_to_real_currentimage.vi"("Position (pixels on image)"=w1646) -> ("Position (real coords)"=w1648:cluster{dbl, dbl, "Z":dbl})  [unwired: 9 in]
                n512 = call "replace_position.vi"("Position"=w1648) -> ("Spot"=w1650:T2)  [unwired: 3 in]
                n513 = Build Array (concatenate)(w1652, w1650) -> (w1643:T2[])
                n514 = Build Array (concatenate)(w1644, T8 {"Group ID"=0, "Selected"=TRUE} ("selection_element")) -> (w1651:T8[])
                n515 = Array Size(array=w1643) -> (size(s)=w1642:i32)
                n516 = local write "Induce check"(TRUE) -> ()
                n517 = Subtract(x=w1642, y=1) -> (x-y=w1641:i32)
                n518 = local write "Current Spot #"(w1641) -> ()
              }
            }
          }
        }
        n519 = register-events(reference=w1576, w1575, w1578, w1578, w1578) -> (reference out=w1577:refnum<event-registration>)  [unwired: 1 in, 1 out]
      }
      event Mouse Move {
        n520 = event-data() -> ("Coords"=w1670:T22)  [unwired: 1 in, 2 out]
        n521 = call "mouse_to_image_coords.vi"("Mouse Coords (screen/pane units)"=w1670, "Image Control"=w1669) -> ("Mouse Coords (image pixels)"=w1661:cluster{dbl, dbl})  [unwired: 4 in, 1 out]
        n522 = Not(x=w1660) -> (.not. x?=w1665:bool)
        n523 = case shown="True" w1665 {
          tunnel: w1663 -> [_ w1683]
          tunnel: w1668 -> [w1675 w1685]
          tunnel: w1667 -> [w1674 w1684]
          tunnel: [w1674 w1684] -> w1656
          tunnel: [w1675 w1686] -> w1666
          tunnel: w1661 -> [_ w1677]
          tunnel: w1657 -> [_ w1676]
          frame False {
          }
          frame True {
            # "this is the displacement of the mouse, since the last iteration, in \"real\" coordinates (NB the conversions go before subtracting, as it may involve adding a constant as well as multiplying, which would confuse things as we're only interested in displacements here."
            # "The \"position\" local variable is there just in case we're on the \"current spot\" tab, so that the position updates nicely"
            # "If the user is dragging, translate the spots.\nHolding down shift causes the mouse's motion to be transformed into scaling about the centroid of the spots and rotation about the same point"
            n524 = Unbundle By Name(w1683) -> ("Position (Image Pixels)"=w1678:cluster{"X":dbl, "Y":dbl})
            n525 = call "find_centroid.vi"("Selection and Groups"=w1684, "Spots"=w1685) -> ("centroid"=w1679:cluster{"x":dbl, "y":dbl, "z":dbl})  [unwired: 2 in, 4 out]
            n526 = Unbundle By Name(w1683) -> ("PlatMods.Shift"=w1682:bool)
            n527 = disable-structure shown="Disabled" {
              disable-tunnel: w1679 -> [w1687 _]
              frame Disabled {
                n528 = local write "Position"(w1687) -> ()
              }
              frame Enabled {
              }
            }
            n529 = call "coords_image_to_real_currentimage.vi"("Position (pixels on image)"=w1677) -> ("Position (real coords)"=w1680:cluster{dbl, dbl, "Z":dbl})  [unwired: 9 in]
            n530 = call "coords_image_to_real_currentimage.vi"("Position (pixels on image)"=w1678) -> ("Position (real coords)"=w1681:cluster{dbl, dbl, "Z":dbl})  [unwired: 9 in]
            n531 = case shown="False" w1682 {
              tunnel: [w1692 w1966] -> w1686
              tunnel: w1685 -> [w1698 w1967]
              tunnel: w1684 -> [w1697 w1965]
              tunnel: w1681 -> [w1696 w1952]
              tunnel: w1679 -> [_ w1962]
              tunnel: w1680 -> [w1693 w1953]
              tunnel: w1676 -> [_ _]
              frame False {
                # "Spot Checker passes on information for the bubble collision,system so proper calculations can be made."
                n532 = while {
                  tunnel: w1696 -> [w1737]
                  tunnel: [w1727] -> w1694
                  tunnel: w1693 -> [w1726]
                  i -> [w1720]
                  stop <- w1722 stop-if-true
                  w1712 = 0
                  # "This while loop statement makes sure\nthat every spot gets checked before \nallowing any spot to move."
                  # "Buffer zone controls the amount of space between the\ncenter of a spot compared to the center of another spot.\nThis is used to prevent bubbles from colliding with each other."
                  # "Projected distance calculates the distance between two spots- this is used for when a \"hit\" occurs. If the projected distance becomes larger than the previous distance, the program will assume that the spot is being pulled from the buffer zone and as a result will allow the bubble to exit."
                  # "This subVI leads to the distance function, which outputs the distance between a spot being checked compared to the current spot number."
                  n533 = control-ref of="Value Check"() -> (w1717:refnum<vi>)
                  n534 = control-ref of="ID num check"() -> (w1716:refnum<vi>)
                  n535 = control-ref of="Spot Checker"() -> (w1733:refnum<vi>)
                  n536 = Subtract(x=w1726, y=w1737) -> (x-y=w1727:cluster{dbl, dbl, "Z":dbl})
                  n537 = call "DistanceFunction.vi"("Condition Driver"=FALSE, "Position (real coords)"=w1737, "Current Spot Number"=w1716, "Spot Checker"=w1733, "Spot Number Being Checked"=w1717) -> ("Distance"=w1701:dbl)  [unwired: 6 in]
                  n538 = stacked-sequence {
                    tunnel: w1701 -> [_ w1742]
                    frame #0 {
                      n539 = local read "Distance"() -> (→"Previous Distance":dbl)
                    }
                    frame #1 {
                      "Distance" <- w1742
                    }
                  }
                  n540 = Unbundle(w1727) -> (→"X Displacement":dbl, →"Y Displacement":dbl)  [unwired: 1 out]
                  n541 = control-ref of="ID num check"() -> (w1718:refnum<vi>)
                  n542 = control-ref of="Spot Checker"() -> (w1731:refnum<vi>)
                  n543 = control-ref of="Y Displacement"() -> (w1729:refnum<vi>)
                  n544 = control-ref of="Value Check"() -> (w1719:refnum<vi>)
                  n545 = control-ref of="X Displacement"() -> (w1730:refnum<vi>)
                  n546 = call "ProjectedDistance.vi"("X Displacement"=w1730, "Spot Number Check"=w1719, "Current Spot #"=w1718, "Spot Checker"=w1731, "Y Displacement"=w1729) -> ("Numeric"=→"Projected Distance":dbl)  [unwired: 6 in]
                  n547 = Multiply(x="Buffer Zone", y=2) -> (x*y=w1736:dbl)
                  n548 = local read "ID num check"() -> (w1713:dbl)
                  n549 = local read "Value Check"() -> (w1714:dbl)
                  n550 = local read "Projected Distance"() -> (w1705:dbl)
                  n551 = Equal?(x=w1701, y=0) -> (x = y?=w1702:bool)
                  n552 = case shown="False" w1702 {
                    frame False {
                      n553 = local read "Hit"() -> (w1739:bool)
                      n554 = local write "Hit Indicator"(w1739) -> ()
                    }
                    frame True {
                      "Hit Indicator" <- FALSE
                    }
                  }
                  n555 = Not Equal?(x=w1705, y=0) -> (x != y?=w1703:bool)
                  n556 = Less Or Equal?(x=w1701, y=w1736) -> (x <= y?=w1706:bool)
                  n557 = Equal?(x=w1713, y=w1712) -> (x = y?=w1711:bool)
                  n558 = And(x=w1706, y=w1703) -> (x .and. y?=w1699:bool)
                  "Hit" <- w1699
                  n559 = Equal?(x=w1712, y=w1714) -> (x = y?=w1710:bool)
                  n560 = Not(x=w1699) -> ()  [unwired: 1 out]
                  n561 = And(x=w1711, y=w1710) -> (x .and. y?=w1709:bool)
                  n562 = Or(x=w1699, y=w1709) -> (x .or. y?=w1715:bool)
                  n563 = case shown="False" w1715 {
                    frame False {
                      n564 = stacked-sequence {
                        frame #0 {
                          n565 = local read "Potential Collisions"() -> (w1745:dbl)
                          n566 = local read "Spot # Check"() -> (w1747:dbl)
                          n567 = Subtract(x=w1745, y=1) -> (x-y=w1743:dbl)
                          n568 = Less Or Equal?(x=w1747, y=w1743) -> (x <= y?=w1746:bool)
                          n569 = case shown="True" w1746 {
                            frame False {
                              # "Spot # Check resets if the the number of potential collisons is more than Spot # Check."
                              n570 = local write "Spot # Check"(0) -> ()
                            }
                            frame True {
                              n571 = stacked-sequence {
                                frame #0 {
                                # "Spot # Check increments by 1 every time it is greater than the # of potential collisions."
                                n572 = local read "Spot # Check"() -> (w1751:dbl)
                                n573 = Add(x=w1751, y=1) -> (x+y=→"Spot # Check":dbl)
                                }
                                frame #1 {
                                # "Spot # Check resets if the Spot # Check is eqaul to the # of potential collisions."
                                n574 = local read "Potential Collisions"() -> (w1752:dbl)
                                n575 = local read "Spot # Check"() -> (w1753:dbl)
                                n576 = Equal?(x=w1753, y=w1752) -> (x = y?=w1754:bool)
                                n577 = case shown="True" w1754 {
                                frame False {
                                }
                                frame True {
                                n578 = local write "Spot # Check"(0) -> ()
                                }
                                }
                                }
                                frame #2 {
                                n579 = local read "Spot Checker"() -> (w1769:T2[])
                                n580 = local read "Current Spot #"() -> (w1770:dbl)
                                n581 = local read "Area to check"() -> (w1756:dbl)
                                n582 = Index Array(array=w1769, index=w1770) -> (element=w1768:T2)
                                n583 = local read "Orig Y SC"() -> (w1765:dbl)
                                n584 = Unbundle By Name(w1768) -> ("Position.x"=w1766:dbl, "Position.y"=w1764:dbl)
                                n585 = local read "Orig X SC"() -> (w1767:dbl)
                                n586 = Subtract(x=w1764, y=w1765) -> (x-y=w1757:dbl)
                                n587 = Absolute Value(x=w1757) -> (abs(x)=w1758:dbl)
                                n588 = Subtract(x=w1766, y=w1767) -> (x-y=w1760:dbl)
                                n589 = Greater?(x=w1758, y=w1756) -> (0:w1762:bool)
                                n590 = Absolute Value(x=w1760) -> (abs(x)=w1759:dbl)
                                n591 = Greater?(x=w1759, y=w1756) -> (0:w1761:bool)
                                n592 = Or(x=w1761, y=w1762) -> (x .or. y?=w1763:bool)
                                n593 = case shown="True" w1763 {
                                frame False {
                                }
                                frame True {
                                n594 = stacked-sequence {
                                frame #0 {
                                n595 = local read "Null array"() -> (w1775:dbl[])
                                n596 = local write "What to Check"(w1775) -> ()
                                n597 = local write "ID"(w1775) -> ()
                                n598 = local read "Current Spot #"() -> (w1777:dbl)
                                n599 = local write "Potential Collisions"(0) -> ()
                                n600 = local read "Spot Checker"() -> (w1776:T2[])
                                n601 = Index Array(array=w1776, index=w1777) -> (element=w1778:T2)
                                n602 = Wait (ms)(milliseconds to wait=100) -> ()  [unwired: 1 out]
                                n603 = Unbundle By Name(w1778) -> ("Position.x"=w1772:dbl, "Position.y"=w1773:dbl)
                                n604 = local write "Orig Y SC"(w1773) -> ()
                                n605 = local write "Orig X SC"(w1772) -> ()
                                }
                                frame #1 {
                                # "All this is a  statement checking whether the microrobot is within the area being checked using absolute value statements. The number of potential collisions gets added by 1 every time a bubble is detected within the area."
                                n606 = local read "# of Spots"() -> (w1779:dbl)
                                n607 = for {
                                N: w1779 -> [_]
                                tunnel: w1779 -> [w1784]
                                i -> [w1780]
                                n608 = local read "Selection/Group"() -> (w1783:T8[])
                                n609 = Index Array(array=w1783, index=w1780) -> (element=w1782:T8)
                                n610 = Unbundle By Name(w1782) -> ("Selected"=w1781:bool)
                                n611 = case shown="True" w1781 {
                                tunnel: w1784 -> [_ w1786]
                                tunnel: w1780 -> [_ w1785]
                                frame False {
                                }
                                frame True {
                                n612 = for {
                                N: w1786 -> [_]
                                tunnel: w1785 -> [w1787]
                                i -> [w1788]
                                n613 = local read "Selection/Group"() -> (w1792:T8[])
                                n614 = Index Array(array=w1792, index=w1788) -> (element=w1791:T8)
                                n615 = Unbundle By Name(w1791) -> ("Selected"=w1789:bool)
                                n616 = Not(x=w1789) -> (.not. x?=w1790:bool)
                                n617 = case shown="True" w1790 {
                                tunnel: w1788 -> [_ w1796]
                                tunnel: w1787 -> [_ w1795]
                                tunnel: w1787 -> [_ w1794]
                                frame False {
                                }
                                frame True {
                                n618 = local read "Spot Checker"() -> (w1813:T2[])
                                n619 = Index Array(array=w1813, index=w1796) -> (element=w1814:T2)
                                n620 = Index Array(array=w1813, index=w1795) -> (element=w1812:T2)
                                n621 = Unbundle By Name(w1812) -> ("Position.x"=w1809:dbl, "Position.y"=w1805:dbl)
                                n622 = Unbundle By Name(w1814) -> ("Position.x"=w1806:dbl, "Position.y"=w1802:dbl)
                                n623 = local read "Area+ Buffer"() -> (w1793:dbl)
                                n624 = Subtract(x=w1809, y=w1793) -> (x-y=w1810:dbl)
                                n625 = Greater Or Equal?(x=w1806, y=w1810) -> (x >= y?=w1811:bool)
                                n626 = Add(x=w1805, y=w1793) -> (x+y=w1804:dbl)
                                n627 = Subtract(x=w1805, y=w1793) -> (x-y=w1803:dbl)
                                n628 = Add(x=w1809, y=w1793) -> (x+y=w1807:dbl)
                                n629 = Less Or Equal?(x=w1802, y=w1804) -> (x <= y?=w1801:bool)
                                n630 = Greater Or Equal?(x=w1802, y=w1803) -> (x >= y?=w1800:bool)
                                n631 = Less Or Equal?(x=w1806, y=w1807) -> (x <= y?=w1808:bool)
                                n632 = And(x=w1811, y=w1808) -> (x .and. y?=w1798:bool)
                                n633 = And(x=w1801, y=w1800) -> (x .and. y?=w1799:bool)
                                n634 = And(x=w1798, y=w1799) -> (x .and. y?=w1797:bool)
                                n635 = case shown="True" w1797 {
                                tunnel: w1796 -> [_ _]
                                tunnel: w1796 -> [_ w1816]
                                tunnel: w1794 -> [_ w1815]
                                frame False {
                                }
                                frame True {
                                n636 = stacked-sequence {
                                tunnel: w1816 -> [w1817 _]
                                tunnel: w1815 -> [w1818 _]
                                frame #0 {
                                n637 = local read "Potential Collisions"() -> (w1821:dbl)
                                n638 = local read "What to Check"() -> (w1822:dbl[])
                                n639 = Insert Into Array(array=w1822, index=w1821, new element=w1817) -> (w1823:dbl[])
                                n640 = local read "ID"() -> (w1820:dbl[])
                                n641 = local write "What to Check"(w1823) -> ()
                                n642 = Insert Into Array(array=w1820, index=w1821, new element=w1818) -> (w1819:dbl[])
                                n643 = local write "ID"(w1819) -> ()
                                }
                                frame #1 {
                                n644 = local read "Potential Collisions"() -> (w1826:dbl)
                                n645 = Add(x=w1826, y=1) -> (x+y=w1824:dbl)
                                n646 = local write "Potential Collisions"(w1824) -> ()
                                }
                                }
                                }
                                }
                                }
                                }
                                }
                                }
                                }
                                }
                                }
                                frame #2 {
                                n647 = local read "Current Spot #"() -> (w1827:dbl)
                                n648 = local write "Prev Current Spot"(w1827) -> ()
                                }
                                }
                                }
                                }
                                }
                              }
                            }
                          }
                        }
                        frame #1 {
                          # "This updates the ID and Value being checked at the beginning of IDs and values being checked."
                          n649 = local read "Spot # Check"() -> (w1830:dbl)
                          n650 = local read "What to Check"() -> (w1831:dbl[])
                          n651 = local read "ID"() -> (w1832:dbl[])
                          n652 = Index Array(array=w1832, index=w1830) -> (element=w1829:dbl)
                          n653 = Index Array(array=w1831, index=w1830) -> (element=w1828:dbl)
                          n654 = local write "Value Check"(w1828) -> ()
                          n655 = local write "ID num check"(w1829) -> ()
                        }
                      }
                    }
                    frame True {
                      n656 = stacked-sequence {
                        frame #0 {
                          # "This section activate a case statement which allows us to change the area being checked. Orig X/Y SC holds the position of the area to check and changes after the bubble exits the area beig checked."
                          # "This statement controls the areas selected and finds which bubbles needs to be checked. This activates when the bubble\nmoves out of the area specified."
                          n657 = local read "# of Spots"() -> (w1852:dbl)
                          n658 = local read "Current Spot #"() -> (w1851:dbl)
                          n659 = Subtract(x=w1852, y=1) -> (x-y=w1853:dbl)
                          n660 = Equal?(x=w1851, y=w1853) -> (x = y?=w1849:bool)
                          n661 = case shown="True" w1849 {
                            tunnel: [w1912 w1915] -> w1850
                            frame True {
                              n662 = local read "# of Spots"() -> (w1913:dbl)
                              n663 = Subtract(x=w1913, y=2) -> (x-y=w1912:dbl)
                            }
                            frame False {
                              n664 = local read "# of Spots"() -> (w1914:dbl)
                              n665 = Subtract(x=w1914, y=1) -> (x-y=w1915:dbl)
                            }
                          }
                          "Maximum" <- w1850
                          n666 = local read "Spot Checker"() -> (w1848:T2[])
                          n667 = local read "Current Spot #"() -> (w1847:dbl)
                          n668 = Index Array(array=w1848, index=w1847) -> (element=w1846:T2)
                          n669 = Unbundle By Name(w1846) -> ("Position.x"=w1845:dbl, "Position.y"=w1844:dbl)
                          n670 = local read "Orig Y SC"() -> (w1842:dbl)
                          n671 = local read "Orig X SC"() -> (w1843:dbl)
                          n672 = Subtract(x=w1844, y=w1842) -> (x-y=w1839:dbl)
                          n673 = Subtract(x=w1845, y=w1843) -> (x-y=w1841:dbl)
                          n674 = Absolute Value(x=w1839) -> (abs(x)=w1838:dbl)
                          n675 = Absolute Value(x=w1841) -> (abs(x)=w1840:dbl)
                          n676 = local read "Area to check"() -> (w1834:dbl)
                          n677 = local read "Area to check"() -> (w1833:dbl)
                          n678 = Greater?(x=w1840, y=w1834) -> (0:w1837:bool)
                          n679 = Greater?(x=w1838, y=w1833) -> (0:w1836:bool)
                          n680 = Or(x=w1837, y=w1836) -> (x .or. y?=w1835:bool)
                          n681 = case shown="True" w1835 {
                            frame False {
                            }
                            frame True {
                              n682 = stacked-sequence {
                                frame #0 {
                                # "A small time delay of 100 ms is provided to allow the data to pass throguh properly."
                                n683 = Wait (ms)(milliseconds to wait=100) -> ()  [unwired: 1 out]
                                n684 = local read "Null array"() -> (→"What to Check" →"ID":dbl[])
                                n685 = local read "Spot Checker"() -> (w1860:T2[])
                                n686 = local read "Current Spot #"() -> (w1859:dbl)
                                n687 = Index Array(array=w1860, index=w1859) -> (element=w1858:T2)
                                n688 = Unbundle By Name(w1858) -> ("Position.x"=→"Orig X SC":dbl, "Position.y"=→"Orig Y SC":dbl)
                                "Potential Collisions" <- 0
                                }
                                frame #1 {
                                n689 = local read "# of Spots"() -> (w1863:dbl)
                                n690 = for {
                                N: w1863 -> [_]
                                tunnel: w1863 -> [w1868]
                                i -> [w1864]
                                n691 = local read "Selection/Group"() -> (w1867:T8[])
                                n692 = Index Array(array=w1867, index=w1864) -> (element=w1866:T8)
                                n693 = Unbundle By Name(w1866) -> ("Selected"=w1865:bool)
                                n694 = case shown="True" w1865 {
                                tunnel: w1868 -> [_ w1870]
                                tunnel: w1864 -> [_ w1869]
                                frame False {
                                }
                                frame True {
                                n695 = for {
                                N: w1870 -> [_]
                                tunnel: w1869 -> [w1871]
                                i -> [w1872]
                                n696 = local read "Selection/Group"() -> (w1876:T8[])
                                n697 = Index Array(array=w1876, index=w1872) -> (element=w1875:T8)
                                n698 = Unbundle By Name(w1875) -> ("Selected"=w1873:bool)
                                n699 = Not(x=w1873) -> (.not. x?=w1874:bool)
                                n700 = case shown="True" w1874 {
                                tunnel: w1872 -> [_ w1880]
                                tunnel: w1871 -> [_ w1879]
                                tunnel: w1871 -> [_ w1878]
                                frame False {
                                }
                                frame True {
                                n701 = local read "Spot Checker"() -> (w1897:T2[])
                                n702 = Index Array(array=w1897, index=w1880) -> (element=w1898:T2)
                                n703 = Index Array(array=w1897, index=w1879) -> (element=w1896:T2)
                                n704 = Unbundle By Name(w1896) -> ("Position.x"=w1893:dbl, "Position.y"=w1889:dbl)
                                n705 = Unbundle By Name(w1898) -> ("Position.x"=w1890:dbl, "Position.y"=w1886:dbl)
                                n706 = local read "Area+ Buffer"() -> (w1877:dbl)
                                n707 = Subtract(x=w1893, y=w1877) -> (x-y=w1894:dbl)
                                n708 = Greater Or Equal?(x=w1890, y=w1894) -> (x >= y?=w1895:bool)
                                n709 = Add(x=w1889, y=w1877) -> (x+y=w1888:dbl)
                                n710 = Subtract(x=w1889, y=w1877) -> (x-y=w1887:dbl)
                                n711 = Add(x=w1893, y=w1877) -> (x+y=w1891:dbl)
                                n712 = Less Or Equal?(x=w1886, y=w1888) -> (x <= y?=w1885:bool)
                                n713 = Greater Or Equal?(x=w1886, y=w1887) -> (x >= y?=w1884:bool)
                                n714 = Less Or Equal?(x=w1890, y=w1891) -> (x <= y?=w1892:bool)
                                n715 = And(x=w1895, y=w1892) -> (x .and. y?=w1882:bool)
                                n716 = And(x=w1885, y=w1884) -> (x .and. y?=w1883:bool)
                                n717 = And(x=w1882, y=w1883) -> (x .and. y?=w1881:bool)
                                n718 = case shown="True" w1881 {
                                tunnel: w1880 -> [_ _]
                                tunnel: w1880 -> [_ w1900]
                                tunnel: w1878 -> [_ w1899]
                                frame False {
                                }
                                frame True {
                                n719 = stacked-sequence {
                                tunnel: w1900 -> [w1901 _]
                                tunnel: w1899 -> [w1902 _]
                                frame #0 {
                                n720 = local read "Potential Collisions"() -> (w1905:dbl)
                                n721 = local read "What to Check"() -> (w1906:dbl[])
                                n722 = Insert Into Array(array=w1906, index=w1905, new element=w1901) -> (w1907:dbl[])
                                n723 = local read "ID"() -> (w1904:dbl[])
                                n724 = Insert Into Array(array=w1904, index=w1905, new element=w1902) -> (w1903:dbl[])
                                n725 = local write "What to Check"(w1907) -> ()
                                n726 = local write "ID"(w1903) -> ()
                                }
                                frame #1 {
                                n727 = local read "Potential Collisions"() -> (w1910:dbl)
                                n728 = Add(x=w1910, y=1) -> (x+y=w1908:dbl)
                                n729 = local write "Potential Collisions"(w1908) -> ()
                                }
                                }
                                }
                                }
                                }
                                }
                                }
                                }
                                }
                                }
                                }
                              }
                            }
                          }
                        }
                        frame #1 {
                          n730 = local read "# of Spots"() -> (w1919:dbl)
                          n731 = Not Equal?(x=w1919, y=1) -> (x != y?=w1917:bool)
                          n732 = case shown="True" w1917 {
                            frame False {
                            }
                            frame True {
                              n733 = stacked-sequence {
                                frame #0 {
                                n734 = local read "Potential Collisions"() -> (w1922:dbl)
                                n735 = local read "Spot # Check"() -> (w1924:dbl)
                                n736 = Subtract(x=w1922, y=1) -> (x-y=w1920:dbl)
                                n737 = Less Or Equal?(x=w1924, y=w1920) -> (x <= y?=w1923:bool)
                                n738 = case shown="False" w1923 {
                                frame False {
                                n739 = local write "Spot # Check"(0) -> ()
                                }
                                frame True {
                                }
                                }
                                }
                                frame #1 {
                                n740 = local read "What to Check"() -> (w1930:dbl[])
                                n741 = local read "ID"() -> (w1928:dbl[])
                                n742 = local read "Spot # Check"() -> (w1926:dbl)
                                n743 = Index Array(array=w1930, index=w1926) -> (element=→"Value Check":dbl)
                                n744 = Index Array(array=w1928, index=w1926) -> (element=→"ID num check":dbl)
                                }
                              }
                            }
                          }
                        }
                      }
                    }
                  }
                  n745 = local read "Potential Collisions"() -> (w1707:dbl)
                  n746 = Subtract(x=w1707, y=1) -> (x-y=w1708:dbl)
                  n747 = local read "Hit"() -> (w1725:bool)
                  n748 = Equal?(x=w1720, y=w1708) -> (x = y?=w1724:bool)
                  n749 = Or(x=w1725, y=w1724) -> (x .or. y?=w1722:bool)
                }
                n750 = for {
                  tunnel: w1697 -> [w1944] mode=indexing
                  tunnel: w1698 -> [w1941] mode=indexing
                  tunnel: [w1943] -> w1692 mode=indexing
                  tunnel: w1694 -> [w1942]
                  # "If the projected distance is greater than the\nprevious distance, then the selected spots will move. \nThis situation only occurs if the bubble is about to/crossing \nthe buffer zone of another bubble. \n\nThe selected spots will also move if none of the bubbles\nare near/crossing the buffer zone of another bubble."
                  n751 = local read "Hit"() -> (w1934:bool)
                  n752 = Unbundle By Name(w1941) -> ()  [unwired: 1 out]
                  n753 = local read "Projected Distance"() -> (w1933:dbl)
                  n754 = Unbundle(w1944) -> ("Group ID"=→"Group ID #":i32, "Selected"=w1938:bool)
                  n755 = local read "Previous Distance"() -> (w1936:dbl)
                  n756 = Not(x=w1934) -> (.not. x?=w1932:bool)
                  n757 = Greater?(x=w1933, y=w1936) -> (0:w1935:bool)
                  n758 = And(x=w1934, y=w1935) -> (x .and. y?=w1931:bool)
                  n759 = Or(x=w1932, y=w1931) -> (x .or. y?=w1937:bool)
                  n760 = And(x=w1938, y=w1937) -> (x .and. y?=w1939:bool)
                  n761 = case shown="True" w1939 {
                    tunnel: w1941 -> [w1945 w1949]
                    tunnel: [w1945 w1948] -> w1943
                    tunnel: w1942 -> [_ w1950]
                    frame False {
                      # "otherwise, leave it alone!"
                    }
                    frame True {
                      # "If the spot is selected, move it by the same amount as the mouse"
                      n762 = call "extract_position.vi"("Spot"=w1949) -> ("Position"=w1947:cluster{"x":dbl, "y":dbl, "z":dbl})
                      n763 = Add(x=w1947, y=w1950) -> (x+y=w1946:cluster{dbl, dbl, dbl})
                      n764 = call "replace_position.vi"("Position"=w1946, "Spot in"=w1949) -> ("Spot"=w1948:T2)  [unwired: 2 out]
                    }
                  }
                }
                "Spot Checker" <- w1692
                n765 = local read "Locked Current Spot"() -> (w1688:dbl)
                n766 = Index Array(array=w1692, index=w1688) -> (element=w1691:T2)
                n767 = Unbundle By Name(w1691) -> ("Position.x"=→"New X":dbl, "Position.y"=→"New Y":dbl)  [unwired: 1 out]
                n768 = Array Size(array=w1692) -> (size(s)=→"# of Spots":i32)
              }
              frame True {
                # "coordinate conversion to find the rotation and scaling done by the mouse, about the centroid of the spots"
                n769 = Subtract(x=w1952, y=w1962) -> (x-y=w1971:cluster{dbl, dbl, dbl})
                n770 = Subtract(x=w1953, y=w1962) -> (x-y=w1970:cluster{dbl, dbl, dbl})
                n771 = Unbundle(w1970) -> (w1956:dbl, w1957:dbl)  [unwired: 1 out]
                n772 = Unbundle(w1971) -> (w1961:dbl, w1960:dbl)  [unwired: 1 out]
                n773 = Re/Im To Polar(2:w1957, 3:w1956) -> (0:w1954:dbl, 1:w1955:dbl)
                n774 = Re/Im To Polar(2:w1960, 3:w1961) -> (0:w1958:dbl, 1:w1959:dbl)
                n775 = Divide(x=w1955, y=w1959) -> (x/y=w1951:dbl)
                n776 = Subtract(x=w1954, y=w1958) -> (x-y=w1963:dbl)
                n777 = Bundle(w1951, w1951, w1951) -> (w1973:cluster{dbl, dbl, dbl})  [unwired: 1 out]
                n778 = call "scale_matrix.vi"("Scale Factors"=w1973) -> ("Scale Matrix"=w1969:T10)
                n779 = call "arb_rotation_matrix.vi"("Unit Vector"=cluster{dbl, dbl, dbl} {0.0, 0.0, 1.0}, "theta"=w1963) -> ("Real Matrix"=w1968:T10)
                n780 = call-poly <vilib>:"A x B.vi"("B"=w1968, "A"=w1969) -> ("A x B"=w1964:T10)  [unwired: 1 out]
                n781 = for {
                  tunnel: w1967 -> [w1979] mode=indexing
                  tunnel: [w1978] -> w1966 mode=indexing
                  tunnel: w1965 -> [w1977] mode=indexing
                  tunnel: w1962 -> [w1975]
                  tunnel: w1964 -> [w1974]
                  n782 = Unbundle(w1977) -> ("Selected"=w1976:bool)  [unwired: 1 out]
                  n783 = case shown="True" w1976 {
                    tunnel: w1979 -> [w1980 w1984]
                    tunnel: [w1980 w1983] -> w1978
                    tunnel: w1975 -> [_ w1982]
                    tunnel: w1974 -> [_ w1981]
                    frame False {
                    }
                    frame True {
                      n784 = call "apply_matrix_transformation_to_spots.vi"("Transform centre (i.e. transform about this point)"=w1982, "Transformation Matrix (3x3)"=w1981, "Spot In"=w1984) -> ("Spot Out"=w1983:T2)  [unwired: 5 out]
                    }
                  }
                }
              }
            }
          }
        }
        "Selection/Group" <- w1656
        n785 = Unbundle By Name(w1663) -> ("Position (Image Pixels)"=w1662:cluster{"X":dbl, "Y":dbl})
        n786 = Bundle By Name(cluster=w1663, "Dragging"=TRUE, "Previous Position (Image Pixels)"=w1662, "Position (Image Pixels)"=w1661) -> (w1672:T11)
      }
      event "stop": Value Change {
        n787 = event-data() -> ()  [unwired: 1 in, 4 out]
        n788 = global read "red_tweezers_globals_INTERNAL_VOLATILE.vi" "Current Settings File"() -> (w1988:path)
        n789 = call <vilib>:"Check if File or Folder Exists.vi"("path"=w1988) -> ("file or folder exists?"=w1987:bool)  [unwired: 8 in, 2 out]
        n790 = case shown="False" w1987 {
          tunnel: [w1995 w1999] -> w1989
          frame False {
            n791 = Two Button Dialog(message="Save current settings?", 1:"Don't Save" ("F button name (\"Cancel\")"), 2:"Save As..." ("T button name (\"OK\")")) -> (T button?=w1992:bool)
            n792 = Select(t=T16."Center Button" ("Which Button?"), s=w1992, f=T16."Right Button" ("Which Button?")) -> (s? t:f=w1995:T16)
          }
          frame True {
            n793 = call <vilib>:"Three Button Dialog.vi"("Allow user to close window? (TRUE)"=TRUE, "Window Title (\"\")"="Save Settings?" ("Window Title (\"\")"), "Right Button Text (\"Cancel\")"="No" ("Right Button Text (\"Cancel\")"), "Center Button Text (\"No\")"="Save As..." ("Center Button Text (\"No\")"), "Left Button Text (\"Yes\")"="Save" ("Left Button Text (\"Yes\")"), "message"="Would you like to save the current settings? You can choose to use the current settings file or save to a new location.") -> ("Which Button?"=w1999:T16)  [unwired: 5 in]
          }
        }
        n794 = case shown="\"Center Button\"" w1989 {
          tunnel: [TRUE TRUE FALSE FALSE] -> w1986
          frame "Left Button", Default {
          }
          frame "Center Button" {
            n795 = call "File Dialog5"("prompt"="Please select a location to save the settings", "button label"="Save", "default name"="red_tweezers_settings.xml", "pattern (all files)"="*.xml" ("pattern label"), "pattern label"="XML Settings Files") -> ("selected path"=w2007:path)  [unwired: 7 in, 3 out]
            n796 = global write "red_tweezers_globals_INTERNAL_VOLATILE.vi" "Current Settings File"(w2007) -> ()
          }
          frame "Right Button" {
          }
          frame "Window Close" {
          }
        }
        n797 = global write "red_tweezers_globals_INTERNAL_VOLATILE.vi" "Save Settings On Exit"(w1986) -> ()
      }
    }
    n798 = call "Vision Acquisition"() -> ("Image Out"=w32:T9)  [unwired: 24 in, 3 out]
    n799 = call "IMAQ Create"("Image Name"="untitled", "Image Type"=w61) -> ("New Image"=w60:T9)  [unwired: 3 in, 1 out]
    n800 = local read "Number of Matches Returned 2"() -> (w54:dbl)
    n801 = Add(x=w54, y=1.0 ("x+y")) -> (x+y=w58:dbl)
    n802 = for {
      N: w58 -> [_]
      tunnel: w32 -> [w191]
      i -> [w219]
      # "ROI CODE TO SELECT SPECIFIC POINTS"
      n803 = local read "Circles 2"() -> (w206:T1)
      n804 = Number To Decimal String(number=w219) -> (decimal integer string=w218:string)  [unwired: 1 in]
      n805 = Index Array(array=w206) -> (element=w223:T25)  [unwired: 1 in]
      n806 = Unbundle(w223) -> ("Position"=w217:cluster{"X":sgl, "Y":sgl}, "Radius"=w205:dbl)  [unwired: 1 out]
      n807 = property on="Camera 3" class="ImageControl"() -> ("ROI"=w201:T26)  [unwired: 2 in, 2 out]
      n808 = Unbundle(w217) -> ("X"=w221:sgl, "Y"=w220:sgl)
      n809 = Unbundle By Name(w201) -> ("Contours"=w192:T27)
      n810 = Subtract(x=w221, y=w205) -> (x-y=→"toplx 2":dbl)
      n811 = Add(x=w221, y=w205) -> (x+y=→"bottomrx 2":dbl)
      n812 = Add(x=w220, y=w205) -> (x+y=→"bottomry 2":dbl)
      n813 = Subtract(x=w220, y=w205) -> (x-y=→"toply 2":dbl)
      n814 = Index Array(array=w192) -> (element=w193:T28)  [unwired: 1 in]
      n815 = Unbundle By Name(w193) -> ("Points"=w194:i32[])
      n816 = Index Array(array=w194, index #1=0 ("index"), index #2=1 ("index")) -> (element #1=w202:i32, element #2=w203:i32)
      "ROI-X" <- w202
      "ROI-Y" <- w203
      n817 = local read "toply 2"() -> (w209:dbl)
      n818 = local read "bottomrx 2"() -> (w208:dbl)
      n819 = Bundle(w202, w203) -> (w197:cluster{i32, i32})  [unwired: 1 in]
      "Specific Point" <- w197
      n820 = local read "toplx 2"() -> (w210:dbl)
      n821 = local read "bottomry 2"() -> (w207:dbl)
      n822 = Build Array(w210, w209, w208, w207) -> (w215:dbl[])
      n823 = call "IMAQ Overlay Text"("Text Color (black)"=u32 1703680, "Font, Size & Style"=T12 {"Desired Font (Application)"=enum."Application Font", "[User-specified Font]"={"Font Name"="", "Size"=40, "Strikeout?"=FALSE, "Italic?"=FALSE, "Underline?"=FALSE, "Outline?"=FALSE, "Shadow?"=FALSE, "Bold?"=FALSE, "Rotation Angle"=0.0}, "Horizontal Alignment"=0, "Vertical Alignment"=0}, "String"="ROI", "Origin"=w197, "Image"=w191) -> ()  [unwired: 5 in, 2 out]
      n824 = Array To Cluster(array=w215) -> (cluster=w222:T29)
      n825 = call "IMAQ Overlay Oval"("Bounding Rectangle"=w222, "Image"=w191) -> ("Image Out"=w216:T9)  [unwired: 8 in, 1 out]
      n826 = call "IMAQ Overlay Text"("String"=w218, "Origin"=w217, "Image"=w216) -> ("Image Out"=→"Camera 3":T9)  [unwired: 7 in, 1 out]
    }
    n827 = call "IMAQ ExtractSingleColorPlane"("Color Plane"=w59, "Image Dst"=w60, "Image Src"=w32) -> ()  [unwired: 7 in, 2 out]
    n828 = call-poly "IMAQ Detect Shapes"("Circle Descriptor"="Circle Descriptor 2", "Image"=w32) -> ("Number of Matches Returned"=→"Number of Matches Returned 2":i32, "Circles"=→"Circles 2":T1)  [unwired: 7 in, 1 out]
    n829 = case shown="True" "Camera Capture 2" {
      frame False {
      }
      frame True {
        n830 = local read "Circles 2"() -> (w179:T1)
        n831 = Index Array(array=w179) -> (element=w180:T25)  [unwired: 1 in]
        n832 = Index Array(array=w179) -> (element=w190:T25)  [unwired: 1 in]
        n833 = Unbundle(w180) -> ("Position"=w188:cluster{"X":sgl, "Y":sgl}, "Radius"=w181:dbl)  [unwired: 1 out]
        n834 = Unbundle(w190) -> ("Position"=w189:cluster{"X":sgl, "Y":sgl})  [unwired: 2 out]
        n835 = Unbundle(w188) -> ("X"=w186:sgl, "Y"=w187:sgl)
        n836 = Unbundle(w189) -> ("X"=→"Object x":sgl, "Y"=→"Object y":sgl)
        n837 = Subtract(x=w186, y=w181) -> (x-y=→"toplx 3":dbl)
        n838 = Add(x=w186, y=w181) -> (x+y=→"bottomrx 3":dbl)
        n839 = Add(x=w187, y=w181) -> (x+y=→"bottomry 3":dbl)
        n840 = Subtract(x=w187, y=w181) -> (x-y=→"toply 3":dbl)
      }
    }
    n841 = case shown="1" "Numeric 2" {
      frame 0, Default {
        n842 = local read "ROI-X"() -> (w171:dbl)
        n843 = local read "ROI-Y"() -> (w170:dbl)
        n844 = Build Array(w171, w170) -> (w168:T10)
        n845 = call-poly <vilib>:"Multiply.vi"("Real Scalar c"=1e-07 ("y"), "Real Matrix A"=w168) -> ("A * c"=→"ROI 0":T10)
      }
      frame 1 {
        n846 = local read "ROI-X"() -> (w176:dbl)
        n847 = local read "ROI-Y"() -> (w175:dbl)
        n848 = Build Array(w176, w175) -> (w173:T10)
        n849 = call-poly <vilib>:"Multiply.vi"("Real Matrix A"=w173, "Real Scalar c"=1e-07 ("y")) -> ("c * A"=→"ROI 1":T10)
      }
    }
    n850 = local read "Stop"() -> (w64:i32)
    n851 = local read "Start"() -> (w63:i32)
    n852 = Subtract(x=w64, y=w63) -> (x-y=→"Time Elapsed(ms)":i32)
    n853 = case shown="True" "Play" {
      frame False {
      }
      frame True {
        n854 = stacked-sequence {
          frame #0 {
            n855 = Tick Count (ms)() -> (millisecond timer value=→"Start":u32)
          }
          frame #1 {
            n856 = case shown="False" "Input Object Location" {
              frame False {
                # "If Play is pressed, but user input is not, will surround object \n(a circle right now)"
                n857 = local read "Object X"() -> (w415:dbl)
                n858 = local read "bottomry 2"() -> (w417:dbl)
                n859 = local read "toply 2"() -> (w412:dbl)
                n860 = local read "toplx 2"() -> (w425:dbl)
                n861 = local read "Object Y"() -> (w424:dbl)
                n862 = local read "Object X"() -> (w408:dbl)
                n863 = local read "bottomrx 2"() -> (w430:dbl)
                n864 = local read "Object Y"() -> (w429:dbl)
                n865 = Multiply(x=w425, y=1e-07) -> (x*y=w426:dbl)
                n866 = Multiply(x=w415, y=1e-07) -> (x*y=w418:dbl)
                n867 = Multiply(x=w424, y=1e-07) -> (x*y=w427:dbl)
                n868 = Multiply(x=w429, y=1e-07) -> (x*y=w428:dbl)
                n869 = Multiply(x=w417, y=1e-07) -> (x*y=w419:dbl)
                n870 = Multiply(x=w412, y=1e-07) -> (x*y=w413:dbl)
                n871 = Multiply(x=w430, y=1e-07) -> (x*y=w431:dbl)
                n872 = Multiply(x=w408, y=1e-07) -> (x*y=w410:dbl)
                n873 = Build Array(w410, w413) -> (w404:T10)
                n874 = Build Array(w418, w419) -> (w405:T10)
                n875 = Build Array(w431, w428) -> (w406:T10)
                n876 = Build Array(w426, w427) -> (w407:T10)
                n877 = Build Array (concatenate)(w404, w405, w406, w407) -> (w403:T10)
                n878 = local write "NewXYArray"(w403) -> ()
              }
              frame True {
                n879 = local read "distance  bw x and rad"() -> (w433:dbl)
                n880 = local read "distance  bw x and rad"() -> (w436:dbl)
                n881 = local read "Object New Y"() -> (w443:dbl)
                n882 = local read "Object New Y"() -> (w440:dbl)
                n883 = local read "Object New X"() -> (w437:dbl)
                n884 = local read "distance bw y and rad"() -> (w442:dbl)
                n885 = local read "Object New X"() -> (w434:dbl)
                n886 = local read "distance bw y and rad"() -> (w439:dbl)
                n887 = local read "Object New X"() -> (w458:dbl)
                n888 = local read "Object New X"() -> (w468:dbl)
                n889 = Subtract(x=w434, y=w433) -> (x-y=w432:dbl)
                n890 = local read "Object New Y"() -> (w446:dbl)
                n891 = Add(x=w437, y=w436) -> (x+y=w435:dbl)
                n892 = Subtract(x=w443, y=w442) -> (x-y=w441:dbl)
                n893 = Add(x=w440, y=w439) -> (x+y=w438:dbl)
                n894 = local read "Object New Y"() -> (w451:dbl)
                n895 = Multiply(x=w432, y=1e-07) -> (x*y=w448:dbl)
                n896 = Multiply(x=w441, y=1e-07) -> (x*y=w464:dbl)
                n897 = Multiply(x=w468, y=1e-07) -> (x*y=w465:dbl)
                n898 = Multiply(x=w438, y=1e-07) -> (x*y=w455:dbl)
                n899 = Multiply(x=w458, y=1e-07) -> (x*y=w459:dbl)
                n900 = Multiply(x=w435, y=1e-07) -> (x*y=w454:dbl)
                n901 = Multiply(x=w451, y=1e-07) -> (x*y=w450:dbl)
                n902 = Multiply(x=w446, y=1e-07) -> (x*y=w445:dbl)
                n903 = Build Array(w465, w464) -> (w463:T10)
                n904 = Build Array(w459, w455) -> (w462:T10)
                n905 = Build Array(w454, w450) -> (w461:T10)
                n906 = Build Array(w448, w445) -> (w460:T10)
                n907 = Build Array (concatenate)(w463, w462, w461, w460) -> (w444:T10)
                n908 = local write "NewXYArray"(w444) -> ()
              }
            }
            n909 = local write "Max Number of Bubbles 2"("Max Number of Bubbles 2") -> ()
            n910 = local write "LCS"("LCS") -> ()
            n911 = local write "Rates"("Rates") -> ()
            n912 = local write "How Many Frames?"("Number of Planned Sequence Frames 2") -> ()
            "Initiate Creation 2" <- 1.0
          }
          frame #2 {
            n913 = local read "NewXYArray"() -> (w472:dbl[][])
            n914 = Array Size(array=w472) -> (size(s)=w471:i32[])
            n915 = Index Array(array=w471, index=0) -> (element=w469:i32)
            "NewXYArraySize" <- w469
            n916 = for {
              N: w469 -> [w474]
              i -> [w475]
              stop <- w473 stop-if-true
              n917 = stacked-sequence {
                tunnel: w475 -> [w477 _]
                tunnel: w474 -> [w476 _]
                tunnel: [_ w480] -> w473
                frame #0 {
                  n918 = local write "Locked Current Spot"(w477) -> ()
                  n919 = local write "# of Spots"(w476) -> ()
                  n920 = local write "Rates"(1) -> ()
                  n921 = local write "LCS"(0) -> ()
                }
                frame #1 {
                  n922 = local read "Insert"() -> (w480:bool)
                  n923 = local write "Insert"(TRUE) -> ()
                }
              }
            }
          }
        }
      }
    }
    n924 = local read "toplx 2"() -> (w45:dbl)
    n925 = local read "bottomrx 2"() -> (w46:dbl)
    n926 = Subtract(x=w45, y=w46) -> (x-y=w48:dbl)
    n927 = local read "toplx 2"() -> (w50:dbl)
    n928 = Absolute Value(x=w48) -> (abs(x)=w49:dbl)
    n929 = Divide(x=w49, y=2.0) -> (x/y=w37:dbl)
    "distance  bw x and rad" <- w37
    n930 = Add(x=w37, y=w50) -> (x+y=→"Object X":dbl)
    n931 = local write "Object New X"("Object New X") -> ()
    n932 = local write "Object New Y"("Object New Y") -> ()
    n933 = local read "bottomry 2"() -> (w44:dbl)
    n934 = local read "toply 2"() -> (w43:dbl)
    n935 = Subtract(x=w44, y=w43) -> (x-y=w42:dbl)
    n936 = local read "toply 2"() -> (w39:dbl)
    n937 = Absolute Value(x=w42) -> (abs(x)=w41:dbl)
    n938 = Divide(x=w41, y=2.0) -> (x/y=w36:dbl)
    "distance bw y and rad" <- w36
    n939 = Add(x=w36, y=w39) -> (x+y=→"Object Y":dbl)
    n940 = case shown="True" "Lock Current Spot" {
      frame False {
      }
      frame True {
        n941 = global read "red_tweezers_globals.vi" "Spots"() -> (w559:T2[])
        n942 = local read "Current Spot #"() -> (w560:dbl)
        "Locked Current Spot" <- w560
        n943 = Index Array(array=w559, index=w560) -> (element=w561:T2)
        n944 = Unbundle By Name(w561) -> ("Position.x"=→"LCS X":dbl, "Position.y"=→"LCS Y":dbl)
        n945 = local write "LCS"(0) -> ()
      }
    }
    n946 = local read "Rates"() -> (w69:dbl)
    n947 = Equal?(x=w69, y=1.0) -> (x = y?=w67:bool)
    n948 = case shown="True" w67 {
      frame False {
      }
      frame True {
        n949 = stacked-sequence {
          frame #0 {
            n950 = local read "Number of Planned Sequence Frames 2"() -> (w305:dbl)
            n951 = local read "Tab Control"() -> (w306:enum32{"Line", "Arc"})
            n952 = case shown="\"Arc\"" w306 {
              tunnel: w305 -> [w312 w366]
              frame "Arc" {
                w319 = 1e-07 ("x")
                w340 = 2
                n953 = local read "Current Y"() -> (w329:dbl)
                n954 = local read "Current X"() -> (w331:dbl)
                n955 = local read "Center Y"() -> (w330:dbl)
                n956 = local read "Center X"() -> (w332:dbl)
                n957 = Subtract(x=w312, y=1.0) -> (x-y=w311:dbl)
                n958 = expression code="(x/180.0)*pi" "degrees to radians"(180.0) -> (w335:dbl)
                n959 = Subtract(x=w330, y=w329) -> (x-y=→"Original\nD-Y":dbl)
                n960 = Subtract(x=w332, y=w331) -> (x-y=→"Original\nD-X":dbl)
                n961 = local read "Current X"() -> (w309:dbl)
                n962 = Divide(x=w335, y=w311) -> (x/y=→"Degree Rate":dbl)
                n963 = local read "Current Y"() -> (w307:dbl)
                n964 = Less Than 0?(x=w309) -> (x < 0?=w310:bool)
                n965 = case shown="False" w310 {
                  tunnel: w309 -> [_ w363]
                  tunnel: w307 -> [w346 w362]
                  tunnel: w309 -> [_ _]
                  tunnel: w309 -> [w345 _]
                  frame False {
                    n966 = Less Than 0?(x=w346) -> (x < 0?=w344:bool)
                    n967 = case shown="True" w344 {
                      tunnel: w346 -> [w349 w353]
                      tunnel: w345 -> [w348 w352]
                      frame False {
                        n968 = Divide(x=w349, y=w348) -> (x/y=w350:dbl)
                        n969 = Inverse Tangent(1:w350) -> (0:w347:dbl)
                        n970 = local write "Original Theta"(w347) -> ()
                      }
                      frame True {
                        w354 = 2.0  # x
                        n971 = Divide(x=w353, y=w352) -> (x/y=w358:dbl)
                        n972 = Inverse Tangent(1:w358) -> (0:w357:dbl)
                        n973 = Multiply(x=w354, y=3.141592653589793) -> (x*y=w356:dbl)
                        n974 = Add(x=w357, y=w356) -> (x+y=w351:dbl)
                        n975 = local write "Original Theta"(w351) -> ()
                      }
                    }
                  }
                  frame True {
                    n976 = Divide(x=w362, y=w363) -> (x/y=w364:dbl)
                    n977 = Inverse Tangent(1:w364) -> (0:w361:dbl)
                    n978 = Add(x=w361, y=3.141592653589793) -> (x+y=w359:dbl)
                    n979 = local write "Original Theta"(w359) -> ()
                  }
                }
                n980 = local read "ROI-Y"() -> (w317:dbl)
                n981 = local read "ROI-X"() -> (w318:dbl)
                n982 = local read "Current Y"() -> (w342:dbl)
                n983 = local read "Current X"() -> (w338:dbl)
                n984 = Multiply(x=w319, y=w317) -> (x*y=w316:dbl)
                n985 = Multiply(x=w319, y=w318) -> (x*y=w315:dbl)
                n986 = Add(x=w316, y=w342) -> (x+y=w341:dbl)
                n987 = Add(x=w315, y=w338) -> (x+y=w339:dbl)
                n988 = Divide(x=w341, y=w340) -> (x/y=w333:dbl)
                "Center Y" <- w333
                n989 = Divide(x=w339, y=w340) -> (x/y=w334:dbl)
                "Center X" <- w334
                n990 = Build Array(w334, w333) -> (→"Center location":T10)
                n991 = local read "Original\nD-X"() -> (w328:dbl)
                n992 = local read "Original\nD-Y"() -> (w327:dbl)
                n993 = local read "Position"() -> (w322:cluster{"x":dbl, "y":dbl, "z":dbl})
                n994 = Square(x=w328) -> (x^2=w326:dbl)
                n995 = Square(x=w327) -> (x^2=w325:dbl)
                n996 = Unbundle(w322) -> ("x"=→"Current X":dbl, "y"=→"Current Y":dbl)  [unwired: 1 out]
                n997 = Add(x=w326, y=w325) -> (x+y=w324:dbl)
                n998 = Square Root(x=w324) -> (sqrt(x)=→"Original\nRadius":dbl)
              }
              frame "Line" {
                n999 = local read "Max Number of Bubbles 2"() -> (w365:dbl)
                n1000 = for {
                  N: w365 -> [_]
                  tunnel: w366 -> [w368]
                  i -> [w367]
                  n1001 = stacked-sequence {
                    tunnel: w368 -> [_ w386]
                    tunnel: w367 -> [w372 w383]
                    frame #0 {
                      n1002 = local read "NewXYArray"() -> (w378:dbl[][])
                      n1003 = Index Array(array=w378, index (row)=w372) -> (element=w377:dbl[])  [unwired: 1 in]
                      n1004 = Array To Cluster(array=w377) -> (cluster=w376:T30)
                      n1005 = global read "red_tweezers_globals.vi" "Spots"() -> (w373:T2[])
                      n1006 = Unbundle By Name(w376) -> ("NewXYArray[0]"=w375:dbl, "NewXYArray[1]"=w374:dbl)
                      n1007 = Index Array(array=w373, index=w372) -> (element=w371:T2)
                      n1008 = local write "New Y"(w374) -> ()
                      n1009 = local write "New X"(w375) -> ()
                      n1010 = Unbundle By Name(w371) -> ("Position.x"=w370:dbl, "Position.y"=w369:dbl)
                      n1011 = local write "Original X"(w370) -> ()
                      n1012 = local write "Original Y"(w369) -> ()
                    }
                    frame #1 {
                      n1013 = local read "Original X"() -> (w387:dbl)
                      n1014 = local read "Original Y"() -> (w389:dbl)
                      n1015 = Subtract(x=w386, y=1) -> (x-y=w393:dbl)
                      n1016 = local read "New Y"() -> (w390:dbl)
                      n1017 = local read "New X"() -> (w388:dbl)
                      n1018 = Subtract(x=w389, y=w390) -> (x-y=w392:dbl)
                      n1019 = Subtract(x=w387, y=w388) -> (x-y=w391:dbl)
                      n1020 = Divide(x=w392, y=w393) -> (x/y=w381:dbl)
                      "Y Rate" <- w381
                      n1021 = Divide(x=w391, y=w393) -> (x/y=w382:dbl)
                      "X Rate" <- w382
                      n1022 = Bundle(w382, w381) -> (w380:cluster{dbl, dbl})  [unwired: 1 in]
                      n1023 = local read "NewXYRates"() -> (w384:dbl[][])
                      n1024 = Cluster To Array(cluster=w380) -> (array=w379:dbl[])
                      n1025 = Insert Into Array(array=w384, index (row)=w383, new element=w379) -> (w385:dbl[][])  [unwired: 1 in]
                      n1026 = local write "NewXYRates"(w385) -> ()
                    }
                  }
                }
              }
            }
          }
          frame #1 {
            n1027 = local write "Rates"(0) -> ()
          }
        }
      }
    }
    n1028 = case shown="True" "Mark Original Position" {
      frame False {
      }
      frame True {
        w562 = TRUE
        n1029 = local write "Mark Original Position"(FALSE) -> ()
        n1030 = local read "New X"() -> (→"Original X":dbl)
        n1031 = local read "New Y"() -> (→"Original Y":dbl)
        "MOP pressed After" <- w562
        "MOP pressed" <- w562
      }
    }
    n1032 = local read "Sequence Instances"() -> (w125:dbl)
    n1033 = case shown="True" w144 {
      tunnel: w150 -> [_ w628]
      frame False {
      }
      frame True {
        n1034 = global write "red_tweezers_globals_INTERNAL.vi" "Image Overlay (extras from control loop)"(w628) -> ()
      }
    }
    n1035 = local read "Counter"() -> (w124:dbl)
    n1036 = call "red_tweezers_UNDO.vi"("Force Save"=w146, "This change is inconsequential (don't save it)"=w147, "Selection/Group"=w148, "Spots"=w149) -> ()  [unwired: 6 in, 2 out]
    n1037 = call "sync_with_globals.vi"("Selection/Group"=w148, "Spots"=w149) -> ("Selection/Group 2"=w160:T8[], "Spots 2"=w111:T2[])  [unwired: 4 in]
    n1038 = local read "Sequence Storer"() -> (w120:T2[][])
    n1039 = local read "Sequence On?"() -> (w123:bool)
    n1040 = local read "Sequence On?"() -> (w138:bool)
    n1041 = call "SequenceControl.vi"("Sequence On? 2"=w123, "Counter 2"=w124, "Sequence Instances 2"=w125, "Sequence Storer"=w120) -> ("Time per Frame (ms) 2"=w118:dbl, "Sequence Order 2"=w121:dbl, "Reset 2"=w122:bool, "Sequence Storer 2"=w133:T2[][], "Clearance Button 2"=w132:bool, "Manual Edit 2"=w131:bool, "Save State 2"=w130:bool, "Play Sequence 2"=w127:bool, "Bubble ID to Empty 2"=w126:dbl, "Manual Sequence 2"=w128:bool, "Edit Sequence Mode 2"=w129:bool)  [unwired: 1 in]
    n1042 = local write "Play Sequence"(w127) -> ()
    n1043 = local write "Bubble ID to Empty"(w126) -> ()
    n1044 = local write "Manual Sequence"(w128) -> ()
    n1045 = local write "Reset"(w122) -> ()
    n1046 = local write "Edit Sequence Mode"(w129) -> ()
    n1047 = local write "Clearance Button"(w132) -> ()
    n1048 = local write "Sequence Storer"(w133) -> ()
    n1049 = local write "Save State"(w130) -> ()
    n1050 = local write "Manual Edit"(w131) -> ()
    n1051 = Or(x=w138, y="Manual Sequence") -> (x .or. y?=w137:bool)
    n1052 = local write "Time per Frame (ms)"(w118) -> ()
    n1053 = feedback #10() -> (w165:T31)  [unwired: 1 out]
    n1054 = call "Smoothed Frame Rate.vi"("Feedback In"=w165) -> ("Feedback Out"=w164:T31, "Frame Rate"=→"Interface Frame Rate":dbl)  [unwired: 1 in, 4 out]
    n1055 = feedback-in #10(w164) -> ()
    n1056 = local write "Sequence Order"(w121) -> ()
    n1057 = Not(x=w114) -> (.not. x?=w115:bool)
    n1058 = Not(x="Output to SLM") -> (.not. x?=w116:bool)
    n1059 = case shown="True" w137 {
      tunnel: [w598 w603] -> w141
      tunnel: w111 -> [w597 _]
      frame False {
        n1060 = Or(x="Manual Edit", y="Edit Sequence Mode") -> (x .or. y?=w596:bool)
        n1061 = case shown="False" w596 {
          tunnel: w597 -> [w599 _]
          tunnel: [w599 w600] -> w598
          frame False {
          }
          frame True {
            n1062 = local read "Sequence Order"() -> (w601:dbl)
            n1063 = local read "Sequence Storer"() -> (w602:T2[][])
            n1064 = Index Array(array=w602, index (row)=w601) -> (element=w600:T2[])  [unwired: 1 in]
          }
        }
      }
      frame True {
        n1065 = stacked-sequence {
          tunnel: [w605 _] -> w603
          frame #0 {
            n1066 = local read "Counter"() -> (w606:dbl)
            n1067 = local read "Sequence Storer"() -> (w607:T2[][])
            n1068 = Index Array(array=w607, index (row)=w606) -> (element=w605:T2[])  [unwired: 1 in]
            n1069 = Wait (ms)(milliseconds to wait="Time per Frame (ms)") -> ()  [unwired: 1 out]
          }
          frame #1 {
            n1070 = local read "Sequence Instances"() -> (w609:dbl)
            n1071 = local read "Counter"() -> (w612:dbl)
            n1072 = Subtract(x=w609, y=1) -> (x-y=w610:dbl)
            n1073 = Equal?(x=w612, y=w610) -> (x = y?=w611:bool)
            n1074 = case shown="True" w611 {
              frame False {
                n1075 = local read "Counter"() -> (w615:dbl)
                n1076 = Add(x=w615, y=1) -> (x+y=→"Counter":dbl)
              }
              frame True {
                w616 = FALSE
                n1077 = local write "Counter"(0) -> ()
                n1078 = local write "Play Sequence"(w616) -> ()
                n1079 = local write "Sequence On?"(w616) -> ()
              }
            }
          }
        }
      }
    }
    n1080 = case shown="True" "Save State" {
      tunnel: w111 -> [_ w619]
      frame False {
      }
      frame True {
        n1081 = local write "Save State"(FALSE) -> ()
        n1082 = stacked-sequence {
          tunnel: w619 -> [w620 _]
          frame #0 {
            "Spot Storage" <- w620
          }
          frame #1 {
            n1083 = local read "Spot Storage"() -> (w626:T2[])
            n1084 = Replace Array Subset(array="Sequence Storer", new element=w626, index (row)="Sequence Order") -> (w624:T2[][])  [unwired: 1 in]
            n1085 = Array Size(array=w624) -> (size(s)=w623:i32[])
            n1086 = local write "Sequence Storer"(w624) -> ()
            n1087 = Index Array(array=w623, index=0) -> (element=→"Sequence Instances":i32)
          }
        }
      }
    }
    n1088 = case shown="True" "Clearance Button" {
      frame False {
      }
      frame True {
        # "This is the Bubble ID to Empty tool- this \"deletes\" the bubble in a sequence."
        n1089 = local read "Sequence Order"() -> (w589:dbl)
        n1090 = local read "Sequence Storer"() -> (w590:T2[][])
        n1091 = Replace Array Subset(array=w590, new element=T13 {"Position"={"x"=nan, "y"=nan, "z"=nan}, "Intensity"=1.0, "Vortex Charge"=1, "Phase"=1.0, "NA Position"={"x"=0.0, "y"=0.0, "r"=1.0}, "Line Trapping"={"Vector"={"x"=0.0, "y"=0.0, "z"=0.0}, "Phase Gradient"=0.0}, "Amplitude Correction"=0.0} ("Cluster"), index (row)=w589, index (col)="Bubble ID to Empty") -> (w586:T2[][])
        n1092 = local write "Sequence Storer"(w586) -> ()
      }
    }
    n1093 = case shown="True" "Save" {
      frame False {
      }
      frame True {
        n1094 = local read "Sequence Storer"() -> (w555:T2[][])
        n1095 = call "SequenceSaver.vi"("Sequence Storer"=w555) -> ()  [unwired: 10 in, 1 out]
      }
    }
    n1096 = And(x=w116, y=w115) -> (x .and. y?=w119:bool)
    n1097 = case shown="True" "Load" {
      frame False {
      }
      frame True {
        n1098 = call "SequenceSaver.vi"() -> ("Sequence Storer 2"=w554:T2[][])  [unwired: 11 in]
        n1099 = local write "Sequence Storer"(w554) -> ()
      }
    }
    n1100 = local read "Initiate Creation 2"() -> (w72:dbl)
    n1101 = case shown="True" w119 {
      tunnel: w111 -> [w2016 _]
      frame False {
        n1102 = call "UDP Sender generic_2.vi"("Spots"=w2016) -> ()  [unwired: 2 in, 1 out]
      }
      frame True {
      }
    }
    n1103 = case shown="True" "Reset" {
      frame False {
      }
      frame True {
        n1104 = local write "Counter"(0) -> ()
      }
    }
    n1105 = case shown="True" "Add Additional Frames" {
      frame False {
      }
      frame True {
        # "This adds additional frames to the sequence."
        n1106 = for {
          N: "Additional Frames Wanted" -> [_]
          i -> [w568]
          n1107 = local read "Max Number of Bubbles 2"() -> (w572:dbl)
          n1108 = Add(x=1, y=w568) -> (x+y=w569:i32)
          n1109 = Add(x="Frame Location", y=w569) -> (x+y=w570:dbl)
          n1110 = Initialize Array(T13 {"Position"={"x"=nan, "y"=nan, "z"=nan}, "Intensity"=1.0, "Vortex Charge"=1, "Phase"=1.0, "NA Position"={"x"=0.0, "y"=0.0, "r"=1.0}, "Line Trapping"={"Vector"={"x"=0.0, "y"=0.0, "z"=0.0}, "Phase Gradient"=0.0}, "Amplitude Correction"=0.0} ("Cluster"), w572) -> (w573:T32)
          n1111 = local read "Sequence Storer"() -> (w574:T2[][])
          n1112 = Insert Into Array(array=w574, index (row)=w570, new element=w573) -> (w575:T2[][])  [unwired: 1 in]
          n1113 = local write "Sequence Storer"(w575) -> ()
        }
      }
    }
    n1114 = case shown="1" w72 {
      frame 0, Default {
      }
      frame 1 {
        # "This create the array needed for a sequential\narray."
        n1115 = local read "Number of Planned Sequence Frames 2"() -> (w579:dbl)
        n1116 = local read "Max Number of Bubbles 2"() -> (w578:dbl)
        n1117 = for {
          N: w579 -> [_]
          tunnel: w578 -> [w580]
          i -> [w583]
          n1118 = Initialize Array(T13 {"Position"={"x"=nan, "y"=nan, "z"=nan}, "Intensity"=1.0, "Vortex Charge"=1, "Phase"=1.0, "NA Position"={"x"=0.0, "y"=0.0, "r"=1.0}, "Line Trapping"={"Vector"={"x"=0.0, "y"=0.0, "z"=0.0}, "Phase Gradient"=0.0}, "Amplitude Correction"=0.0} ("Cluster"), w580) -> (w581:T32)
          n1119 = local read "Sequence Storer"() -> (w584:T2[][])
          n1120 = Insert Into Array(array=w584, index (row)=w583, new element=w581) -> (w585:T2[][])  [unwired: 1 in]
          n1121 = local write "Sequence Storer"(w585) -> ()
        }
        n1122 = local write "Initiate Creation 2"(0) -> ()
      }
    }
    n1123 = case shown="False" "Play Sequence" {
      frame False {
        n1124 = local write "Sequence On?"(FALSE) -> ()
      }
      frame True {
        "Sequence On?" <- TRUE
      }
    }
    n1125 = local read "Current Spot #"() -> (w94:dbl)
    n1126 = local read "Selection/Group"() -> (w95:T8[])
    n1127 = local read "# of Spots"() -> (w110:dbl)
    n1128 = Not Equal?(x=w94, y=-1) -> (x != y?=w96:bool)
    n1129 = local read "spots selected 2"() -> (w84:i32)
    n1130 = Index Array(array=w95, index=w94) -> (element=w93:T8)
    n1131 = Unbundle By Name(w93) -> ("Selected"=w92:bool)
    n1132 = local read "spots selected"() -> (w85:i32)
    n1133 = Not(x=w92) -> (.not. x?=w91:bool)
    n1134 = And(x=w91, y=w96) -> (x .and. y?=w86:bool)
    n1135 = Less?(x=w85, y=w84) -> (x < y?=w82:bool)
    n1136 = case shown="True" "Insert" {
      tunnel: w111 -> [_ w225]
      tunnel: w110 -> [_ w224]
      frame False {
      }
      frame True {
        n1137 = for {
          N: w224 -> [_]
          tunnel: w225 -> [w227]
          i -> [w226]
          n1138 = stacked-sequence {
            tunnel: w227 -> [w229 w234 _]
            tunnel: w226 -> [_ w230 _]
            frame #0 {
              n1139 = local read "Start at Which Frame?"() -> (→"Num":dbl)
              "Spot Storage 2" <- w229
            }
            frame #1 {
              n1140 = local read "Selection/Group"() -> (w233:T8[])
              n1141 = Index Array(array=w233, index=w230) -> (element=w232:T8)
              n1142 = Unbundle By Name(w232) -> ("Selected"=w231:bool)
              n1143 = case shown="True" w231 {
                tunnel: w234 -> [_ _]
                frame False {
                }
                frame True {
                  n1144 = stacked-sequence {
                    frame #0 {
                      n1145 = case shown="\"Arc\"" "Tab Control" {
                        frame "Arc" {
                          n1146 = local read "How Many Frames?"() -> (w238:dbl)
                          n1147 = Subtract(x=w238, y=1) -> (x-y=w236:dbl)
                          n1148 = for {
                            N: w238 -> [_]
                            tunnel: w236 -> [w240]
                            i -> [w242]
                            # "What is this ^\n\nFor # of sequence\nframes, don't worry\nabout it"
                            # "How to make position x and y?\nIt's called a cluster, inser the new position to Position.x and Position.y"
                            n1149 = Equal?(x=w240, y=w242) -> (x = y?=w241:bool)
                            n1150 = case shown="False" w241 {
                              tunnel: [w261 w273] -> w244
                              tunnel: [w260 w272] -> w243
                              tunnel: w242 -> [w263 _]
                              frame False {
                                # "calculating new position"
                                n1151 = local read "Original Theta"() -> (w269:dbl)
                                n1152 = local read "Degree Rate"() -> (w271:dbl)
                                n1153 = Add(x=w263, y=1.0) -> (x+y=w262:dbl)
                                n1154 = Multiply(x=w271, y=w262) -> (x*y=w270:dbl)
                                n1155 = Add(x=w269, y=w270) -> (x+y=w268:dbl)
                                n1156 = local read "Original\nRadius"() -> (w265:dbl)
                                n1157 = Cosine(x=w268) -> (cos(x)=w267:dbl)
                                n1158 = Sine(x=w268) -> (sin(x)=w266:dbl)
                                n1159 = Multiply(x=w266, y=w265) -> (x*y=w260:dbl)
                                n1160 = Multiply(x=w267, y=w265) -> (x*y=w261:dbl)
                              }
                              frame True {
                                n1161 = global read "red_tweezers_globals.vi" "Spots"() -> (w276:T2[])
                                n1162 = local read "Numeric"() -> (w275:dbl)
                                n1163 = Index Array(array=w276, index=w275) -> (element=w274:T2)
                                n1164 = Unbundle By Name(w274) -> ("Position.x"=w273:dbl, "Position.y"=w272:dbl)
                              }
                            }
                            n1165 = local read "Spot Storage 2"() -> (w259:T2[])
                            n1166 = local read "Numeric"() -> (w258:dbl)
                            n1167 = Index Array(array=w259, index=w258) -> (element=w246:T2)
                            n1168 = local read "Start at Which Frame?"() -> (w239:dbl)
                            "Numeric 4" <- w239
                            n1169 = Bundle By Name(cluster=w246, "Position.x"=w244, "Position.y"=w243) -> (w245:T2)
                            n1170 = local read "How Many Frames?"() -> (w247:dbl)
                            n1171 = Subtract(x=w239, y=w242) -> (x-y=w256:dbl)
                            n1172 = local read "Sequence Storer"() -> (w257:T2[][])
                            n1173 = local read "Numeric"() -> (w252:dbl)
                            n1174 = Add(x=w256, y=w247) -> (x+y=w255:dbl)
                            n1175 = Subtract(x=w255, y=1) -> (x-y=w253:dbl)
                            n1176 = Replace Array Subset(array=w257, new element=w245, index (row)=w253, index (col)=w252) -> (w251:T2[][])
                            n1177 = Array Size(array=w251) -> (size(s)=w250:i32[])
                            n1178 = local write "Sequence Storer"(w251) -> ()
                            n1179 = Index Array(array=w250, index=0) -> (element=w248:i32)
                            n1180 = local write "Sequence Instances"(w248) -> ()
                          }
                        }
                        frame "Line" {
                          # "This is the automatic sequence generator which allows for the creation of the sequence. This calculates the LAST coordinates of each bubble first\nbefore going for the first few coordinates of the sequence."
                          n1181 = local read "How Many Frames?"() -> (w277:dbl)
                          n1182 = for {
                            N: w277 -> [_]
                            i -> [w285]
                            # "For why do we multiply?"
                            n1183 = local read "Spot Storage 2"() -> (w295:T2[])
                            n1184 = local read "Numeric"() -> (w282:dbl)
                            n1185 = local read "NewXYRates"() -> (w283:dbl[][])
                            n1186 = Index Array(array=w283, index (row)=w282, index (col)=1) -> (element=w278:dbl)
                            n1187 = Index Array(array=w283, index (row)=w282, index (col)=0) -> (element=w279:dbl)
                            n1188 = Index Array(array=w295, index=w282) -> (element=w293:T2)
                            n1189 = Unbundle By Name(w293) -> ("Position.x"=w300:dbl, "Position.y"=w298:dbl)
                            n1190 = Multiply(x=w279, y=w285) -> (x*y=w299:dbl)
                            n1191 = Multiply(x=w278, y=w285) -> (x*y=w294:dbl)
                            "probe" <- w294
                            n1192 = Subtract(x=w300, y=w299) -> (x-y=w297:dbl)
                            n1193 = Subtract(x=w298, y=w294) -> (x-y=w296:dbl)
                            n1194 = Bundle By Name(cluster=w293, "Position.x"=w297, "Position.y"=w296) -> (w288:T2)
                            n1195 = local read "Sequence Storer"() -> (w301:T2[][])
                            n1196 = local read "Numeric"() -> (w287:dbl)
                            n1197 = Add(x="Start at Which Frame?", y=w285) -> (x+y=w284:dbl)
                            n1198 = Replace Array Subset(array=w301, new element=w288, index (row)=w284, index (col)=w287) -> (w292:T2[][])
                            n1199 = Array Size(array=w292) -> (size(s)=w291:i32[])
                            n1200 = local write "Sequence Storer"(w292) -> ()
                            n1201 = Index Array(array=w291, index=0) -> (element=w289:i32)
                            n1202 = local write "Sequence Instances"(w289) -> ()
                          }
                        }
                      }
                    }
                    frame #1 {
                      w303 = FALSE
                      n1203 = Tick Count (ms)() -> (millisecond timer value=→"Stop":u32)
                      n1204 = local write "Play Pressed"(w303) -> ()
                      "Insert End" <- w303
                    }
                  }
                }
              }
              "Numeric" <- w230
            }
            frame #2 {
              n1205 = local write "Insert"(FALSE) -> ()
            }
          }
        }
      }
    }
    n1206 = And(x=w82, y=w86) -> (x .and. y?=w87:bool)
    n1207 = case shown="True" w87 {
      frame False {
      }
      frame True {
        n1208 = local read "# of Spots"() -> (w489:dbl)
        n1209 = for {
          N: w489 -> [_]
          i -> [w491]
          stop <- w490 stop-if-true
          n1210 = local read "Selection/Group"() -> (w493:T8[])
          n1211 = Index Array(array=w493, index=w491) -> (element=w492:T8)
          n1212 = Unbundle By Name(w492) -> ("Selected"=w490:bool)
          n1213 = case shown="True" w490 {
            tunnel: w491 -> [_ w495]
            frame False {
            }
            frame True {
              n1214 = local write "Current Spot #"(w495) -> ()
              "Induce check" <- TRUE
            }
          }
        }
      }
    }
    n1215 = local read "spots selected"() -> (w97:i32)
    n1216 = local read "spots selected 2"() -> (w98:i32)
    n1217 = local read "Prev Current Spot"() -> (w106:dbl)
    n1218 = local read "Current Spot #"() -> (w107:dbl)
    n1219 = Not Equal?(x=w107, y=w106) -> (x != y?=w105:bool)
    n1220 = Greater?(x=w98, y=w97) -> (0:w99:bool)
    n1221 = local read "Induce check"() -> (w88:bool)
    n1222 = Or(x=w105, y=w99) -> (x .or. y?=w90:bool)
    n1223 = Or(x=w90, y=w88) -> (x .or. y?=w89:bool)
    n1224 = case shown="True" w89 {
      frame False {
      }
      frame True {
        n1225 = stacked-sequence {
          frame #0 {
            # "A small 100 ms delay is given to provide enough time for the data to be processed properly."
            n1226 = local read "Null array"() -> (w501:dbl[])
            n1227 = local write "What to Check"(w501) -> ()
            n1228 = local write "ID"(w501) -> ()
            n1229 = local read "Current Spot #"() -> (w503:dbl)
            n1230 = local write "Potential Collisions"(0) -> ()
            n1231 = local read "Spot Checker"() -> (w502:T2[])
            n1232 = Index Array(array=w502, index=w503) -> (element=w504:T2)
            n1233 = Wait (ms)(milliseconds to wait=10) -> ()  [unwired: 1 out]
            n1234 = Unbundle By Name(w504) -> ("Position.x"=w498:dbl, "Position.y"=w499:dbl)
            n1235 = local write "Orig Y SC"(w499) -> ()
            n1236 = local write "Orig X SC"(w498) -> ()
            n1237 = local write "Induce check"(FALSE) -> ()
          }
          frame #1 {
            n1238 = local read "# of Spots"() -> (w505:dbl)
            n1239 = for {
              N: w505 -> [_]
              tunnel: w505 -> [w510]
              i -> [w506]
              n1240 = local read "Selection/Group"() -> (w509:T8[])
              n1241 = Index Array(array=w509, index=w506) -> (element=w508:T8)
              n1242 = Unbundle By Name(w508) -> ("Selected"=w507:bool)
              n1243 = case shown="True" w507 {
                tunnel: w510 -> [_ w512]
                tunnel: w506 -> [_ w511]
                frame False {
                }
                frame True {
                  n1244 = for {
                    N: w512 -> [_]
                    tunnel: w511 -> [w513]
                    i -> [w514]
                    # "If the bubble is not selected, find difference of bubble to bubble\nbeing checked"
                    n1245 = local read "Selection/Group"() -> (w518:T8[])
                    n1246 = Index Array(array=w518, index=w514) -> (element=w517:T8)
                    n1247 = Unbundle By Name(w517) -> ("Selected"=w515:bool)
                    n1248 = Not(x=w515) -> (.not. x?=w516:bool)
                    n1249 = case shown="True" w516 {
                      tunnel: w514 -> [_ w522]
                      tunnel: w513 -> [_ w521]
                      tunnel: w513 -> [_ w520]
                      frame False {
                      }
                      frame True {
                        n1250 = local read "Spot Checker"() -> (w539:T2[])
                        n1251 = Index Array(array=w539, index=w522) -> (element=w540:T2)
                        n1252 = Index Array(array=w539, index=w521) -> (element=w538:T2)
                        n1253 = Unbundle By Name(w538) -> ("Position.x"=w535:dbl, "Position.y"=w531:dbl)
                        n1254 = Unbundle By Name(w540) -> ("Position.x"=w532:dbl, "Position.y"=w528:dbl)
                        n1255 = local read "Area+ Buffer"() -> (w519:dbl)
                        n1256 = Subtract(x=w535, y=w519) -> (x-y=w536:dbl)
                        n1257 = Greater Or Equal?(x=w532, y=w536) -> (x >= y?=w537:bool)
                        n1258 = Add(x=w531, y=w519) -> (x+y=w530:dbl)
                        n1259 = Subtract(x=w531, y=w519) -> (x-y=w529:dbl)
                        n1260 = Add(x=w535, y=w519) -> (x+y=w533:dbl)
                        n1261 = Less Or Equal?(x=w528, y=w530) -> (x <= y?=w527:bool)
                        n1262 = Greater Or Equal?(x=w528, y=w529) -> (x >= y?=w526:bool)
                        n1263 = Less Or Equal?(x=w532, y=w533) -> (x <= y?=w534:bool)
                        n1264 = And(x=w537, y=w534) -> (x .and. y?=w524:bool)
                        n1265 = And(x=w527, y=w526) -> (x .and. y?=w525:bool)
                        n1266 = And(x=w524, y=w525) -> (x .and. y?=w523:bool)
                        n1267 = case shown="True" w523 {
                          tunnel: w522 -> [_ _]
                          tunnel: w522 -> [_ w542]
                          tunnel: w520 -> [_ w541]
                          frame False {
                          }
                          frame True {
                            n1268 = stacked-sequence {
                              tunnel: w542 -> [w543 _]
                              tunnel: w541 -> [w544 _]
                              frame #0 {
                                n1269 = local read "Potential Collisions"() -> (w547:dbl)
                                n1270 = local read "What to Check"() -> (w548:dbl[])
                                n1271 = Insert Into Array(array=w548, index=w547, new element=w543) -> (w549:dbl[])
                                n1272 = local read "ID"() -> (w546:dbl[])
                                n1273 = local write "What to Check"(w549) -> ()
                                n1274 = Insert Into Array(array=w546, index=w547, new element=w544) -> (w545:dbl[])
                                n1275 = local write "ID"(w545) -> ()
                              }
                              frame #1 {
                                n1276 = local read "Potential Collisions"() -> (w552:dbl)
                                n1277 = Add(x=w552, y=1) -> (x+y=w550:dbl)
                                n1278 = local write "Potential Collisions"(w550) -> ()
                              }
                            }
                          }
                        }
                      }
                    }
                  }
                }
              }
            }
          }
          frame #2 {
            n1279 = local read "Current Spot #"() -> (w553:dbl)
            n1280 = local write "Prev Current Spot"(w553) -> ()
          }
        }
      }
    }
    n1281 = local read "Buffer Zone"() -> (w103:dbl)
    n1282 = Multiply(x=w103, y=2) -> (x*y=w104:dbl)
    n1283 = Add(x="Area to check", y=w104) -> (x+y=→"Area+ Buffer":dbl)
    n1284 = feedback #11() -> (w76:dbl)  [unwired: 1 in]
    n1285 = Equal?(x=w76, y=10000) -> (x = y?=w77:bool)
    n1286 = call "Elapsed Time"("Reset"=w77) -> ("Elapsed Time (s)"=w75:dbl, "Time has Elapsed"=w80:bool)  [unwired: 11 in, 6 out]
    "Elapsed Time" <- w75
    n1287 = feedback-in #11(w75) -> ()
    n1288 = And(x="On", y=w80) -> (x .and. y?=w81:bool)
    n1289 = case shown="True" w81 {
      frame False {
      }
      frame True {
        n1290 = local read "Position"() -> (w488:cluster{"x":dbl, "y":dbl, "z":dbl})
        n1291 = Unbundle By Name(w488) -> ("x"=→"X Pos every 10 sec":dbl)
      }
    }
    n1292 = case shown="True" "OK Button" {
      frame False {
      }
      frame True {
        n1293 = script code="clear all;\nclc;\n\ng = gigecam('169.254.154.83');\n\ng.PixelFormat= 'BayerGR8'\n\nimg = snapshot(g);\n\nimshow(img);"() -> ()  [unwired: 1 in, 1 out]
      }
    }
    n1294 = case shown="True" "O Button" {
      frame False {
      }
      frame True {
        n1295 = script code="%\n    rslt = Hough1_data(img);\n\n    % Frame translation\n    %- omit this as of now \n    \n    % Control method\n    increment = 10; %assuming the diamiter of the agent around 20 pic \n    \n    %- NewLoc = [x,y] whose unit is px\n    %- update new location based on current location obtained by the camera\n    NewLoc(1)= rslt(1);\n    NewLoc(2)= rslt(2);\n    \n    \n    % Update microrobot location with NewLoc\n    % the single robot would move to oblique downword\n    \n    % wait seconds"() -> ("NewLoc"=w484:dbl[])  [unwired: 1 in, 1 out]
        n1296 = Index Array(array=w484, index=1) -> (element=→"Y":dbl)
        n1297 = Index Array(array=w484, index=0) -> (element=→"X":dbl)
      }
    }
  }
  n1298 = flat-sequence {
    tunnel: w6 -> [w2019]
    tunnel: w5 -> [w2018]
    tunnel: [w2017] -> w3
    frame #0 {
      n1299 = disable-structure shown="\"White Image (stub)\"" {
        disable-tunnel: w2019 -> [_ _ _ _ _ _]
        disable-tunnel: w2018 -> [_ _ w2077 _ _ _]
        disable-tunnel: [_ _ w2076 _ _ _] -> w2017
        frame condition #0 {
          w2021 = u32 10 ("Number of buffers")
          (unwired) FALSE ("background subtraction")
          # "This subdiagram uses the IMAQ drivers, with a pre-allocated ringbuffer for images.  This is the code I use with my Mikrotron MC1362-CL"
          n1300 = call <vilib>:"IMAQ Init.vi"("Interface Name"="img0") -> ("IMAQ Session Out"=w2028:refnum<k11>)  [unwired: 9 in, 1 out]
          n1301 = call <vilib>:"IMAQ Configure List.vi"("Region of interest"="Global ROI (requires restart)", "Number of buffers"=w2021, "Continuous?"=enum16{"One-Shot", "Continuous"}."Continuous", "IMAQ Session In"=w2028) -> ("error out"=w2022:errorcluster, "IMAQ Session Out"=w2024:refnum<k11>)  [unwired: 6 in]
          n1302 = for {
            N: w2021 -> [_]
            tunnel: 0 ("Channel") -> [w2041]
            shift-right: [w2044] -> w2026
            shift-left: w2022 -> [w2040]
            shift-right: [w2043] -> w2025
            shift-left: w2024 -> [w2042]
            i -> [w2039]
            n1303 = Format Into String(format string="mikrotronbuffer%04d", w2039) -> (resulting string=w2037:string)  [unwired: 2 in, 1 out]
            n1304 = call "IMAQ Create"("Image Name"=w2037) -> ("New Image"=w2036:T9)  [unwired: 4 in, 1 out]
            n1305 = call <vilib>:"IMAQ Configure Buffer.vi"("Channel"=w2041, "error in (no error)"=w2040, "Buffer Number"=w2039, "Image In"=w2036, "IMAQ Session In"=w2042) -> ("error out"=w2044:errorcluster, "IMAQ Session Out"=w2043:refnum<k11>)  [unwired: 5 in]
          }
          n1306 = call <vilib>:"IMAQ Start.vi"("error in (no error)"=w2026, "IMAQ Session In"=w2025) -> ("error out"=w2032:errorcluster, "IMAQ Session Out"=w2033:refnum<k11>)  [unwired: 8 in]
          n1307 = call "IMAQ Create"("Image Name"="Red Tweezers live image") -> ("New Image"=w2034:T9)  [unwired: 3 in, 2 out]
          n1308 = while {
            tunnel: w2033 -> [w2052]
            tunnel: w2032 -> [w2051]
            tunnel: w2034 -> [_]
            tunnel: [w2053] -> w2030
            tunnel: [w2046] -> w2031
            i -> [w2048]
            stop <- w2054 stop-if-true
            n1309 = local read "stop"() -> (w2054:bool)
            n1310 = call <vilib>:"IMAQ Extract Buffer.vi"("error in (no error)"=w2051, "Buffer to extract"=w2048, "IMAQ Session In"=w2052) -> ("error out"=w2046:errorcluster, "Image Out"=w2045:T9, "IMAQ Session Out"=w2053:refnum<k11>)  [unwired: 3 in, 3 out]
            n1311 = call "imageQ_camera_hook.vi"("Image"=w2045) -> ()  [unwired: 11 in]
            n1312 = feedback #12() -> (w2049:T31)  [unwired: 1 in]
            n1313 = call "Smoothed Frame Rate.vi"("Feedback In"=w2049) -> ("Feedback Out"=w2050:T31, "Frame Rate"=w2047:dbl)  [unwired: 1 in, 4 out]
            n1314 = feedback-in #12(w2050) -> ()
            n1315 = global write "red_tweezers_globals_INTERNAL_VOLATILE.vi" "Video Frame Rate"(w2047) -> ()
          }
          n1316 = call <vilib>:"IMAQ Close.vi"("error in (no error)"=w2031, "IMAQ Session In"=w2030) -> ()  [unwired: 9 in, 1 out]
        }
        frame condition #1 {
          (unwired) FALSE ("background subtraction")
          # "This subdiagram acquires using the IMAQdx drivers.  This covers most FireWire and GigE cameras (at least the ones supporting the IIDC or GenICam standards)."
          n1317 = call <vilib>:"IMAQdx Open Camera.vi"("Session In"=T7 "dalsaGenie") -> ("error out"=w2057:errorcluster, "Session Out"=w2056:T7)  [unwired: 9 in]
          n1318 = call <vilib>:"IMAQdx Configure Grab.vi"("error in"=w2057, "Session In"=w2056) -> ("error out"=w2058:errorcluster, "Session Out"=w2059:T7)  [unwired: 8 in]
          n1319 = call "IMAQ Create"("Image Name"="Red Tweezers live image") -> ("New Image"=w2062:T9)  [unwired: 3 in, 2 out]
          n1320 = while {
            tunnel: w2059 -> [w2071]
            tunnel: w2058 -> [w2070]
            tunnel: w2062 -> [w2064]
            tunnel: [w2072] -> w2060
            tunnel: [w2066] -> w2061
            stop <- w2073 stop-if-true
            n1321 = local read "stop"() -> (w2073:bool)
            n1322 = call <vilib>:"IMAQdx Grab.vi"("error in"=w2070, "Image In"=w2064, "Session In"=w2071) -> ("error out"=w2066:errorcluster, "Image Out"=w2065:T9, "Session Out"=w2072:T7)  [unwired: 5 in, 1 out]
            n1323 = call "imageQ_camera_hook.vi"("Image"=w2065) -> ()  [unwired: 11 in]
            n1324 = feedback #13() -> (w2068:T31)  [unwired: 1 in]
            n1325 = call "Smoothed Frame Rate.vi"("Feedback In"=w2068) -> ("Feedback Out"=w2069:T31, "Frame Rate"=w2067:dbl)  [unwired: 1 in, 4 out]
            n1326 = feedback-in #13(w2069) -> ()
            n1327 = global write "red_tweezers_globals_INTERNAL_VOLATILE.vi" "Video Frame Rate"(w2067) -> ()
          }
          n1328 = call <vilib>:"IMAQdx Close Camera.vi"("error in"=w2061, "Session In"=w2060) -> ()  [unwired: 9 in, 1 out]
        }
        frame condition #2 {
          # "This subdiagram acquires using the IMAQdx drivers.  This covers most FireWire and GigE cameras (at least the ones supporting the IIDC or GenICam standards)."
          n1329 = call <vilib>:"IMAQdx Open Camera.vi"("Session In"="Camera") -> ("error out"=w2085:errorcluster, "Session Out"=w2084:T7)  [unwired: 9 in]
          n1330 = call <vilib>:"IMAQdx Configure Grab.vi"("error in"=w2085, "Session In"=w2084) -> ("error out"=w2081:errorcluster, "Session Out"=w2082:T7)  [unwired: 8 in]
          n1331 = call "IMAQ Create"("Image Name"="Red Tweezers live image") -> ("New Image"=w2079:T9)  [unwired: 3 in, 2 out]
          n1332 = call "IMAQdx_get_ROI.vi"("Session In"=w2082) -> ("ROI"=w2078:u32[], "Session Out"=w2080:T7)  [unwired: 8 in]
          n1333 = while {
            shift-right: [w2094] -> w2074
            shift-left: w2081 -> [w2095]
            shift-right: [w2091] -> w2075
            shift-left: w2080 -> [w2092]
            tunnel: w2079 -> [w2090]
            tunnel: w2078 -> [w2089]
            tunnel: w2077 -> [w2088]
            tunnel: [w2087] -> w2076
            stop <- w2101 stop-if-true
            n1334 = event shown="[0] Timeout" {
              selector: _ -> [_ _ _]
              dyn-events: _ -> [_ _ _]
              timeout: 0 -> [_ _ _]
              tunnel: w2095 -> [w2108 w2115 w2130]
              tunnel: [w2107 w2115 w2130] -> w2094
              tunnel: w2092 -> [w2106 w2116 w2131]
              tunnel: [w2105 w2116 w2131] -> w2091
              tunnel: w2090 -> [w2104 _ _]
              tunnel: w2089 -> [w2103 _ _]
              tunnel: w2088 -> [_ w2114 w2129]
              event Timeout {
                w2102 = 0  # timeout in ms
                # "Use a timeout of a few hundred ms if you want to acquire just fast enough to update the image- or a timeout of zero to run the camera at full speed."
                # "This VI sends the image to the loop above for display.\nIt's better to do this than to display here, because it separates the camera loop from the front panel a bit, and increases speed without sacrificing responsiveness of the UI.  Of course, using the event structure removes some of those benefits- but it is possible to write a high-performance camera loop with fast particle tracking, and still use this mechanism to display images without slowing down acquisition."
                # "If we're not dealing with other events, acquire from the camera."
                n1335 = event-data() -> ("Time"=w2113:u32)  [unwired: 1 in]
                n1336 = call <vilib>:"IMAQdx Grab.vi"("error in"=w2108, "Image In"=w2104, "Session In"=w2106) -> ("error out"=w2107:errorcluster, "Image Out"=w2110:T9, "Session Out"=w2105:T7)  [unwired: 5 in, 1 out]
                n1337 = call "IMAQ Clear Overlay"("Image"=w2110) -> ("Image Out"=w2109:T9)  [unwired: 9 in, 1 out]
                n1338 = Multiply(x=w2113, y=u32 1000) -> (x*y=w2111:u32)
                n1339 = call "imageQ_camera_hook.vi"("timeout in ms (0=don't wait if there are no requests)"=w2102, "Timestamp/us"=w2111, "ROI"=w2103, "Image"=w2109) -> ()  [unwired: 8 in]
              }
              event "Draw ROI", "Zoom": Value Change {
                # "This changes the current mouse mode on the image, allowing zooming/drawing of ROI (which can be useful if you want to window down a camera for particle tracking)."
                n1340 = event-data() -> ("CtlRef"=w2121:refnum<vi>)  [unwired: 1 in]
                n1341 = control-ref of="Draw ROI"() -> (w2122:refnum<vi>)
                n1342 = Equal?(x=w2122, y=w2121) -> (x = y?=w2120:bool)
                n1343 = case shown="True" w2120 {
                  tunnel: [w2125 w2128] -> w2119
                  tunnel: [TRUE ("stop") FALSE ("stop")] -> w2117
                  tunnel: [FALSE ("Update Indicators?") TRUE ("Update Indicators?")] -> w2118
                  frame False {
                    w2125 = u32 8 items=["Zoom Tool"=8, "Selection Tool"=0, "Pan Tool"=9, "Point Tool"=1, "Line Tool"=2, "Rectangle Tool"=3, "Rotated Rectangle Tool"=12, "Polyline Tool"=10, "Polygon Tool"=5, "Freehand Tool"=11, "Closed Freehand Tool"=6, "Ellipse Tool"=4, "Annulus Tool"=7] ("Current ROI Tool")
                  }
                  frame True {
                    w2128 = u32 3 items=["Zoom Tool"=8, "Selection Tool"=0, "Pan Tool"=9, "Point Tool"=1, "Line Tool"=2, "Rectangle Tool"=3, "Rotated Rectangle Tool"=12, "Polyline Tool"=10, "Polygon Tool"=5, "Freehand Tool"=11, "Closed Freehand Tool"=6, "Ellipse Tool"=4, "Annulus Tool"=7] ("Current ROI Tool")
                  }
                }
                n1344 = local write "Draw ROI"(w2118) -> ()
                n1345 = local write "Zoom"(w2117) -> ()
                n1346 = property on="Property Node" class="ImageControl"(reference=w2114, "Current ROI Tool"=w2119) -> ()  [unwired: 1 in, 2 out]
              }
              event "Zoom to Fit": Value Change {
                # "The various ROI tools are hidden, so the image control resizes nicely as the Red Tweezers window is resized.  The zoom to fit button/mouse mode buttons return some of this functionality."
                n1347 = event-data() -> ("NewVal"=w2132:bool)  [unwired: 1 in]
                n1348 = property on="Property Node" class="ImageControl"(reference=w2129, "Zoom to Fit Mode"=w2132) -> ()  [unwired: 1 in, 2 out]
              }
            }
            n1349 = feedback #14() -> (w2100:T31)  [unwired: 1 in]
            n1350 = call "Smoothed Frame Rate.vi"("Feedback In"=w2100, "Alpha"=0.05) -> ("Feedback Out"=w2099:T31, "Frame Rate"=w2096:dbl)  [unwired: 4 out]
            n1351 = feedback-in #14(w2099) -> ()
            n1352 = global write "red_tweezers_globals_INTERNAL_VOLATILE.vi" "Video Frame Rate"(w2096) -> ()
            n1353 = local read "stop"() -> (w2097:bool)
            n1354 = Unbundle By Name(w2094) -> ("status"=w2087:bool)
            n1355 = Or(x=w2087, y=w2097) -> (x .or. y?=w2101:bool)
          }
          n1356 = call <vilib>:"IMAQdx Close Camera.vi"("error in"=w2074, "Session In"=w2075) -> ()  [unwired: 9 in, 1 out]
        }
        frame condition #3 (active) {
          w2134 = 0 ("element")
          w2136 = 1920 ("dimension size")
          w2135 = 1080 ("dimension size")
          w2137 = T17 0 items=["Grayscale (U8)", "Grayscale (I16)", "Grayscale (SGL)", "Complex (CSG)", "RGB (U32)", "HSL (U32)", "RGB (U64)", "Grayscale (U16)"] ("Image Type")
          (unwired) FALSE ("background subtraction")
          # "This subdiagram generates a blank white image- useful if you don't have a camera"
          n1357 = Build Array(w2134, w2134, w2136, w2135) -> (w2133:i32[])
          n1358 = Initialize Array(u8 255 ("element"), w2135, w2136) -> (w2138:u8[][])
          n1359 = global write "red_tweezers_globals_INTERNAL.vi" "Global ROI"(w2133) -> ()
          n1360 = call "IMAQ Create"("Image Name"="red tweezers camera stub", "Image Type"=w2137) -> ("New Image"=w2139:T9)  [unwired: 2 in, 2 out]
          n1361 = call "IMAQ ArrayToImage"("Image Pixels (U8)"=w2138, "Image"=w2139) -> ("Image Out"=w2142:T9)  [unwired: 8 in, 1 out]
          n1362 = call "IMAQ Create"("Image Name"="Red Tweezers live image") -> ("New Image"=w2143:T9)  [unwired: 3 in, 2 out]
          n1363 = while {
            tunnel: w2142 -> [w2146]
            tunnel: w2143 -> [_]
            stop <- w2150 stop-if-true
            n1364 = local read "stop"() -> (w2150:bool)
            n1365 = Wait Until Next ms Multiple(millisecond multiple=u32 20) -> ()  [unwired: 1 out]
            n1366 = call "imageQ_camera_hook.vi"("Image"=w2146) -> ()  [unwired: 11 in]
            n1367 = feedback #15() -> (w2148:T31)  [unwired: 1 in]
            n1368 = call "Smoothed Frame Rate.vi"("Feedback In"=w2148) -> ("Feedback Out"=w2149:T31, "Frame Rate"=w2147:dbl)  [unwired: 1 in, 4 out]
            n1369 = feedback-in #15(w2149) -> ()
            n1370 = global write "red_tweezers_globals_INTERNAL_VOLATILE.vi" "Video Frame Rate"(w2147) -> ()
          }
        }
        frame condition #4 {
          # "Use this subdiagram if you have an external camera VI which writes to the image queue (using imageQ_camera_hook.vi)"
        }
        frame condition #5 {
          w2151 = path "C:/Users/Tweezer Cube/Desktop/red_tweezers_1_4_rc0/camera_for_rt136.llb/Particle Tracking.vi"  # Path to camera VI
          # "Use this subdiagram if you have an external camera VI which writes to the image queue (using imageQ_camera_hook.vi).  This is the slightly more sophisticated version, which checks that said external VI is running, and runs it if not."
          n1371 = Open VI Reference(vi path=w2151) -> (vi reference=w2152:refnum<vi>, error out=w2154:errorcluster)  [unwired: 5 in]
          n1372 = property class="VI"(reference=w2152) -> ("Path"=w2153:path)  [unwired: 1 in, 2 out]
          n1373 = global write "red_tweezers_globals_INTERNAL_VOLATILE.vi" "Current Camera VI"(w2153) -> ()
          n1374 = property class="VI"(reference=w2152, error in=w2154) -> (reference out=w2159:refnum<vi>, error out=w2158:errorcluster, "Exec.State"=w2156:T33)
          n1375 = Equal?(x=w2156, y=T33."Idle") -> (x = y?=w2160:bool)
          n1376 = case shown="True" w2160 {
            tunnel: w2159 -> [w2164 w2173]
            tunnel: w2158 -> [w2163 w2170]
            tunnel: [w2162 w2169] -> w2155
            tunnel: w2156 -> [w2166 _]
            frame False {
              n1377 = Close Reference(reference=w2164, error in (no error)=w2163) -> (error out=w2162:errorcluster)
              n1378 = Equal?(x=w2166, y=T33."Bad") -> (x = y?=w2165:bool)
              n1379 = case shown="False" w2165 {
                frame False {
                }
                frame True {
                  n1380 = One Button Dialog(message="The external camera VI is not running and cannot be started- it's probably broken or missing.  Check the static/dynamically loaded VI reference in the bottom loop on the block diagram.") -> ()  [unwired: 1 in, 1 out]
                }
              }
            }
            frame True {
              n1381 = invoke class="VI" method="Run VI"(reference=w2173, error in=w2170, "Wait until done"=FALSE ("Wait Until Done"), "Auto Dispose Ref"=TRUE ("Auto Dispose Reference")) -> (error out=w2169:errorcluster)  [unwired: 1 in, 4 out]
            }
          }
          n1382 = call <vilib>:"Simple Error Handler.vi"("error source (\" \")"="External camera VI (see the bottom loop in the block diagram)" ("error source (\" \")"), "error in (no error)"=w2155) -> ()  [unwired: 3 in, 5 out]
        }
      }
    }
  }
  n1383 = while {
    tunnel: w9 -> [w2191]
    shift-right: [w2190] -> w8
    shift-left: w10 -> [w2192]
    shift-right: [w2187] -> _
    shift-left: _ -> [w2180]
    shift-right: [w2186] -> _
    shift-left: _ -> [w2184]
    shift-right: [w2185] -> _
    shift-left: FALSE ("Saving") -> [w2181]
    stop <- w2189 stop-if-true
    w2178 = u32 50 ("millisecond multiple")
    # "Start/stop saving data, if necessary"
    n1384 = Divide(x=u32 1000, y=w2178) -> (x/y=w2176:dbl)
    n1385 = Wait Until Next ms Multiple(millisecond multiple=w2178) -> ()  [unwired: 1 out]
    n1386 = call "imageQ_dequeue.vi"("timeout in ms (-1)"=2000, "Return queue"=w2192, "Image Dst"=w2191) -> ("Timestamp/us"=w2182:u64, "Return queue out"=w2190:refnum<queue>, "Image Dst Out"=w2193:T9, "timed out?"=w2196:bool, "ROI"=w2175:u64[])  [unwired: 4 in]
    n1387 = Not(x=w2196) -> (.not. x?=w2194:bool)
    n1388 = case shown="True" w2194 {
      tunnel: w2193 -> [_ w2230]
      tunnel: w2184 -> [w2223 w2233]
      tunnel: w2181 -> [_ w2227]
      tunnel: [w2223 w2228] -> w2183
      tunnel: w2182 -> [_ w2231]
      tunnel: w2180 -> [w2224 w2232]
      tunnel: [w2224 w2229] -> w2179
      tunnel: w2175 -> [_ w2226]
      frame False {
      }
      frame True {
        n1389 = global read "red_tweezers_globals_INTERNAL.vi" "Image Overlay (extras from control loop)"() -> (w2241:T19[])
        n1390 = case shown="True" w2227 {
          tunnel: w2233 -> [w2242 w2244]
          tunnel: w2232 -> [w2243 w2250]
          tunnel: w2231 -> [_ w2249]
          tunnel: w2230 -> [_ w2248]
          tunnel: [w2243 w2247] -> w2229
          tunnel: [w2242 w2246] -> w2228
          frame False {
          }
          frame True {
            n1391 = call "save_data_save.vi"("Image"=w2248, "Timestamp"=w2249, "Avi Refnum"=w2244, "Data refnum"=w2250) -> ("error out"=w2245:errorcluster, "Avi Refnum (duplicate)"=w2246:T34, "Data refnum (duplicate)"=w2247:refnum<file>)  [unwired: 5 in]
            n1392 = case shown="Error" w2245 {
              selector: w2245 -> [_ w2252]
              frame No Error {
              }
              frame Error {
                n1393 = call <vilib>:"Clear Errors.vi"("error in (no error)"=w2252) -> ()  [unwired: 5 in, 2 out]
                n1394 = local write "Save Video"(FALSE ("Save")) -> ()
              }
            }
          }
        }
        n1395 = global write "red_tweezers_globals_INTERNAL.vi" "Global ROI"(w2226) -> ()
        n1396 = global read "red_tweezers_globals_INTERNAL_VOLATILE.vi" "Tracked Spot Positions (3D)"() -> (w2234:cluster{"x":dbl, "y":dbl, "Z":dbl}[])
        n1397 = global read "red_tweezers_globals.vi" "Selection/Group"() -> (w2240:T8[])
        n1398 = global read "red_tweezers_globals.vi" "Spots"() -> (w2239:T2[])
        n1399 = call "overlay_positions.vi"("Positions"=w2234, "Image"=w2230) -> ("Image 2"=w2236:T9)  [unwired: 9 in]
        n1400 = call "render_overlay_elements.vi"("Image Overlay (extras from control loop)"=w2241, "Image"=w2236) -> ("Image Out"=w2238:T9)  [unwired: 5 in]
        n1401 = call "grid_and_guides.vi"("Operation"=T14."Render on image", "Image"=w2238) -> ("Image Out"=w2225:T9)  [unwired: 9 in]
        n1402 = call "overlay_spots_on_image.vi"("Selection and Groups"=w2240, "Spots"=w2239, "image"=w2225) -> ("Image"=→"Image":T9)  [unwired: 3 in, 1 out]
      }
    }
    n1403 = global read "red_tweezers_globals_INTERNAL_VOLATILE.vi" "Video Frame Rate"() -> (→"Video Frame Rate":dbl)
    n1404 = case shown="True" "Save Video" {
      tunnel: [w2199 w2214] -> w2187
      tunnel: [w2198 w2208] -> w2186
      tunnel: [FALSE ("Saving") w2213] -> w2185
      tunnel: w2181 -> [w2202 w2212]
      tunnel: w2183 -> [w2200 w2211]
      tunnel: w2179 -> [w2201 w2210]
      tunnel: w2176 -> [_ w2209]
      frame False {
        n1405 = case shown="True" w2202 {
          tunnel: w2201 -> [w2204 w2207]
          tunnel: w2200 -> [w2203 w2206]
          tunnel: [w2204 _] -> w2199
          tunnel: [w2203 _] -> w2198
          frame False {
          }
          frame True {
            n1406 = local write "Save Video"(FALSE ("Save")) -> ()
            n1407 = call "save_data_stop.vi"("Avi Refnum"=w2206, "Data refnum"=w2207) -> ()  [unwired: 10 in]
          }
        }
      }
      frame True {
        n1408 = case shown="False" w2212 {
          selector: w2212 -> [_ w2222]
          tunnel: [w2219 w2220] -> w2214
          tunnel: [w2218 w2221] -> w2208
          tunnel: [w2215 w2222] -> w2213
          tunnel: w2211 -> [_ w2221]
          tunnel: w2210 -> [_ w2220]
          tunnel: w2209 -> [w2217 _]
          frame False {
            n1409 = call "save_data_start.vi"("Save Video"=TRUE, "Frames Per Second"=w2217) -> ("Saving"=w2215:bool, "Avi Refnum"=w2218:T34, "Data Refnum"=w2219:refnum<file>)  [unwired: 3 in]
            n1410 = local write "Save Video"(w2215) -> ()
          }
          frame True {
          }
        }
      }
    }
    n1411 = local read "stop"() -> (w2189:bool)
  }
  n1412 = Release Queue(queue=w8) -> ()  [unwired: 2 in, 3 out]
  n1413 = case shown="True" w3 {
    frame False {
    }
    frame True {
      n1414 = One Button Dialog(message="Warning: there was a camera error.  You may need to restart Red Tweezers.") -> ()  [unwired: 1 in, 1 out]
    }
  }
  n1415 = flat-sequence {
    tunnel: w18 -> [w2258]
    tunnel: w17 -> [_]
    frame #0 {
      # "This autosaves when we stop.  The sequence structures are necessary so that:\n1. loading settings doesn't stop the VI\n2. plugins are still open (and hence saved) when we save settings"
      n1416 = local read "Plugins"() -> (w2261:T4)
      n1417 = global read "red_tweezers_globals_INTERNAL_VOLATILE.vi" "Current Settings File"() -> (w2255:path)
      n1418 = global read "red_tweezers_globals_INTERNAL_VOLATILE.vi" "Save Settings On Exit"() -> (w2254:bool)
      n1419 = flat-sequence {
        tunnel: w2258 -> [w2264]
        tunnel: [w2264] -> w2257
        frame #0 {
          n1420 = local write "stop"(FALSE ("STOP")) -> ()
        }
      }
      n1421 = case shown="True" w2254 {
        tunnel: w2255 -> [_ w2269]
        tunnel: w2257 -> [w2266 w2267]
        tunnel: [w2266 w2267] -> w2256
        frame False {
        }
        frame True {
          n1422 = Path To String(path=w2269) -> (string=w2268:string)
          n1423 = call "settings_save_to_file.vi"("XML File Path"=w2269) -> ()  [unwired: 11 in]
          n1424 = call "settings_filename_to_registry.vi"("Last Used Settings File"=w2268) -> ()  [unwired: 11 in]
        }
      }
      n1425 = flat-sequence {
        tunnel: w2256 -> [w2262]
        tunnel: [w2262] -> _
        frame #0 {
          n1426 = local write "stop"(TRUE ("STOP")) -> ()
        }
      }
      n1427 = control-ref of="Plugin Pnl"() -> (w2259:refnum<vi>)
      n1428 = control-ref of="Plugin:"() -> (w2260:refnum<vi>)
      n1429 = call "plugins_unload.vi"("error in (no error)"=w2256, "Plugins"=w2261, "Sub Panel"=w2259, "Plugin Chooser"=w2260) -> ()  [unwired: 2 in, 2 out]
    }
  }
